vi "Project Program.vi"() -> ()   [LabVIEW 2023]
uses:
  <vilib>/Utility/file.llb/Write Delimited Spreadsheet (string).vi
  <vilib>/Utility/file.llb/Write Delimited Spreadsheet (DBL).vi
  <vilib>/express/express arith-compare/Formula/XNode/ExpressFormulaBlockNode.xnode
panel:
  out "Temp":dbl=4.0
  out "IG Array.":dbl[](array[numeric])=[-6.82e-13, -5e-13, -4.42e-13, -8.34e-13, -4.21e-13, -3.68e-13, -5.57e-13, -6.42e-13, -4.64e-13, -4e-13, -6.61e-13, -7.43e-13, -3.88e-13, -2.58e-13, -5.2e-13, -3.59e-13, -5.4e-13, -3.47e-13, -7.65e-13, -4.69e-13, -3.96e-13, -4.05e-13, -9.33e-13, -5.96e-13, -7.48e-13, -9.11e-13, -8.06e-13, -6.45e-13, -4.48e-13, -5.19e-13, -7.58e-13, -7.76e-13, -5.16e-13, -3.9e-13, -3.24e-13, -6.43e-13, -6.17e-13, -6.27e-13, -4.35e-13, -4.04e-13, -5.04e-13, -8.21e-13, -4.73e-13, -4.57e-13, -2.88e-13, -5.66e-13, -4.46e-13, -7.34e-13, -3.11e-13, -5.05e-13, -6.99e-13, -8.36e-13, -7.42e-13, -5.52e-13, -5.7e-13, -4.36e-13, -4.75e-13, -7.06e-13, -7.55e-13, -6.53e-13, -6.56e-13, -4.28e-13, -7.24e-13, -6.36e-13, -4.42e-13, -5.4e-13, -9.54e-13, -3.54e-13, -3.44e-13, -5.99e-13, -4e-13, -6.34e-13, -4.03e-13, -8.94e-13, -6.36e-13, -7.24e-13, -4.01e-13, -5.45e-13, -8.2e-13, -6.39e-13, -7.02e-13, -7.71e-13, -2.97e-13, -2.58e-13, -2.32e-13, -4.29e-13, -2.53e-13, -6.84e-13, -2.11e-13, -3.25e-13, -7.94e-13, -8.62e-13, -7.69e-13, -3.49e-13, -7.07e-13, -9.35e-13, -7.59e-13, -8.18e-13, -1.75e-13, -5.32e-13, -6.85e-13, -6.03e-13, -5.71e-13, -3.91e-13, -3.83e-13, -5.11e-13, -6.19e-13, -8.05e-13, -5.87e-13, -1.199e-12, -1.69e-13, -6.21e-13, -7.91e-13, -7.88e-13, -8.19e-13, -2.8e-13, -6e-13, -2.05e-13, -7.35e-13, -9.14e-13, -5.56e-13, -6.15e-13, -4.42e-13, -3.57e-13, -6.11e-13, -6.95e-13, -3.19e-13, -3.43e-13, -1.41e-13, -6.66e-13, -8.3e-13, -2.95e-13, -2.83e-13, -3.68e-13, -5.57e-13, -6.58e-13, -9.05e-13, -5.9e-13, -3.75e-13, -5.67e-13, 6.3e-14, -6.42e-13, -5.47e-13, -5.51e-13, -2.83e-13, -2.68e-13, -1.89e-13, -4.14e-13, -1.48e-13, -2.35e-13, -5.91e-13, -4.54e-13, -3.95e-13, -1.6e-13, -3.92e-13, -2.8e-13, -5.4e-13, -5.74e-13, -4.24e-13, -1.97e-13, -3.02e-13, -7.59e-13, -3.84e-13, -3.12e-13, -1.53e-13, -5e-13, -2.01e-13, -1.93e-13, -6.54e-13, -7.73e-13, -4.32e-13, -4.13e-13, -5.04e-13, -7.92e-13, -5.26e-13, -7.05e-13, -1.48e-13, -4.35e-13, -5.34e-13, -6.1e-13, -7.07e-13, -5.12e-13, -2.05e-13, -4.81e-13, -5.25e-13, -5.59e-13, -6.02e-13, -6.46e-13, -2.85e-13, -8.37e-13, -5.61e-13, -7.06e-13, -5.7e-13, -6.64e-13, -4.13e-13, -5.68e-13, -3.11e-13, -1.84e-13, -4.02e-13, -7.21e-13, -5.2e-13, 3.29e-13, 2.34e-13, -2.45e-13, -4.14e-13, -3.81e-13, -4.92e-13, -5.75e-13, -2.57e-13, -5.26e-13, -2.99e-13, 4e-15, -2.53e-13, -1.47e-13, -2.6e-14, -4.26e-13, -3.63e-13, -3.29e-13, -5.5e-14, -4.05e-13, -2.06e-13, -1.03e-13, -2.8e-14, -1.05e-13, -2.6e-13, -5.99e-13, 9.7e-14, -4.2e-14, -2.06e-13, -2e-13, -4.16e-13, -2.51e-13, -4e-15, -1.93e-13, -1.86e-13, -5.89e-13, -1.7e-14, -3.82e-13, -3.01e-13, -2.5e-13, -1.57e-13, -8.7e-14, -1.97e-13, -4.72e-13, -2e-15, -6.68e-13, -2.31e-13, -1.02e-13, -4.17e-13, -5.68e-13, -1.14e-13, -4.6e-13, -4.91e-13, -4.63e-13, -2.12e-13, -1.35e-13, -6.95e-13, -1.07e-13, -6.8e-14, -2.6e-13, -6.72e-13, -3.61e-13, -2.45e-13, -1.11e-13, -3.42e-13, -2.84e-13, -1.79e-13, -6.88e-13, -4.74e-13, -5.54e-13, -1.4e-14, -1.15e-13, 3.8e-14, -1.88e-13, -4.68e-13, -1.75e-13, -4.27e-13, -6.58e-13, -3.4e-13, -4.2e-14, -2.68e-13, -6.2e-14, -5.96e-13, -1.68e-13, -4.1e-14, -9.4e-14, -2.8e-13, -3.81e-13, -2.24e-13, -2.86e-13, -4.53e-13, -5.21e-13, -6e-14, -4.08e-13, -2.43e-13, -4.3e-13, -7.7e-14, -3.7e-14, -5.15e-13, -3.27e-13, -3.92e-13, 4.1e-14, 1e-13, -4.77e-13, 1.23e-13, -1.54e-13, 5e-15, -4.27e-13, -5.34e-13, -6.01e-13, -2.12e-13, 3.66e-13, -9.7e-14, -3.61e-13, -1.82e-13, -1.01e-13, -5e-15, -4.18e-13, -3.18e-13, -3.43e-13, -2.39e-13, -4.5e-14, -2e-14, -3.4e-13, -2.26e-13, -7.2e-14, -1.1e-13, 1.21e-13, -1.32e-13, -2.78e-13, -2.48e-13, -1.78e-13, 4e-14, -2.05e-13, -2.36e-13, -2.02e-13, -9.2e-14, -2.21e-13, -5.1e-14, -4.32e-13, -1.25e-13, -2.8e-13, -2.2e-13, -3.37e-13, -2.31e-13, -7.8e-14, -2.37e-13, -4.72e-13, 4.3e-14, -7.2e-14, 5.4e-14, 6.6e-14, -4.5e-13, -1.78e-13, -2.78e-13, -1.67e-13, -3.97e-13, -9e-14, -7.2e-14, -4.35e-13, -1.42e-13, -2.21e-13, -2.98e-13, -8.3e-14, -1.71e-13, -3.7e-13, -2.32e-13, -3.63e-13, -3.13e-13, -2.81e-13, -5e-15, -1.9e-13, -3.68e-13, -2.52e-13, -6.7e-14, -1.79e-13, -3e-14, 1.81e-13, -1.51e-13, 1.6e-14, -7e-14, -2.77e-13, -2e-13, -2.96e-13, 1.24e-13, 8.3e-14, -1.71e-13, -4.7e-14, -2.69e-13, 4e-14, -1.82e-13, -3.15e-13, -4.22e-13, -1.56e-13, -3.44e-13, -2.46e-13, -3.44e-13, -3.79e-13, -3.57e-13, -1.4e-14, 5.4e-14, -1.02e-13, 5.84e-13, -1.7e-14, 4e-15, -2.38e-13, -1.91e-13, -7.6e-14, 1.88e-13, 5.3e-14, 1.06e-13, -8.1e-14, 3.29e-13, 7.4e-14, 2.3e-14, 8.1e-14, -5.2e-14, 1.75e-13, -1.05e-13, -1.62e-13, -1.52e-13, -1.37e-13, 2.83e-13, -2.01e-13, 1.55e-13, -2.28e-13, -9e-14, -1.08e-13, -2.68e-13, -7.6e-14, 6.4e-14, 4.9e-14, -1.12e-13, -9.3e-14, 2.9e-13, 2e-13, 3.19e-13, 1.24e-13, 1.35e-13, -1.31e-13, -1.18e-13, 0.0, 3.9e-14, 1.96e-13, -2.89e-13, 7.3e-14, 5.7e-14, 1.58e-13, -1.82e-13, -6.4e-14, -2.97e-13, -3.8e-14, 3.21e-13, 1.44e-13, 3.3e-14, -1.25e-13, -1.78e-13, 2.63e-13, 1.3e-13, 1.5e-14, 7.4e-14, 1.04e-13, 7e-14, 6.7e-14, -1.85e-13, 7.4e-14, 2.66e-13, 3.1e-14, 1.27e-13, -2.9e-14, -1.63e-13, 3.25e-13, 2.92e-13, 4.5e-14, -1.53e-13, 2.76e-13, 2.64e-13, -1.45e-13, -1.78e-13, 1.8e-14, 1.59e-13, 2.41e-13, -2.25e-13, 2.67e-13, -1.4e-14, 4.3e-14, 1.49e-13, -1.23e-13, -3.61e-13, -7.8e-14, 4.8e-14, 1.85e-13, -3.45e-13, 1.58e-13, -3.05e-13, 8.2e-14, 1.84e-13, 6.8e-14, -1.82e-13, 1.04e-13, -1.64e-13, 8.5e-14, -1.8e-13, 9.8e-14, -5e-14, 2.3e-14, -2.07e-13, -9.1e-14, -1.71e-13, -1.3e-14, 6.2e-14, 1.04e-13, -1.34e-13, 9.7e-14, 9.8e-14, -4.4e-14, 2.74e-13, -1.38e-13, -1.16e-13, 2.6e-14, -1.46e-13, -1.14e-13, -5.3e-14, 3.2e-14, 1.7e-14, 2.35e-13, 2.64e-13, -1.7e-14, 5.9e-14, -2.23e-13, -2.5e-14, 6e-14, 1.19e-13, 1.61e-13, 6.3e-14, 2.59e-13, 1.94e-13, 2.47e-13, 1.37e-13, -3.06e-13, -2.38e-13, 2.05e-13, -9.9e-14, 1.1e-14, 1.48e-13, 5.8e-14, 4.4e-14, -1.4e-13, 2.7e-14, -3.39e-13, -2.75e-13, -2.58e-13, -3.37e-13, -7.4e-14, 2.24e-13, 1.9e-14, 3e-14, 2.66e-13, 2.16e-13, 1.33e-13, 6.4e-14, -9.8e-14, -2.48e-13, 1.89e-13, 2.8e-13, 1.88e-13, -2.83e-13, -1.29e-13, -6.8e-14, -3.9e-14, -3e-14, 3.4e-14, 2.08e-13, 2.48e-13, -2.29e-13, -3.13e-13, 9.9e-14, 1.1e-14, 1.71e-13, -1.38e-13, -5.1e-14, 1.75e-13, 1.46e-13, 1.97e-13, -1.43e-13, -8.2e-14, -1.7e-13, 4.1e-14, -1.1e-14, 2.3e-14, -5e-14, -1.42e-13, 3e-15, -2.88e-13, 3.02e-13, -2.4e-14, 2.99e-13, 2.82e-13, 4.16e-13, -1e-14, 6.67e-13, 2e-15, -9.7e-14, 5.35e-13, 3.82e-13, 6.95e-13, 2e-14, 9.2e-14, -1.6e-14, 5.21e-13, 4.68e-13, 1.51e-13, 2.8e-14, 2.17e-13, 3.9e-14, 4.61e-13, 5.25e-13, 2.57e-13, 1.68e-13, 3.19e-13, 1.92e-13, -4e-14, 2.56e-13, 4.05e-13, 1.19e-13, 4.26e-13, 4.39e-13, 4.51e-13, 4.5e-14, 3.61e-13, 2.33e-13, 2.6e-14, 2.97e-13, 1.83e-13, 2.1e-14, 3.82e-13, -4.9e-14, 1.53e-13, -7.1e-14, 5.3e-13, 3.78e-13, -5.1e-14, 3.25e-13, 1.52e-13, 1.09e-13, 1.16e-13, 4.7e-13, 2.93e-13, 3.92e-13, -1.33e-13, 3.44e-13, 4.93e-13, 9.6e-14, -1.5e-14, 1.22e-13, 7.8e-14, 3.6e-13, 5.5e-14, 4.16e-13, 3.8e-14, 2.65e-13, 6.14e-13, 3.3e-13, 5.13e-13, 3.59e-13, 6.7e-14, 5.2e-14, 5.62e-13, 5.22e-13, -7.5e-14, -2.4e-14, 2.24e-13, 3.88e-13, 9e-15, 5.14e-13, -2.2e-14, 8e-14, -6e-15, 4.51e-13, 2.81e-13, -1.61e-13, 1.89e-13, -9e-15, 4.4e-13, 1.46e-13, 2.23e-13, 5.7e-14, 6.28e-13, 3.3e-13, 3.9e-14, 1.08e-13, 4.48e-13, -4.6e-14, 3.47e-13, 1.91e-13, 4.28e-13, 8.8e-14, 4.49e-13, 3.93e-13, 3.5e-13, 3.79e-13, -1e-15, 5e-13, 3.85e-13, -1.2e-14, 4.47e-13, 5.7e-14, 4.27e-13, 5.31e-13, 4.09e-13, 4.53e-13, 9.7e-14, 8e-14, -1.24e-13, 3.3e-13, -9e-15, 2.4e-13, 3.95e-13, 2.18e-13, 3.31e-13, 1.09e-13, 4.33e-13, 8.7e-14, 2.95e-13, 3.41e-13, -1.28e-13, -7.1e-14, 1.058e-12, 3.33e-13, 2.88e-13, -3.6e-14, 2.85e-13, 3.72e-13, -2.5e-14, 4.76e-13, 2.36e-13, 4.69e-13, 3.91e-13, 7.7e-14, 2.27e-13, 8.4e-14, 4.01e-13, 3.55e-13, 2.51e-13, -1.57e-13, 4.06e-13, 3.2e-13, 3.88e-13, 1.74e-13, 4.69e-13, -1.39e-13, 1.3e-14, 4.32e-13, 3.7e-14, 4.77e-13, -2.19e-13, 2.78e-13, 9.1e-14, -5.2e-14, -7.8e-14, 4.01e-13, 5.8e-14, 3.88e-13, 3.37e-13, 2.64e-13, 4.82e-13, 1.07e-13, 4.48e-13, -9.7e-14, 1.21e-13, 3.87e-13, 2.38e-13, 2.76e-13, 4.55e-13, 1.38e-13, 3.06e-13, 1.53e-13, 2.4e-14, 2.9e-13, 1.5e-13, 4.51e-13, 2.21e-13, -1e-15, -5e-14, 2.12e-13, 3.6e-13, 6.9e-14, 2.66e-13, 3.83e-13, -5e-15, 1.39e-13, 1.24e-13, 2.55e-13, 3.51e-13, 1.23e-13, 3.45e-13, 1.29e-13, 1.58e-13, 2.38e-13, 1.23e-13, 4.27e-13, 2.43e-13, 9e-15, 8.6e-14, 7.38e-13, 5.06e-13, 4.28e-13, 7.03e-13, 6.12e-13, 1.47e-13, 1.8e-13, 3.82e-13, 2.45e-13, 2.26e-13, -1.47e-13, 6.06e-13, 2.23e-13, 5.36e-13, 3.34e-13, 3.8e-14, 5.08e-13, 2.49e-13, 2.5e-14, 2.81e-13, 3.98e-13, 2.51e-13, 3.48e-13, 5.39e-13, 6e-13, 3.9e-13, 2.45e-13, 4.17e-13, 6.93e-13, 2.32e-13, 2.78e-13, 6.19e-13, 4.87e-13, 3.68e-13, 6.8e-13, 1.81e-13, 1.82e-13, 3.63e-13, 1.46e-13, 4.6e-13, 4.01e-13, 6.71e-13, 5.98e-13, 4.98e-13, 3.95e-13, 2.33e-13, 4.23e-13, 1.76e-13, 1.79e-13, 4.5e-13, 5.38e-13, 1.06e-13, 4.37e-13, 3.52e-13, 2.38e-13, 5.36e-13, 1.69e-13, 2.1e-13, 6.3e-14, 1.06e-13, 3.98e-13, 1.45e-13, 1.69e-13, 3.27e-13, 6.04e-13, 2.29e-13, 6.07e-13, 4.02e-13, 3.86e-13, 2.03e-13, 6.1e-14, 1.34e-13, 5.67e-13, 3.62e-13, 1.01e-13, 4.68e-13, 6.14e-13, 1.67e-13, 2.98e-13, 2.57e-13, 3.43e-13, 5.74e-13, 1.14e-13, 3.19e-13, 2.06e-13, 4.41e-13, 4.75e-13, 5.9e-14, 1.61e-13, 4.51e-13, 4.81e-13, 4.93e-13, 1.25e-13, 5.25e-13, 2.43e-13, 3.1e-14, 5.47e-13, 5.5e-13, 3.22e-13, 2.07e-13, 1.09e-13, 2.1e-13, 5.02e-13, 1.8e-13, 7.39e-13, 7.08e-13, 6.59e-13, 1.48e-13, 6.28e-13, 6.14e-13, 4.39e-13, 4.18e-13, 4.09e-13, 3.93e-13, -4e-14, 5.1e-13, 3.35e-13, 6.31e-13, 3.03e-13, 6.7e-13, 2.6e-13, 2.84e-13, -6.37e-13, 7.55e-13, 4.6e-13, 6.32e-13, 4.21e-13, 4.58e-13, 4.74e-13, 6.53e-13, 2.34e-13, 4.7e-13, 4.8e-14, 3.43e-13, 5.53e-13, 4.41e-13, 3.05e-13, 3.93e-13, 5.99e-13, 5.14e-13, 4.48e-13, 6.15e-13, 5.84e-13, 8.5e-14, 1.12e-13, 8.7e-14, 4.24e-13, 4.25e-13, 1.44e-13, 1.13e-13, 6.66e-13, 3.59e-13, 4.49e-13, 4.12e-13, 4.91e-13, -9.1e-14, -1.03e-13, -1.45e-13, 3.54e-13, 3.62e-13, 2.3e-14, 1.96e-13, 8.67e-13, 1.45e-13, 4.61e-13, 4.26e-13, 3.17e-13, 5.2e-13, 1.48e-13, 2.17e-13, 5.61e-13, 5.29e-13, 7.6e-14, 3.63e-13, 1.38e-13, 8.7e-14, 9.4e-14, 1.53e-13, 2.13e-13, 1.67e-13, 5.7e-14, 4.7e-13, 6.26e-13, 2.01e-13, 4.63e-13, 5.33e-13, 5.61e-13, 2.93e-13, 3.24e-13, 6.8e-14, 3.09e-13, 1.24e-13, 4.98e-13, 3.88e-13, 1.31e-13, 5.47e-13, 6.1e-14, 4.6e-13, 1.77e-13, 4.94e-13, 3.46e-13]
  out "IS Array.":dbl[](array[numeric])=[1.45e-12, 5e-14, -2.1e-13, -2.86e-12, 9.3e-13, 7.8e-13, -9.4e-13, -3e-14, -1.04e-12, 1.2e-13, -6.7e-13, -7.7e-13, 4.2e-13, 5.3e-13, 1.5e-13, -1e-14, 3.9e-13, 5.4e-13, -2e-14, 1.2e-13, -5e-13, 2.4e-13, -3.6e-13, -3e-13, 7.3e-13, -5.6e-13, -9e-14, 3e-13, 3.7e-13, -1.3e-13, 4.6e-13, 4.7e-13, -1.03e-12, 2e-13, 1.4e-13, 5e-14, 4.3e-13, 5e-14, 6e-14, 3.6e-13, 9e-14, -4.6e-13, -7e-14, -5.5e-13, 2.5e-13, 2.3e-13, 3.1e-13, 2.9e-13, 4.1e-13, -9e-14, -5e-14, -1.17e-12, 1.8e-13, 1.5e-13, -5.4e-13, 1.2e-13, 1e-14, -2.7e-13, -5e-13, 1.8e-13, -7.2e-13, -7.6e-13, 3.9e-13, -1.03e-12, -4.8e-13, -5.5e-13, -1.14e-12, -4.4e-13, -7.3e-13, -1.5e-12, -1.03e-12, -1.43e-12, -1.35e-12, -1.04e-12, -1.06e-12, -1.12e-12, -1.2e-12, -4e-13, -3.8e-13, -5.7e-13, 4.8e-13, -3e-14, 3.5e-13, 2e-14, -2.4e-13, 1.3e-13, 4.9e-13, -5.3e-13, 5.2e-13, -1e-13, 3e-13, -8.4e-13, -7.5e-13, -2.4e-13, 3.1e-13, -1.29e-12, -1.37e-12, 4.6e-13, 2.8e-13, 1.9e-13, 2e-13, -6.5e-13, -1.09e-12, -1.12e-12, -1.2e-12, -8.9e-13, -1.76e-12, -1.28e-12, -1.43e-12, -3.13e-12, 3.8e-13, -1.67e-12, -1.88e-12, -1.91e-12, -2.11e-12, -1.44e-12, -2.2e-12, -1.79e-12, -1.62e-12, -1.01e-12, -1.69e-12, -2.03e-12, -8.3e-13, -1.36e-12, -1.41e-12, -1.72e-12, -1.97e-12, -2.05e-12, -1.01e-12, -2.14e-12, -2.65e-12, -1.98e-12, -2.07e-12, -9.2e-13, -1.45e-12, -2.15e-12, -1.33e-12, -1.51e-12, -7.2e-13, -1.03e-12, -5.9e-13, -2.3e-13, -7e-13, -1.83e-12, -1.13e-12, -1.42e-12, -6.9e-13, -1.17e-12, -1.28e-12, -1.22e-12, -9.1e-13, -1.49e-12, -1.2e-12, -1e-12, -1.24e-12, -1.27e-12, -1.77e-12, -1.27e-12, -1.71e-12, -2.68e-12, -2.83e-12, -2.35e-12, -2.67e-12, -1.1e-12, -1.49e-12, -2.12e-12, -2.13e-12, -3.07e-12, -2.63e-12, -3.09e-12, -2.87e-12, -2.45e-12, -1.91e-12, -2.45e-12, -2e-12, -1.09e-12, -1.32e-12, -1.8e-12, -8.9e-13, -2.76e-12, -1.52e-12, -2e-12, -1.19e-12, -2.22e-12, -1.11e-12, -2.47e-12, -1.74e-12, -2.4e-12, -2.69e-12, -2.77e-12, -1.03e-12, -1.99e-12, -1.61e-12, -2.42e-12, -1.35e-12, -2.7e-12, -1.49e-12, -1.34e-12, -1.62e-12, -1.27e-12, -2.73e-12, 2.73e-12, 1.57e-12, 6e-13, -1.7e-13, -1.25e-12, -1.8e-13, -1.53e-12, -1.17e-12, -1.52e-12, -1.32e-12, -3.7e-13, -1.58e-12, -8.7e-13, -2.08e-12, -1.41e-12, -4.6e-13, -9.8e-13, 2e-14, -3.7e-13, -1.21e-12, -2.14e-12, -9.2e-13, -1.96e-12, -6.6e-13, -2.27e-12, -1.8e-12, -5.2e-13, -3.9e-13, -6.2e-13, -5.1e-13, -1.7e-12, -6.1e-13, -1.35e-12, -1.68e-12, -1.87e-12, -1.02e-12, -1.17e-12, -1.43e-12, -1.5e-13, -2.05e-12, -1.61e-12, -8.4e-13, -1.7e-13, -1.1e-12, -2.12e-12, -1.15e-12, -2.03e-12, -1.05e-12, 3.6e-13, -1.4e-12, -5.7e-13, -4.3e-13, -9.1e-13, -1.05e-12, -1.2e-12, -1.54e-12, -1.47e-12, -2.12e-12, -2.02e-12, -1.78e-12, -1.94e-12, -1.49e-12, -6.8e-13, -1.76e-12, -1.68e-12, -1.74e-12, -2.18e-12, -1.77e-12, -1.99e-12, -1.01e-12, -9e-13, -1.56e-12, -1.66e-12, -8.2e-13, -1.85e-12, -1.71e-12, -2.03e-12, -1.81e-12, -1.08e-12, -1.42e-12, -9e-13, -1.94e-12, -1.74e-12, -6.2e-13, -5.2e-13, -1.12e-12, -1.41e-12, -2.36e-12, -8.7e-13, -1.65e-12, -2.5e-13, -1.97e-12, -1.47e-12, -2e-13, -1.95e-12, -1.82e-12, -1.73e-12, -2.13e-12, -1.22e-12, -1.94e-12, -4.5e-13, -4.5e-13, -4.7e-13, -1.05e-12, -3e-13, -6.3e-13, -8.2e-13, -5.8e-13, -1.29e-12, -6e-13, -9.4e-13, -7.8e-13, -9.6e-13, -8.4e-13, -7.2e-13, -5.4e-13, -8.1e-13, -1.47e-12, -1.11e-12, -5.8e-13, -6.9e-13, -8.1e-13, -4.6e-13, -1.08e-12, -6.7e-13, -8.4e-13, -8.1e-13, -1.14e-12, -9.7e-13, -2.17e-12, -8.8e-13, -8.1e-13, -1.09e-12, -1.23e-12, -1.62e-12, -4.9e-13, -1.17e-12, -8.7e-13, -1.3e-12, -9e-13, -7.4e-13, -1.31e-12, -1.59e-12, -5.1e-13, -9.8e-13, -1.48e-12, -1.61e-12, -9.8e-13, -1.25e-12, -8e-13, -1.01e-12, -1.05e-12, -1.75e-12, -1.6e-12, -1.05e-12, -2.05e-12, -2.24e-12, -2.6e-12, -2.1e-12, -1.18e-12, -4.8e-13, -2.52e-12, -2.55e-12, -2.45e-12, -1.33e-12, -2.5e-12, -1.91e-12, -1.81e-12, -2.13e-12, -2.08e-12, -2.67e-12, -2.15e-12, -1.98e-12, -1.59e-12, -1.51e-12, -1.56e-12, -1.55e-12, -1.62e-12, -1.68e-12, -1.81e-12, -1.44e-12, -1.49e-12, -2.74e-12, -1.57e-12, -1.76e-12, -1.65e-12, -2.05e-12, -2.34e-12, -1.89e-12, -1.99e-12, -3.07e-12, -1.87e-12, -1.98e-12, -2.8e-12, -2.47e-12, -2.88e-12, -3.02e-12, -2.54e-12, -2.61e-12, -2.22e-12, -2.11e-12, 1.84e-12, -4.527e-11, -7.62e-11, -9.765e-11, -1.1208e-10, -1.2067e-10, -1.2761e-10, -1.3257e-10, -1.3455e-10, -1.364e-10, -1.3748e-10, -1.3822e-10, -1.3924e-10, -1.3974e-10, -1.399e-10, -1.403e-10, -1.4069e-10, -1.4036e-10, -1.4053e-10, -1.4086e-10, -1.4054e-10, -1.4093e-10, -1.4046e-10, -1.4098e-10, -1.4084e-10, -1.4118e-10, -1.4114e-10, -1.4059e-10, -1.4101e-10, -1.4082e-10, -1.4116e-10, -1.4106e-10, -1.4098e-10, -1.4065e-10, -1.4071e-10, -1.4109e-10, -1.4122e-10, -1.4107e-10, -1.4161e-10, -1.4171e-10, -1.4186e-10, -1.424e-10, -1.4226e-10, -1.4196e-10, -1.4141e-10, -1.4259e-10, -1.4121e-10, -1.4201e-10, -1.4247e-10, -1.4264e-10, -1.4237e-10, -1.4132e-10, -1.4167e-10, -1.4116e-10, -1.4199e-10, -1.4121e-10, -1.416e-10, -1.4155e-10, -1.4222e-10, -1.4124e-10, -1.4118e-10, -1.4173e-10, -1.4239e-10, -1.4143e-10, -1.4161e-10, -1.4134e-10, -1.419e-10, -1.416e-10, -1.4148e-10, -1.4183e-10, -1.4174e-10, -1.4195e-10, -1.4167e-10, -1.4165e-10, -1.4197e-10, -1.4185e-10, -1.4234e-10, -1.4281e-10, -1.4356e-10, -1.4293e-10, -1.4324e-10, -1.4201e-10, -1.421e-10, -1.4332e-10, -1.4357e-10, -1.4387e-10, -1.4283e-10, -1.4343e-10, -1.4313e-10, -1.4341e-10, -1.4369e-10, -1.4388e-10, -1.4359e-10, -1.4282e-10, -1.4388e-10, -1.4289e-10, -1.4361e-10, -1.4297e-10, -1.4366e-10, -1.4404e-10, -1.4348e-10, -1.4383e-10, -1.4245e-10, -1.4235e-10, -1.4395e-10, -1.4377e-10, -1.4375e-10, -1.4322e-10, -1.4311e-10, -1.4396e-10, -1.4379e-10, -1.4377e-10, -1.4429e-10, -1.427e-10, -1.4285e-10, -1.4362e-10, -1.4389e-10, -1.4401e-10, -1.4402e-10, -1.4402e-10, -1.4433e-10, -1.4377e-10, -1.4412e-10, -1.4409e-10, -1.4311e-10, -1.4382e-10, -1.4361e-10, -1.4437e-10, -1.4413e-10, -1.4341e-10, -1.436e-10, -1.4432e-10, -1.444e-10, -1.4404e-10, -1.444e-10, -1.4398e-10, -1.4326e-10, -1.437e-10, -1.4361e-10, -1.4308e-10, -1.4356e-10, -1.4347e-10, -1.4421e-10, -1.4378e-10, -1.4436e-10, -1.4426e-10, -1.4394e-10, -1.4423e-10, -1.4454e-10, -1.4386e-10, -1.4316e-10, -1.4393e-10, -1.4404e-10, -1.4465e-10, -1.4445e-10, -1.4466e-10, -1.4463e-10, -1.4466e-10, -1.4419e-10, -1.4424e-10, -1.4404e-10, -1.4463e-10, -1.4349e-10, -1.4447e-10, -1.4489e-10, -1.4419e-10, -1.4465e-10, -1.4514e-10, -1.4481e-10, -1.4451e-10, -1.4488e-10, -1.448e-10, -1.4505e-10, -1.4492e-10, -1.4527e-10, -1.4411e-10, -1.4463e-10, -1.4465e-10, -1.4487e-10, -1.4545e-10, -1.4418e-10, -1.4441e-10, -1.449e-10, -1.4478e-10, -1.4528e-10, -1.4514e-10, -1.4504e-10, -1.4458e-10, -1.4558e-10, -1.4461e-10, -1.4538e-10, -1.4497e-10, -1.4427e-10, -1.4434e-10, -1.444e-10, -1.4477e-10, -1.4559e-10, -1.448e-10, -1.444e-10, -1.4493e-10, -1.4498e-10, -2.6459e-10, -2.54641e-08, -4.2624e-08, -5.43209e-08, -6.23107e-08, -6.77761e-08, -7.15199e-08, -7.41051e-08, -7.58917e-08, -7.71383e-08, -7.80264e-08, -7.86653e-08, -7.91286e-08, -7.94711e-08, -7.97428e-08, -7.99472e-08, -8.0113e-08, -8.02497e-08, -8.03727e-08, -8.04803e-08, -8.05671e-08, -8.06517e-08, -8.07284e-08, -8.0809e-08, -8.08814e-08, -8.09404e-08, -8.10136e-08, -8.10705e-08, -8.11236e-08, -8.11863e-08, -8.12392e-08, -8.12964e-08, -8.13523e-08, -8.13998e-08, -8.14508e-08, -8.1509e-08, -8.15636e-08, -8.1603e-08, -8.16525e-08, -8.17068e-08, -8.17488e-08, -8.17941e-08, -8.18423e-08, -8.18884e-08, -8.19383e-08, -8.19736e-08, -8.2019e-08, -8.20568e-08, -8.20943e-08, -8.2139e-08, -8.21761e-08, -8.2213e-08, -8.22478e-08, -8.2299e-08, -8.23299e-08, -8.23703e-08, -8.24058e-08, -8.24431e-08, -8.24765e-08, -8.25173e-08, -8.25541e-08, -8.25886e-08, -8.26219e-08, -8.26445e-08, -8.26754e-08, -8.27119e-08, -8.27546e-08, -8.27777e-08, -8.28106e-08, -8.28426e-08, -8.28771e-08, -8.29038e-08, -8.29457e-08, -8.29715e-08, -8.29998e-08, -8.30274e-08, -8.30638e-08, -8.30896e-08, -8.31279e-08, -8.31525e-08, -8.31749e-08, -8.32069e-08, -8.32449e-08, -8.32765e-08, -8.32978e-08, -8.33339e-08, -8.33645e-08, -8.33938e-08, -8.34173e-08, -8.34608e-08, -8.34732e-08, -8.35048e-08, -8.35329e-08, -8.35541e-08, -8.35798e-08, -8.36099e-08, -8.36382e-08, -8.366e-08, -8.36882e-08, -8.37031e-08, -8.37258e-08, -8.37499e-08, -8.37649e-08, -8.38027e-08, -8.38215e-08, -8.3846e-08, -8.3872e-08, -8.38942e-08, -8.39152e-08, -8.39316e-08, -8.39607e-08, -8.39733e-08, -8.40076e-08, -8.40155e-08, -8.40436e-08, -8.40615e-08, -8.40903e-08, -8.4109e-08, -8.4135e-08, -8.41556e-08, -8.41827e-08, -8.4208e-08, -8.42384e-08, -8.42532e-08, -8.42769e-08, -8.43021e-08, -8.43133e-08, -8.43359e-08, -8.43572e-08, -8.43847e-08, -8.44055e-08, -8.44316e-08, -8.44513e-08, -8.44674e-08, -8.44937e-08, -8.4516e-08, -8.45346e-08, -8.45524e-08, -8.45858e-08, -8.46132e-08, -8.46367e-08, -8.46515e-08, -8.46666e-08, -8.46868e-08, -8.47085e-08, -8.47332e-08, -8.47643e-08, -8.47916e-08, -8.48143e-08, -8.48324e-08, -8.48522e-08, -8.48681e-08, -8.48935e-08, -8.49121e-08, -8.49398e-08, -8.49516e-08, -8.4972e-08, -8.49934e-08, -8.50111e-08, -8.50233e-08, -8.50461e-08, -8.5069e-08, -8.50947e-08, -8.51109e-08, -8.51288e-08, -8.51463e-08, -8.51632e-08, -8.51915e-08, -8.52002e-08, -8.52191e-08, -8.52398e-08, -8.52598e-08, -8.52805e-08, -8.52918e-08, -8.53124e-08, -8.53228e-08, -8.53494e-08, -8.53644e-08, -8.53732e-08, -8.5397e-08, -8.5412e-08, -8.54245e-08, -8.54394e-08, -8.5461e-08, -8.54818e-08, -8.54907e-08, -8.55098e-08, -8.55324e-08, -8.55477e-08, -8.55654e-08, -8.5591e-08, -8.56052e-08, -8.56257e-08, -8.56393e-08, -8.56572e-08, -8.56698e-08, -8.56911e-08, -8.57127e-08, -8.57298e-08, -8.57441e-08, -8.57758e-08, -4.97761e-08, -5.88045e-06, -1.147363e-05, -1.68009e-05, -2.18357e-05, -2.65539e-05, -3.09309e-05, -3.49365e-05, -3.85664e-05, -4.17989e-05, -4.46413e-05, -4.71049e-05, -4.92068e-05, -5.0983e-05, -5.24784e-05, -5.37333e-05, -5.47781e-05, -5.56532e-05, -5.63995e-05, -5.70405e-05, -5.75888e-05, -5.80606e-05, -5.8482e-05, -5.88578e-05, -5.91977e-05, -5.9501e-05, -5.97803e-05, -6.00377e-05, -6.02795e-05, -6.04986e-05, -6.06989e-05, -6.08925e-05, -6.10713e-05, -6.12384e-05, -6.14041e-05, -6.15487e-05, -6.16947e-05, -6.18267e-05, -6.19606e-05, -6.20839e-05, -6.21985e-05, -6.23282e-05, -6.2438e-05, -6.25424e-05, -6.26367e-05, -6.27362e-05, -6.28295e-05, -6.29133e-05, -6.30049e-05, -6.30903e-05, -6.31797e-05, -6.32485e-05, -6.33258e-05, -6.33979e-05, -6.34787e-05, -6.35509e-05, -6.36169e-05, -6.36837e-05, -6.37466e-05, -6.38155e-05, -6.38793e-05, -6.39407e-05, -6.40018e-05, -6.40629e-05, -6.41217e-05, -6.41747e-05, -6.42263e-05, -6.42709e-05, -6.4326e-05, -6.43753e-05, -6.44356e-05, -6.44874e-05, -6.45267e-05, -6.458e-05, -6.46331e-05, -6.46783e-05, -6.47156e-05, -6.47671e-05, -6.48122e-05, -6.48529e-05, -6.49047e-05, -6.49457e-05, -6.49889e-05, -6.50317e-05, -6.50682e-05, -6.51131e-05, -6.51648e-05, -6.52036e-05, -6.52453e-05, -6.52791e-05, -6.53291e-05, -6.53676e-05, -6.54007e-05, -6.54392e-05, -6.54791e-05, -6.5516e-05, -6.55542e-05, -6.55872e-05, -6.56284e-05, -6.566e-05, -6.56994e-05, -6.57288e-05, -6.57688e-05, -6.58028e-05, -6.58443e-05, -6.5879e-05, -6.59121e-05, -6.59415e-05, -6.59762e-05, -6.6e-05, -6.60366e-05, -6.60663e-05, -6.61075e-05, -6.61445e-05, -6.6176e-05, -6.62067e-05, -6.62385e-05, -6.62691e-05, -6.62982e-05, -6.63349e-05, -6.63693e-05, -6.63999e-05, -6.64246e-05, -6.64516e-05, -6.64878e-05, -6.65199e-05, -6.65526e-05, -6.65745e-05, -6.66061e-05, -6.664e-05, -6.66603e-05, -6.66943e-05, -6.67256e-05, -6.67537e-05, -6.67805e-05, -6.68215e-05, -6.6844e-05, -6.68755e-05, -6.69059e-05, -6.69304e-05, -6.69563e-05, -6.69813e-05, -6.70104e-05, -6.70309e-05, -6.7059e-05, -6.70859e-05, -6.71203e-05, -6.71418e-05, -6.71594e-05, -6.71947e-05, -6.7212e-05, -6.72355e-05, -6.72665e-05, -6.72848e-05, -6.73151e-05, -6.73465e-05, -6.73694e-05, -6.73947e-05, -6.7425e-05, -6.74492e-05, -6.74753e-05, -6.75045e-05, -6.75358e-05, -6.75609e-05, -6.75801e-05, -6.75993e-05, -6.76316e-05, -6.76481e-05, -6.76748e-05, -6.76966e-05, -6.7725e-05, -6.77455e-05, -6.77755e-05, -6.78057e-05, -6.78222e-05, -6.78487e-05, -6.78797e-05, -6.78995e-05, -6.7927e-05, -6.79571e-05, -6.79734e-05, -6.79928e-05, -6.80149e-05, -6.80402e-05, -6.80675e-05, -6.8096e-05, -6.81133e-05, -6.81446e-05, -6.81735e-05, -6.81888e-05, -6.82085e-05, -6.82342e-05, -6.82538e-05, -6.82817e-05, -6.83089e-05, -6.83291e-05, -6.83409e-05, -6.83623e-05, -6.83832e-05, -6.83993e-05, -6.84278e-05]
  out "Gate current":dbl=3.46e-13 format="%#_13g"
  out "Source current":dbl=-6.84278e-05 format="%#_13g"
  out "d'ID":dbl=7.673582799462006e-08
  out "VG Array":dbl[](array[numeric])=[0.0, 0.01, 0.02, 0.03, 0.04, 0.05, 0.060000000000000005, 0.07, 0.08, 0.09, 0.09999999999999999, 0.10999999999999999, 0.11999999999999998, 0.12999999999999998, 0.13999999999999999, 0.15, 0.16, 0.17, 0.18000000000000002, 0.19000000000000003, 0.20000000000000004, 0.21000000000000005, 0.22000000000000006, 0.23000000000000007, 0.24000000000000007, 0.25000000000000006, 0.26000000000000006, 0.2700000000000001, 0.2800000000000001, 0.2900000000000001, 0.3000000000000001, 0.3100000000000001, 0.3200000000000001, 0.3300000000000001, 0.34000000000000014, 0.35000000000000014, 0.36000000000000015, 0.37000000000000016, 0.38000000000000017, 0.3900000000000002, 0.4000000000000002, 0.4100000000000002, 0.4200000000000002, 0.4300000000000002, 0.4400000000000002, 0.45000000000000023, 0.46000000000000024, 0.47000000000000025, 0.48000000000000026, 0.49000000000000027, 0.5000000000000002, 0.5100000000000002, 0.5200000000000002, 0.5300000000000002, 0.5400000000000003, 0.5500000000000003, 0.5600000000000003, 0.5700000000000003, 0.5800000000000003, 0.5900000000000003, 0.6000000000000003, 0.6100000000000003, 0.6200000000000003, 0.6300000000000003, 0.6400000000000003, 0.6500000000000004, 0.6600000000000004, 0.6700000000000004, 0.6800000000000004, 0.6900000000000004, 0.7000000000000004, 0.7100000000000004, 0.7200000000000004, 0.7300000000000004, 0.7400000000000004, 0.7500000000000004, 0.7600000000000005, 0.7700000000000005, 0.7800000000000005, 0.7900000000000005, 0.8000000000000005, 0.8100000000000005, 0.8200000000000005, 0.8300000000000005, 0.8400000000000005, 0.8500000000000005, 0.8600000000000005, 0.8700000000000006, 0.8800000000000006, 0.8900000000000006, 0.9000000000000006, 0.9100000000000006, 0.9200000000000006, 0.9300000000000006, 0.9400000000000006, 0.9500000000000006, 0.9600000000000006, 0.9700000000000006, 0.9800000000000006, 0.9900000000000007, 1.0000000000000007, 1.0100000000000007, 1.0200000000000007, 1.0300000000000007, 1.0400000000000007, 1.0500000000000007, 1.0600000000000007, 1.0700000000000007, 1.0800000000000007, 1.0900000000000007, 1.1000000000000008, 1.1100000000000008, 1.1200000000000008, 1.1300000000000008, 1.1400000000000008, 1.1500000000000008, 1.1600000000000008, 1.1700000000000008, 1.1800000000000008, 1.1900000000000008, 1.2000000000000008, 1.2100000000000009, 1.2200000000000009, 1.2300000000000009, 1.2400000000000009, 1.2500000000000009, 1.260000000000001, 1.270000000000001, 1.280000000000001, 1.290000000000001, 1.300000000000001, 1.310000000000001, 1.320000000000001, 1.330000000000001, 1.340000000000001, 1.350000000000001, 1.360000000000001, 1.370000000000001, 1.380000000000001, 1.390000000000001, 1.400000000000001, 1.410000000000001, 1.420000000000001, 1.430000000000001, 1.440000000000001, 1.450000000000001, 1.460000000000001, 1.470000000000001, 1.480000000000001, 1.490000000000001, 1.500000000000001, 1.5100000000000011, 1.5200000000000011, 1.5300000000000011, 1.5400000000000011, 1.5500000000000012, 1.5600000000000012, 1.5700000000000012, 1.5800000000000012, 1.5900000000000012, 1.6000000000000012, 1.6100000000000012, 1.6200000000000012, 1.6300000000000012, 1.6400000000000012, 1.6500000000000012, 1.6600000000000013, 1.6700000000000013, 1.6800000000000013, 1.6900000000000013, 1.7000000000000013, 1.7100000000000013, 1.7200000000000013, 1.7300000000000013, 1.7400000000000013, 1.7500000000000013, 1.7600000000000013, 1.7700000000000014, 1.7800000000000014, 1.7900000000000014, 1.8000000000000014, 1.8100000000000014, 1.8200000000000014, 1.8300000000000014, 1.8400000000000014, 1.8500000000000014, 1.8600000000000014, 1.8700000000000014, 1.8800000000000014, 1.8900000000000015, 1.9000000000000015, 1.9100000000000015, 1.9200000000000015, 1.9300000000000015, 1.9400000000000015, 1.9500000000000015, 1.9600000000000015, 1.9700000000000015, 1.9800000000000015, 1.9900000000000015, 2.0000000000000013, 1.9900000000000013, 1.9800000000000013, 1.9700000000000013, 1.9600000000000013, 1.9500000000000013, 1.9400000000000013, 1.9300000000000013, 1.9200000000000013, 1.9100000000000013, 1.9000000000000012, 1.8900000000000012, 1.8800000000000012, 1.8700000000000012, 1.8600000000000012, 1.8500000000000012, 1.8400000000000012, 1.8300000000000012, 1.8200000000000012, 1.8100000000000012, 1.8000000000000012, 1.7900000000000011, 1.7800000000000011, 1.7700000000000011, 1.7600000000000011, 1.750000000000001, 1.740000000000001, 1.730000000000001, 1.720000000000001, 1.710000000000001, 1.700000000000001, 1.690000000000001, 1.680000000000001, 1.670000000000001, 1.660000000000001, 1.650000000000001, 1.640000000000001, 1.630000000000001, 1.620000000000001, 1.610000000000001, 1.600000000000001, 1.590000000000001, 1.580000000000001, 1.570000000000001, 1.560000000000001, 1.550000000000001, 1.540000000000001, 1.530000000000001, 1.520000000000001, 1.510000000000001, 1.5000000000000009, 1.4900000000000009, 1.4800000000000009, 1.4700000000000009, 1.4600000000000009, 1.4500000000000008, 1.4400000000000008, 1.4300000000000008, 1.4200000000000008, 1.4100000000000008, 1.4000000000000008, 1.3900000000000008, 1.3800000000000008, 1.3700000000000008, 1.3600000000000008, 1.3500000000000008, 1.3400000000000007, 1.3300000000000007, 1.3200000000000007, 1.3100000000000007, 1.3000000000000007, 1.2900000000000007, 1.2800000000000007, 1.2700000000000007, 1.2600000000000007, 1.2500000000000007, 1.2400000000000007, 1.2300000000000006, 1.2200000000000006, 1.2100000000000006, 1.2000000000000006, 1.1900000000000006, 1.1800000000000006, 1.1700000000000006, 1.1600000000000006, 1.1500000000000006, 1.1400000000000006, 1.1300000000000006, 1.1200000000000006, 1.1100000000000005, 1.1000000000000005, 1.0900000000000005, 1.0800000000000005, 1.0700000000000005, 1.0600000000000005, 1.0500000000000005, 1.0400000000000005, 1.0300000000000005, 1.0200000000000005, 1.0100000000000005, 1.0000000000000004, 0.9900000000000004, 0.9800000000000004, 0.9700000000000004, 0.9600000000000004, 0.9500000000000004, 0.9400000000000004, 0.9300000000000004, 0.9200000000000004, 0.9100000000000004, 0.9000000000000004, 0.8900000000000003, 0.8800000000000003, 0.8700000000000003, 0.8600000000000003, 0.8500000000000003, 0.8400000000000003, 0.8300000000000003, 0.8200000000000003, 0.8100000000000003, 0.8000000000000003, 0.7900000000000003, 0.7800000000000002, 0.7700000000000002, 0.7600000000000002, 0.7500000000000002, 0.7400000000000002, 0.7300000000000002, 0.7200000000000002, 0.7100000000000002, 0.7000000000000002, 0.6900000000000002, 0.6800000000000002, 0.6700000000000002, 0.6600000000000001, 0.6500000000000001, 0.6400000000000001, 0.6300000000000001, 0.6200000000000001, 0.6100000000000001, 0.6000000000000001, 0.5900000000000001, 0.5800000000000001, 0.5700000000000001, 0.56, 0.55, 0.54, 0.53, 0.52, 0.51, 0.5, 0.49, 0.48, 0.47, 0.45999999999999996, 0.44999999999999996, 0.43999999999999995, 0.42999999999999994, 0.41999999999999993, 0.4099999999999999, 0.3999999999999999, 0.3899999999999999, 0.3799999999999999, 0.3699999999999999, 0.3599999999999999, 0.34999999999999987, 0.33999999999999986, 0.32999999999999985, 0.31999999999999984, 0.30999999999999983, 0.2999999999999998, 0.2899999999999998, 0.2799999999999998, 0.2699999999999998, 0.2599999999999998, 0.24999999999999978, 0.23999999999999977, 0.22999999999999976, 0.21999999999999975, 0.20999999999999974, 0.19999999999999973, 0.18999999999999972, 0.17999999999999972, 0.1699999999999997, 0.1599999999999997, 0.1499999999999997, 0.13999999999999968, 0.12999999999999967, 0.11999999999999968, 0.10999999999999968, 0.09999999999999969, 0.08999999999999969, 0.0799999999999997, 0.0699999999999997, 0.0599999999999997, 0.0499999999999997, 0.039999999999999696, 0.029999999999999694, 0.01999999999999969, 0.009999999999999691, -3.0878077872387166e-16]
  out "IG Array":dbl[](array[numeric])=[-1.003e-12, -2.13e-13, -1.33e-13, 2.2e-14, 5.1e-14, -2.6e-14, -2.1e-14, 1.53e-13, -1.32e-13, 4.4e-14, 7.9e-14, 1.11e-13, 7.4e-14, -5.3e-14, 9.2e-14, 9.4e-14, -1.59e-13, -2.6e-14, 1.19e-13, -2.3e-14, 1.17e-13, 1.18e-13, 2.8e-14, 3.9e-14, 2.41e-13, 1.51e-13, 2.9e-14, 1.13e-13, 5.5e-14, 1.99e-13, 2.15e-13, 3.03e-13, 2.54e-13, 2.03e-13, 5e-14, 2.97e-13, 2.73e-13, -3.1e-14, 3.9e-14, 1.93e-13, 2.2e-13, -3.1e-14, 3.59e-13, 2.25e-13, 6.3e-14, 3.07e-13, 1.6e-13, 7.3e-14, 6.1e-14, 1.57e-13, 3.31e-13, 1.58e-13, -3.8e-14, 3.5e-14, 3.52e-13, 2.74e-13, 3.33e-13, 3.79e-13, 2.79e-13, 3.66e-13, 6.7e-14, 3.68e-13, 3.82e-13, 3.91e-13, 1.3e-14, 1.12e-13, 3.85e-13, 2.35e-13, 4.56e-13, 3.84e-13, 1.48e-13, 1.59e-13, 2.01e-13, 2.43e-13, 3.99e-13, 7e-14, 3.29e-13, 4.59e-13, 5.9e-14, 1.83e-13, 4.74e-13, 2.79e-13, 5.73e-13, 1.82e-13, 3.37e-13, 2.83e-13, 1.1e-13, 3.39e-13, 2.74e-13, 3.37e-13, 2.75e-13, 4.68e-13, 4.51e-13, 4.4e-13, 7.8e-14, 1.47e-13, 2.04e-13, 3.69e-13, 3.09e-13, 4.2e-13, 5.33e-13, 6.23e-13, 4.3e-13, 3.15e-13, 2.73e-13, 5.33e-13, 2.39e-13, 3.46e-13, 5.35e-13, 2.32e-13, 4.06e-13, 2.58e-13, 5.63e-13, 3.09e-13, 1.88e-13, 6.7e-13, 3.05e-13, 4.22e-13, 7.31e-13, 7.03e-13, 2.57e-13, 5.35e-13, 4.49e-13, 5.53e-13, 3.21e-13, 4.52e-13, 6.15e-13, 4.01e-13, 6.17e-13, 2.33e-13, 4.65e-13, 6.87e-13, 4.71e-13, 5.22e-13, 4.07e-13, 3.87e-13, 3.49e-13, 7.48e-13, 4.14e-13, 3.46e-13, 6.7e-13, 6.03e-13, 4.15e-13, 4.67e-13, 3.69e-13, 3.85e-13, 4.52e-13, 6.27e-13, 4.22e-13, 6.13e-13, 7.24e-13, 3.88e-13, 6.58e-13, 7.23e-13, 5.06e-13, 7.49e-13, 4.49e-13, 4.78e-13, 7.43e-13, 5.4e-13, 5.28e-13, 5.07e-13, 4.95e-13, 7.52e-13, 7.77e-13, 8.45e-13, 8.13e-13, 6.7e-13, 5.13e-13, 7.66e-13, 8.62e-13, 8.5e-13, 5.06e-13, 5.44e-13, 6.46e-13, 5.42e-13, 5.27e-13, 7.14e-13, 6.32e-13, 9.52e-13, 7.34e-13, 5.48e-13, 4.25e-13, 9.12e-13, 9.44e-13, 1.004e-12, 8.99e-13, 9.38e-13, 9.08e-13, 7.99e-13, 5.31e-13, 6.37e-13, 6.4e-13, 5.9e-13, 7.94e-13, 7.35e-13, 5.52e-13, 6.1e-13, 6.1e-13, 1e-12, 9.4e-13, 6.8e-13, 7.38e-13, 5.68e-13, 8.9e-13, 8.42e-13, 7.29e-13, 7.45e-13, 5.27e-13, 8.51e-13, 9.42e-13, 6.34e-13, 4.89e-13, 5.8e-13, 5.68e-13, 5.81e-13, 8.1e-13, 8.33e-13, 6.97e-13, 8.57e-13, 4.9e-13, 8.56e-13, 7.5e-13, 8.46e-13, 7.72e-13, 8.1e-13, 7.38e-13, 7.57e-13, 8.31e-13, 8.35e-13, 7.28e-13, 4.82e-13, 5.65e-13, 8.06e-13, 7.22e-13, 3.87e-13, 8.37e-13, 7.17e-13, 5.65e-13, 5.02e-13, 5.8e-13, 5.3e-13, 7.75e-13, 7.8e-13, 8.39e-13, 4.69e-13, 6.08e-13, 7.13e-13, 4.52e-13, 8.2e-13, 3.63e-13, 4.62e-13, 5.92e-13, 7.1e-13, 7.8e-13, 7.95e-13, 7.33e-13, 4.1e-13, 7.09e-13, 5.52e-13, 5.2e-13, 7.38e-13, 6.62e-13, 7.44e-13, 7.71e-13, 7.47e-13, 4.27e-13, 7.31e-13, 8.27e-13, 2.56e-13, 4.66e-13, 5.42e-13, 7.49e-13, 3.64e-13, 3.13e-13, 7.07e-13, 4.71e-13, 4.63e-13, 2.27e-13, 5e-13, 6.43e-13, 7.41e-13, 5.01e-13, 4.57e-13, 4.85e-13, 2.45e-13, 6.44e-13, 2.88e-13, 5.96e-13, 6.84e-13, 3.48e-13, 6.6e-13, 3.79e-13, 4.28e-13, 6.21e-13, 6.57e-13, 4.12e-13, 5.49e-13, 4.46e-13, 4.01e-13, 4.95e-13, 3.51e-13, 5.29e-13, 3.83e-13, 3.35e-13, 2.82e-13, 4.18e-13, 5.29e-13, 4.21e-13, 3.87e-13, 2.88e-13, 2.48e-13, 3.19e-13, 5.85e-13, 5.03e-13, 4.71e-13, 4.72e-13, 2.32e-13, 2.16e-13, 3.68e-13, 2.66e-13, 5.09e-13, 1.49e-13, 5.32e-13, 4.81e-13, 3.75e-13, 2.1e-14, 5.88e-13, 4.34e-13, -3.1e-14, 3e-13, 2.95e-13, 6.65e-13, 2.39e-13, 4.8e-14, 4.27e-13, 3.07e-13, 2.57e-13, 1.2e-13, 3.83e-13, 3.98e-13, -6e-15, 2.57e-13, 2.44e-13, 6.7e-14, 4.9e-14, 3.63e-13, 1.41e-13, 2.04e-13, 1.71e-13, 4.78e-13, 4.3e-13, 2.66e-13, 2.97e-13, 1.85e-13, -3.63e-13, 7.33e-13, 5.2e-13, 1.91e-13, 1.59e-13, 5.9e-14, 1.49e-13, 3.76e-13, 4.62e-13, 1.62e-13, 3.92e-13, -2.4e-14, 4.7e-14, 3.14e-13, 3.33e-13, 3.62e-13, 4.7e-14, 1.9e-13, 1.01e-13, 7.6e-14, 3.99e-13, 5.1e-14, 1.84e-13, 4.84e-13, 2.87e-13, 1.42e-13, 1.78e-13, 2.36e-13, 4.47e-13, 5e-15, 3.9e-13, 2.1e-14, -1.48e-13, -6.2e-14, -4.42e-13, 1.9e-13, 2.42e-13, -5.6e-14, 4.13e-13, 4.5e-14, -8.1e-14, 4.14e-13, 3.05e-13, 1.2e-13, 8.6e-14, 6.9e-14]
  out "IS Array":dbl[](array[numeric])=[-3.05e-12, -2.69e-12, -2.25e-12, -1.73e-12, -2.58e-12, -1.68e-12, -1.91e-12, -2.35e-12, -2.2e-12, -2.17e-12, -1.53e-12, -1.5e-12, -1.53e-12, -1.72e-12, -1.69e-12, -2.18e-12, -1.89e-12, -1.61e-12, -2.24e-12, -2e-12, -1.4e-12, -1.68e-12, -2e-12, -1.61e-12, -1.95e-12, -1.96e-12, -1.66e-12, -2.52e-12, -2.22e-12, -1.94e-12, -1.74e-12, -2.25e-12, -1.6e-12, -2.11e-12, -1.79e-12, -2.35e-12, -1.82e-12, -1.77e-12, -2.19e-12, -2.36e-12, -1.84e-12, -1.95e-12, -2.01e-12, -1.74e-12, -2.14e-12, -2.44e-12, -3.03e-12, -2.12e-12, -2.73e-12, -2.62e-12, -3.06e-12, -3.34e-12, -2.33e-12, -2.63e-12, -2.52e-12, -3.07e-12, -3.73e-12, -2.64e-12, -3.32e-12, -3.52e-12, -3.27e-12, -4.02e-12, -3.8e-12, -3.93e-12, -3.87e-12, -4.79e-12, -5.38e-12, -4.87e-12, -5.83e-12, -6.07e-12, -6.02e-12, -7.32e-12, -8.37e-12, -7.93e-12, -9.57e-12, -9.61e-12, -1.147e-11, -1.222e-11, -1.28e-11, -1.407e-11, -1.637e-11, -1.764e-11, -1.931e-11, -2.236e-11, -2.384e-11, -2.66e-11, -2.96e-11, -3.412e-11, -3.649e-11, -4.202e-11, -4.569e-11, -5.173e-11, -5.862e-11, -6.585e-11, -7.358e-11, -8.163e-11, -9.157e-11, -1.034e-10, -1.1541e-10, -1.2977e-10, -1.46e-10, -1.6488e-10, -1.8527e-10, -2.0938e-10, -2.3533e-10, -2.6612e-10, -3.0017e-10, -3.3845e-10, -3.825e-10, -4.3155e-10, -4.8869e-10, -5.5105e-10, -6.2387e-10, -7.0596e-10, -7.989e-10, -9.0647e-10, -1.02585e-09, -1.16272e-09, -1.31873e-09, -1.49557e-09, -1.69592e-09, -1.9267e-09, -2.18628e-09, -2.48298e-09, -2.82214e-09, -3.20686e-09, -3.64432e-09, -4.14727e-09, -4.71732e-09, -5.36575e-09, -6.1135e-09, -6.95953e-09, -7.92492e-09, -9.03523e-09, -1.03096e-08, -1.17474e-08, -1.34048e-08, -1.52861e-08, -1.74368e-08, -1.99101e-08, -2.27206e-08, -2.59609e-08, -2.96443e-08, -3.38571e-08, -3.87162e-08, -4.42441e-08, -5.05721e-08, -5.78638e-08, -6.61637e-08, -7.56726e-08, -8.66465e-08, -9.91358e-08, -1.13444e-07, -1.29993e-07, -1.48805e-07, -1.70381e-07, -1.95098e-07, -2.23675e-07, -2.56169e-07, -2.93426e-07, -3.3654e-07, -3.85665e-07, -4.4191e-07, -5.06386e-07, -5.80971e-07, -6.65804e-07, -7.63124e-07, -8.747e-07, -1.00532e-06, -1.15197e-06, -1.32009e-06, -1.51401e-06, -1.735e-06, -1.98773e-06, -2.27717e-06, -2.61122e-06, -2.99041e-06, -3.42463e-06, -3.92074e-06, -4.49243e-06, -5.14086e-06, -5.88208e-06, -6.73369e-06, -7.69862e-06, -8.79905e-06, -1.0051e-05, -1.14876e-05, -1.31091e-05, -1.49681e-05, -1.70607e-05, -1.94385e-05, -2.21546e-05, -2.52107e-05, -2.86911e-05, -3.25866e-05, -3.69845e-05, -4.19878e-05, -4.75705e-05, -5.38488e-05, -6.09423e-05, -6.88302e-05, -6.09323e-05, -5.38268e-05, -4.75543e-05, -4.19667e-05, -3.69625e-05, -3.25571e-05, -2.86604e-05, -2.51859e-05, -2.21348e-05, -1.94186e-05, -1.70418e-05, -1.49505e-05, -1.30938e-05, -1.14735e-05, -1.00374e-05, -8.78612e-06, -7.68625e-06, -6.72398e-06, -5.87236e-06, -5.13316e-06, -4.48483e-06, -3.91407e-06, -3.41868e-06, -2.98588e-06, -2.60643e-06, -2.27323e-06, -1.98439e-06, -1.73204e-06, -1.51162e-06, -1.31788e-06, -1.15013e-06, -1.00381e-06, -8.73468e-07, -7.6201e-07, -6.64943e-07, -5.80205e-07, -5.05792e-07, -4.41324e-07, -3.8513e-07, -3.36094e-07, -2.93083e-07, -2.55826e-07, -2.23378e-07, -1.9484e-07, -1.70175e-07, -1.48641e-07, -1.2985e-07, -1.1333e-07, -9.90297e-08, -8.65633e-08, -7.55941e-08, -6.60876e-08, -5.78044e-08, -5.05172e-08, -4.4193e-08, -3.86796e-08, -3.38276e-08, -2.96199e-08, -2.59408e-08, -2.27028e-08, -1.98945e-08, -1.74241e-08, -1.52736e-08, -1.33958e-08, -1.17382e-08, -1.03011e-08, -9.0433e-09, -7.92087e-09, -6.95577e-09, -6.11071e-09, -5.36383e-09, -4.71414e-09, -4.1458e-09, -3.64248e-09, -3.20521e-09, -2.82087e-09, -2.48173e-09, -2.18529e-09, -1.92492e-09, -1.69474e-09, -1.49485e-09, -1.31823e-09, -1.16229e-09, -1.0261e-09, -9.0564e-10, -7.989e-10, -7.0578e-10, -6.2416e-10, -5.5108e-10, -4.882e-10, -4.3183e-10, -3.8248e-10, -3.3916e-10, -3.0015e-10, -2.6635e-10, -2.3535e-10, -2.0866e-10, -1.8566e-10, -1.6493e-10, -1.4709e-10, -1.3039e-10, -1.1584e-10, -1.0278e-10, -9.164e-11, -8.247e-11, -7.264e-11, -6.498e-11, -5.755e-11, -5.252e-11, -4.626e-11, -4.133e-11, -3.78e-11, -3.39e-11, -2.932e-11, -2.639e-11, -2.496e-11, -2.148e-11, -2.056e-11, -1.75e-11, -1.555e-11, -1.498e-11, -1.305e-11, -1.174e-11, -1.062e-11, -1.072e-11, -9.56e-12, -8.42e-12, -8.87e-12, -7.37e-12, -6.85e-12, -5.64e-12, -5.96e-12, -5.13e-12, -4.33e-12, -4.63e-12, -3.92e-12, -4.57e-12, -4.82e-12, -4.28e-12, -4.09e-12, -3.05e-12, -3.73e-12, -3.92e-12, -3.21e-12, -2.46e-12, -2.44e-12, -3.14e-12, -2.15e-12, -3.47e-12, -2.7e-12, -1.83e-12, -2.03e-12, -2.13e-12, -3.45e-12, -1.16e-12, -2.17e-12, -1.44e-12, -2.82e-12, -2.16e-12, -1.78e-12, -1.75e-12, -2.46e-12, -2.25e-12, -1.84e-12, -2.14e-12, -2.82e-12, -1.58e-12, -2.4e-12, -1.69e-12, -2.05e-12, -2.14e-12, -2.04e-12, -2.28e-12, -1.69e-12, -2.33e-12, -1.56e-12, -1.56e-12, -2.37e-12, -2.27e-12, -2.23e-12, -2.36e-12, -1.47e-12, -2.54e-12, -1.5e-12, -1.78e-12, -2.07e-12, -1.99e-12, -1.77e-12, -9.8e-13, -2.23e-12, -1.61e-12, -1.82e-12, -2.31e-12, -2.17e-12, -1.85e-12, -1.8e-12, -1.92e-12, -2.37e-12, -1.86e-12, -1.4e-12]
  out "ID Array":dbl[](array[numeric])=[3.88e-12, 3.64e-12, 3.18e-12, 2.52e-12, 2.8e-12, 2.68e-12, 2.32e-12, 2.81e-12, 2.16e-12, 2.73e-12, 2.29e-12, 2.34e-12, 2.71e-12, 2.42e-12, 1.98e-12, 1.93e-12, 2.38e-12, 2.17e-12, 1.64e-12, 2.53e-12, 2.2e-12, 2.11e-12, 2.09e-12, 2.42e-12, 2.52e-12, 1.71e-12, 1.77e-12, 2.56e-12, 1.96e-12, 2.56e-12, 2.61e-12, 1.84e-12, 2.01e-12, 1.71e-12, 1.99e-12, 2.59e-12, 1.89e-12, 2.69e-12, 1.66e-12, 2.58e-12, 2.74e-12, 2.52e-12, 2.58e-12, 1.92e-12, 2.63e-12, 2.35e-12, 2.9e-12, 2.07e-12, 3.12e-12, 2.87e-12, 3.01e-12, 2.03e-12, 2.79e-12, 2.4e-12, 3.2e-12, 3.59e-12, 3.05e-12, 3.44e-12, 3.97e-12, 3.12e-12, 3.46e-12, 4.18e-12, 3.64e-12, 4.11e-12, 5.15e-12, 5.3e-12, 5.58e-12, 5.32e-12, 5.57e-12, 6.51e-12, 6.47e-12, 7.66e-12, 8.34e-12, 8.17e-12, 9.3e-12, 1.037e-11, 1.112e-11, 1.146e-11, 1.351e-11, 1.526e-11, 1.586e-11, 1.775e-11, 1.936e-11, 2.186e-11, 2.399e-11, 2.741e-11, 2.955e-11, 3.33e-11, 3.806e-11, 4.096e-11, 4.604e-11, 5.158e-11, 5.795e-11, 6.554e-11, 7.281e-11, 8.134e-11, 9.13e-11, 1.0272e-10, 1.1597e-10, 1.2958e-10, 1.4645e-10, 1.6448e-10, 1.8519e-10, 2.0891e-10, 2.3592e-10, 2.656e-10, 2.9961e-10, 3.3805e-10, 3.8277e-10, 4.3198e-10, 4.8743e-10, 5.5194e-10, 6.24e-10, 7.0694e-10, 7.9931e-10, 9.0539e-10, 1.02644e-09, 1.1625e-09, 1.31809e-09, 1.49425e-09, 1.69599e-09, 1.92587e-09, 2.18703e-09, 2.48255e-09, 2.82254e-09, 3.20734e-09, 3.64559e-09, 4.14722e-09, 4.71621e-09, 5.36629e-09, 6.11357e-09, 6.95969e-09, 7.9255e-09, 9.03598e-09, 1.03146e-08, 1.17517e-08, 1.34102e-08, 1.52907e-08, 1.74415e-08, 1.99148e-08, 2.27251e-08, 2.59674e-08, 2.96495e-08, 3.38627e-08, 3.87214e-08, 4.42515e-08, 5.05772e-08, 5.78698e-08, 6.61666e-08, 7.5681e-08, 8.66554e-08, 9.91418e-08, 1.13458e-07, 1.3e-07, 1.48829e-07, 1.70413e-07, 1.95114e-07, 2.23706e-07, 2.56203e-07, 2.935e-07, 3.36628e-07, 3.8569e-07, 4.42033e-07, 5.065e-07, 5.81044e-07, 6.6598e-07, 7.63283e-07, 8.74861e-07, 1.00629e-06, 1.15287e-06, 1.32094e-06, 1.51491e-06, 1.73584e-06, 1.98839e-06, 2.27792e-06, 2.61187e-06, 2.99133e-06, 3.42515e-06, 3.92114e-06, 4.49253e-06, 5.14099e-06, 5.88197e-06, 6.73388e-06, 7.69827e-06, 8.79826e-06, 1.00505e-05, 1.14867e-05, 1.31084e-05, 1.49676e-05, 1.70609e-05, 1.94389e-05, 2.21526e-05, 2.52108e-05, 2.86887e-05, 3.2585e-05, 3.69848e-05, 4.19856e-05, 4.75668e-05, 5.38457e-05, 6.09384e-05, 6.8832e-05, 6.0933e-05, 5.38293e-05, 4.7549e-05, 4.1964e-05, 3.69624e-05, 3.25575e-05, 2.86601e-05, 2.51835e-05, 2.21335e-05, 1.94169e-05, 1.70425e-05, 1.49505e-05, 1.30926e-05, 1.14729e-05, 1.00378e-05, 8.7856e-06, 7.68648e-06, 6.72357e-06, 5.87283e-06, 5.13321e-06, 4.48541e-06, 3.91479e-06, 3.41982e-06, 2.98613e-06, 2.60712e-06, 2.27402e-06, 1.9852e-06, 1.73291e-06, 1.51243e-06, 1.31878e-06, 1.15105e-06, 1.00473e-06, 8.73592e-07, 7.62236e-07, 6.65138e-07, 5.8028e-07, 5.05874e-07, 4.41403e-07, 3.85205e-07, 3.36194e-07, 2.93149e-07, 2.55868e-07, 2.23409e-07, 1.94879e-07, 1.70201e-07, 1.48666e-07, 1.2986e-07, 1.13347e-07, 9.9043e-08, 8.6567e-08, 7.55938e-08, 6.61033e-08, 5.78057e-08, 5.05225e-08, 4.42007e-08, 3.86861e-08, 3.3832e-08, 2.96229e-08, 2.5945e-08, 2.27092e-08, 1.99003e-08, 1.74304e-08, 1.52806e-08, 1.3401e-08, 1.17444e-08, 1.03069e-08, 9.0485e-09, 7.92018e-09, 6.95589e-09, 6.10949e-09, 5.36312e-09, 4.71469e-09, 4.14605e-09, 3.64381e-09, 3.20526e-09, 2.82135e-09, 2.48098e-09, 2.186e-09, 1.92607e-09, 1.69538e-09, 1.49458e-09, 1.31815e-09, 1.16253e-09, 1.02611e-09, 9.0638e-10, 7.99e-10, 7.0633e-10, 6.25e-10, 5.5101e-10, 4.8828e-10, 4.3127e-10, 3.817e-10, 3.3822e-10, 2.9963e-10, 2.6593e-10, 2.3635e-10, 2.0867e-10, 1.8538e-10, 1.6495e-10, 1.4706e-10, 1.3073e-10, 1.1573e-10, 1.0283e-10, 9.131e-11, 8.23e-11, 7.352e-11, 6.578e-11, 5.766e-11, 5.245e-11, 4.67e-11, 4.123e-11, 3.769e-11, 3.405e-11, 3.024e-11, 2.761e-11, 2.476e-11, 2.251e-11, 2.021e-11, 1.835e-11, 1.6e-11, 1.415e-11, 1.333e-11, 1.195e-11, 1.067e-11, 1.02e-11, 9.57e-12, 7.9e-12, 6.37e-12, 7.99e-12, 8.38e-12, 7.38e-12, 6.33e-12, 4.47e-12, 5.06e-12, 5.48e-12, 4.42e-12, 4.27e-12, 4.14e-12, 4.92e-12, 4.23e-12, 2.87e-12, 2.61e-12, 3.66e-12, 3.21e-12, 2.64e-12, 3.39e-12, 3.2e-12, 3.2e-12, 3.26e-12, 3.26e-12, 2.64e-12, 3.3e-12, 2.16e-12, 1.49e-12, 3.84e-12, 2.79e-12, 2.15e-12, 2.47e-12, 1.46e-12, 2.97e-12, 1.69e-12, 2.26e-12, 2.26e-12, 2.25e-12, 2e-12, 2.54e-12, 1.63e-12, 1.93e-12, 1.97e-12, 1.42e-12, 1.89e-12, 2.56e-12, 2.44e-12, 1.6e-12, 2.77e-12, 2.78e-12, 1.63e-12, 2.64e-12, 2.14e-12, 1.54e-12, 2.24e-12, 2.9e-12, 2.34e-12, 1.15e-12, 1.68e-12, 2.21e-12, 2.34e-12, 1.79e-12, 2.14e-12, 2.33e-12, 1.42e-12, 2.44e-12, 2.04e-12, 1.82e-12, 1.97e-12, 2.05e-12, 1.92e-12, 1.28e-12, 2.53e-12, 2.78e-12]
  out "Mobility Array":dbl[](array[numeric])=[8.42730795294608e-06, 8.320365737465945e-09, 3.3732863829196545e-08, 8.327280629134259e-08, 1.6015210242052114e-08, 2.8540471832412786e-09, 2.8185522052649134e-08, 5.094433604468362e-08, 9.271854477881737e-08, 7.240203740261918e-08, 4.1962881256868745e-08, 5.864065643898759e-10, 2.9479711160547515e-08, 1.7817762067473134e-08, 4.790376520580053e-08, 6.943975022621023e-10, 5.116386456405085e-08, 1.0531392570460425e-08, 8.045820122542513e-08, 2.0869091325435605e-07, 2.5033601292793174e-08, 2.041184408876643e-09, 1.0342851899045321e-10, 2.6257958034195705e-08, 2.198592245133383e-09, 1.7001760594627694e-07, 1.1235248398923812e-09, 1.5785324623372606e-07, 8.687946343243364e-08, 8.687946343243364e-08, 5.251541043512147e-10, 1.4579293092230858e-07, 8.155979047718917e-09, 2.6316889986077026e-08, 2.30443573648374e-08, 8.573134353027616e-08, 1.1951448237617445e-07, 1.5293004946210197e-07, 2.686777445366687e-07, 2.1940239327524883e-07, 5.2270146351242295e-09, 9.99716401547038e-09, 7.666100280908951e-10, 1.0569564855967363e-07, 1.2105999535150441e-07, 1.7110295018527324e-08, 6.274653593628904e-08, 1.515958076686327e-07, 2.3310528858888429e-07, 1.1336254503503093e-08, 3.6204908238680447e-09, 2.089359801682833e-07, 1.3095803447007887e-07, 3.187156460470306e-08, 1.2475329659691555e-07, 2.4346986627610335e-08, 4.77712335287488e-08, 2.547441753530095e-08, 4.122087307592357e-08, 1.1106769509739866e-07, 1.9091904895063394e-08, 7.38526840391342e-08, 4.054399707933924e-08, 3.098282572804771e-08, 1.2725031932750444e-07, 2.3383835267445738e-09, 7.826836058282384e-09, 6.736109371184987e-09, 6.233565281982932e-09, 7.955634798399255e-08, 1.3386697950609897e-10, 1.0903126149142136e-07, 3.139939136102598e-08, 1.9010319869418078e-09, 7.945954792639952e-08, 6.325749286977644e-08, 2.8434497531269273e-08, 5.560139125349351e-09, 1.830838277809465e-07, 1.1570860415085654e-07, 1.2564072124276245e-08, 1.1551170016992992e-07, 7.589137900301959e-08, 1.648159002133359e-07, 1.0751808420261549e-07, 2.4739886893549546e-07, 8.734499903042151e-08, 2.4320440534274585e-07, 3.451994584602821e-07, 1.1561985508860334e-07, 3.224081187134985e-07, 3.4171022044630924e-07, 4.026619716548835e-07, 5.07095361462797e-07, 4.151613489651695e-07, 5.129966341047824e-07, 6.245485740838395e-07, 7.306165276651357e-07, 8.72627889236453e-07, 8.198556420487414e-07, 1.120745850851423e-06, 1.1363745870226574e-06, 1.33324612899069e-06, 1.5518292311848778e-06, 1.782719835754913e-06, 1.9091824584092643e-06, 2.2244580407193426e-06, 2.518835611154334e-06, 3.015938011524284e-06, 3.230770631489752e-06, 3.6351009875254764e-06, 4.352411077990929e-06, 4.799972755411896e-06, 5.618481778716771e-06, 6.157449509666162e-06, 7.175749138465034e-06, 8.245457439551473e-06, 9.193360997204728e-06, 1.0608727521155464e-05, 1.1995008066787043e-05, 1.3868281370371408e-05, 1.586119511866289e-05, 1.802730229238458e-05, 2.033099280125842e-05, 2.368717654391795e-05, 2.669509279203709e-05, 3.0467681907784598e-05, 3.510351826344096e-05, 3.970843029601592e-05, 4.556638611899417e-05, 5.288324128596223e-05, 5.95336736038005e-05, 6.812616883243518e-05, 7.904074446143319e-05, 9.18524967182239e-05, 0.00010174963217932319, 0.00011884670236009769, 0.00013395075201746659, 0.0001536461027060132, 0.00017803016963781505, 0.00020136719848476043, 0.00023472192900570338, 0.00026502582305168817, 0.0003038594271480162, 0.00035360071433007353, 0.00040071901289674103, 0.00045876308529529253, 0.0005331705960261241, 0.0006033729528168363, 0.0006938366951674269, 0.0008066216098344451, 0.0009123335876666689, 0.0010481247397799362, 0.0012220282440107194, 0.0013824189327382433, 0.0015866025286875066, 0.0018148193979770958, 0.002122245869277246, 0.002392508510431417, 0.0027513606691444534, 0.0032094196625004176, 0.0036231889120812506, 0.004169903530580357, 0.004763783517486614, 0.005555417396266736, 0.006289853099142316, 0.00720230557572137, 0.008262981824864813, 0.009984282139798408, 0.010819146551059615, 0.012414900039183477, 0.014425200879304873, 0.016325080172627158, 0.01862025138652243, 0.021363026668915475, 0.02479745632184384, 0.027939705885863097, 0.03188941830681632, 0.036408323603393584, 0.04218990576958308, 0.047457112613011006, 0.05415434807074493, 0.06254520081323862, 0.07006274123717789, 0.07974355017007634, 0.09044811428962575, 0.10412412461757205, 0.11624984531241726, 0.13385081633572296, 0.1487366573565437, 0.16843097089799935, 0.19249044562895987, 0.2146690368042931, 0.2439660236994877, 0.2693379174888114, 0.30248731754837327, 0.3442530679887496, 0.3781180601444472, 0.4225903665387146, 0.4764131529384825, 0.5219200831027319, 0.5226568695385339, 0.4779844020928654, 0.4229219169134312, 0.37880061097716183, 0.3445556936341736, 0.30340774332411147, 0.2697376351777784, 0.24403710705547074, 0.21372800997994965, 0.1930937367755599, 0.16810731413041072, 0.14871696657926328, 0.13382065075893965, 0.11610300783617634, 0.10409287307975537, 0.09056444925745384, 0.07973576084145285, 0.06995498461511336, 0.06246985611407664, 0.05403865128073277, 0.047433980822846604, 0.04214376837014715, 0.03631643206218252, 0.031922795334756365, 0.02792310096692429, 0.02471505933793257, 0.02129372843366805, 0.01861254428204949, 0.01628573377752066, 0.014401207194844907, 0.012384634186724142, 0.010797696886667384, 0.009955072009652826, 0.008241774961594945, 0.007181467960869791, 0.006286407434466546, 0.005541943162782115, 0.004770707164815995, 0.004154052421705281, 0.003620268202148007, 0.003201061177163448, 0.002752440676613388, 0.0023900648031046348, 0.002115734967734768, 0.0018136604057863847, 0.0015812603636286805, 0.0013805434842799286, 0.0012190020186425854, 0.0010473730166916584, 0.0009117334219653627, 0.0008073203015531439, 0.0006910862422827401, 0.0006041113340968446, 0.0005323799621125911, 0.0004587084109102524, 0.00039888821015329274, 0.0003532526639565676, 0.0003035421289911224, 0.00026465457946033385, 0.000233965151027023, 0.00020131023709618604, 0.00017766251806380698, 0.0001536028087818201, 0.00013391267193582748, 0.00011865223352127056, 0.00010187574149860591, 8.89451111543847e-05, 8.156888218640452e-05, 6.795339897222064e-05, 5.9609128981064305e-05, 5.278779449906904e-05, 4.535627329001201e-05, 3.967160857679204e-05, 3.52023871976737e-05, 3.052668164817643e-05, 2.6586071530393583e-05, 2.3752593113789052e-05, 2.0267992981369687e-05, 1.7861335806624855e-05, 1.5975094342277424e-05, 1.3740425258169918e-05, 1.2030170425180587e-05, 1.061243718792287e-05, 9.24339136802347e-06, 8.06367885830808e-06, 7.349941361833767e-06, 6.201343801549878e-06, 5.400683458515212e-06, 5.06049039048221e-06, 4.115636982616189e-06, 3.842127789253647e-06, 3.2854486421136443e-06, 2.854424459210979e-06, 2.5377924152906168e-06, 2.1827011406310393e-06, 1.8934534949351788e-06, 1.8715457266486708e-06, 1.4962169373845941e-06, 1.2949597117073942e-06, 1.114902019331266e-06, 1.0434186439149646e-06, 9.92352460353553e-07, 8.275888146928984e-07, 7.430189278963063e-07, 5.081532592202902e-07, 5.376976103624228e-07, 4.674051967953546e-07, 5.807027265453609e-07, 2.678669357862148e-07, 3.6243967143911393e-07, 3.699009983227492e-07, 1.725302326209487e-07, 2.007004391438298e-07, 2.454231296386084e-07, 1.2991516645477408e-07, 1.6856064993576732e-07, 1.1637314641768617e-07, 1.345756941960057e-07, 9.749197127899203e-08, 1.748015130791986e-07, 1.2339360287735078e-07, 2.6578766861590543e-08, 8.187138714133922e-08, 7.872316812152192e-08, 1.1496231093909046e-08, 2.1807800627779738e-08, 1.7376517179518776e-07, 1.7866503758140373e-07, 1.9910913007479866e-07, 1.0091815816672788e-08, 6.897770215116935e-08, 8.745940699232878e-08, 3.504984034675883e-07, 3.970589667064548e-08, 1.8182668356870404e-08, 1.2361004574739552e-07, 2.812044815950763e-09, 2.182447458913078e-09, 7.306260281334305e-08, 5.658782095495005e-08, 2.8555269110542864e-07, 1.3404107184976785e-08, 1.923160780634276e-07, 3.204512897611636e-08, 6.045823282840954e-08, 1.0170020088139937e-07, 5.950304780871371e-09, 0.0, 6.052105531792235e-10, 0.0, 7.095164406602565e-08, 7.988683819689323e-08, 2.6137054371584065e-07, 1.3470675345725374e-07, 1.1859627893686965e-06, 1.817361675878547e-07, 9.04261549482238e-08, 2.4099439775469745e-08, 2.867033730799208e-07, 5.762087683559222e-07, 3.893093423666347e-07, 8.979631462321217e-08, 0.0, 2.407970349672259e-11, 1.5984328857697692e-08, 7.000080833986825e-08, 2.1829272444116325e-07, 2.750380232637843e-08, 4.455474274416696e-10, 9.755271829837574e-08, 7.284515917566323e-08, 1.1017908646764082e-07, 3.128111196463091e-09, 1.917679725958063e-07, 3.465118820241058e-07, 1.9567462600420016e-11, 3.3140810471412017e-07, 2.631770935766423e-07, 5.6955036926844145e-08, 1.0695405657246102e-07, 1.4200499296700347e-07, 9.241728409654668e-08, 6.518044199453874e-08, 4.5426328934737066e-07, 1.0875558934021854e-07, 7.878779203869647e-08, 4.034512911734045e-09, 7.989892400972736e-08, 3.391832498992551e-08, 8.774514936492631e-09, 2.4345474285231136e-07, 2.980081814717877e-07, 3.886308325878563e-08, 1.3628194464371222e-08, 6.449716440694948e-09, 1.7291157582145603e-09, 4.624234062140053e-09, 1.4042572943461444e-07, 4.5804807617452834e-07, 1.2789498223358228e-08]
  in  "Ids array 2":dbl[](array[numeric])
  out "Vgs index":dbl
  out "Vd array":dbl[](array[numeric])
  in  "Ids Linear":dbl[](array[numeric])=[0.0, 0.000245, 0.0014449999999999999, 0.0036450000000000002, 0.006845, 0.011045000000000001, 0.0, 0.000245, 0.0014449999999999999, 0.0036450000000000002, 0.006845, 0.011045000000000001]
  in  "Vds linear":dbl[](array[numeric])=[0.0, 0.7, 1.7, 2.7, 3.7, 4.7, 0.0, 0.7, 1.7, 2.7, 3.7, 4.7]
  out "Vg array":dbl[](array[numeric])=[1.0, 2.0, 3.0, 4.0, 5.0]
  out "Vds index":dbl=80.0
  in  "Vds array":dbl[](array[numeric])=[0.0, 0.1, 0.2, 0.30000000000000004, 0.4, 0.5, 0.6000000000000001, 0.7000000000000001, 0.8, 0.9, 1.0, 1.1, 1.2000000000000002, 1.3, 1.4000000000000001, 1.5, 1.6, 1.7000000000000002, 1.8, 1.9000000000000001, 2.0, 2.1, 2.2, 2.3000000000000003, 2.4000000000000004, 2.5, 2.6, 2.7, 2.8000000000000003, 2.9000000000000004, 3.0, 3.1, 3.2, 3.3000000000000003, 3.4000000000000004, 3.5, 3.6, 3.7, 3.8000000000000003, 3.9000000000000004, 4.0, 4.1000000000000005, 4.2, 4.3, 4.4, 4.5, 4.6000000000000005, 4.7, 4.800000000000001, 4.9, 5.0, 5.1000000000000005, 5.2, 5.300000000000001, 5.4, 5.5, 5.6000000000000005, 5.7, 5.800000000000001, 5.9, 6.0, 6.1000000000000005, 6.2, 6.300000000000001, 6.4, 6.5, 6.6000000000000005, 6.7, 6.800000000000001, 6.9, 7.0, 7.1000000000000005, 7.2, 7.300000000000001, 7.4, 7.5, 7.6000000000000005, 7.7, 7.800000000000001, 7.9, 0.0, 0.1, 0.2, 0.30000000000000004, 0.4, 0.5, 0.6000000000000001, 0.7000000000000001, 0.8, 0.9, 1.0, 1.1, 1.2000000000000002, 1.3, 1.4000000000000001, 1.5, 1.6, 1.7000000000000002, 1.8, 1.9000000000000001, 2.0, 2.1, 2.2, 2.3000000000000003, 2.4000000000000004, 2.5, 2.6, 2.7, 2.8000000000000003, 2.9000000000000004, 3.0, 3.1, 3.2, 3.3000000000000003, 3.4000000000000004, 3.5, 3.6, 3.7, 3.8000000000000003, 3.9000000000000004, 4.0, 4.1000000000000005, 4.2, 4.3, 4.4, 4.5, 4.6000000000000005, 4.7, 4.800000000000001, 4.9, 5.0, 5.1000000000000005, 5.2, 5.300000000000001, 5.4, 5.5, 5.6000000000000005, 5.7, 5.800000000000001, 5.9, 6.0, 6.1000000000000005, 6.2, 6.300000000000001, 6.4, 6.5, 6.6000000000000005, 6.7, 6.800000000000001, 6.9, 7.0, 7.1000000000000005, 7.2, 7.300000000000001, 7.4, 7.5, 7.6000000000000005, 7.7, 7.800000000000001, 7.9]
  in  "Ids array":dbl[](array[numeric])=[0.0, 6.5e-05, 0.00011999999999999999, 0.000165, 0.00019999999999999996, 0.000225, 0.00024, 0.000245, 0.000245, 0.000245, 0.000245, 0.000245, 0.000245, 0.000245, 0.000245, 0.000245, 0.000245, 0.000245, 0.000245, 0.000245, 0.000245, 0.000245, 0.000245, 0.000245, 0.000245, 0.000245, 0.000245, 0.000245, 0.000245, 0.000245, 0.000245, 0.000245, 0.000245, 0.000245, 0.000245, 0.000245, 0.000245, 0.000245, 0.000245, 0.000245, 0.000245, 0.000245, 0.000245, 0.000245, 0.000245, 0.000245, 0.000245, 0.000245, 0.000245, 0.000245, 0.000245, 0.000245, 0.000245, 0.000245, 0.000245, 0.000245, 0.000245, 0.000245, 0.000245, 0.000245, 0.000245, 0.000245, 0.000245, 0.000245, 0.000245, 0.000245, 0.000245, 0.000245, 0.000245, 0.000245, 0.000245, 0.000245, 0.000245, 0.000245, 0.000245, 0.000245, 0.000245, 0.000245, 0.000245, 0.000245, 0.0, 6.5e-05, 0.00011999999999999999, 0.000165, 0.00019999999999999996, 0.000225, 0.00024, 0.000245, 0.000245, 0.000245, 0.000245, 0.000245, 0.000245, 0.000245, 0.000245, 0.000245, 0.000245, 0.000245, 0.000245, 0.000245, 0.000245, 0.000245, 0.000245, 0.000245, 0.000245, 0.000245, 0.000245, 0.000245, 0.000245, 0.000245, 0.000245, 0.000245, 0.000245, 0.000245, 0.000245, 0.000245, 0.000245, 0.000245, 0.000245, 0.000245, 0.000245, 0.000245, 0.000245, 0.000245, 0.000245, 0.000245, 0.000245, 0.000245, 0.000245, 0.000245, 0.000245, 0.000245, 0.000245, 0.000245, 0.000245, 0.000245, 0.000245, 0.000245, 0.000245, 0.000245, 0.000245, 0.000245, 0.000245, 0.000245, 0.000245, 0.000245, 0.000245, 0.000245, 0.000245, 0.000245, 0.000245, 0.000245, 0.000245, 0.000245, 0.000245, 0.000245, 0.000245, 0.000245, 0.000245, 0.000245]
  out "Index":i32=47
  in  "Tab Control":enum32{"Simulation", "Transfer", "Output"}(tab)=enum."Output"
  in  "Transfer Save Button":bool
  in  "Output Save Button":bool
  out "Output Graph":cluster{"Value":dbl[], "Value":dbl[]}[](graph)
  out "Temp Vg":dbl=5.0
  out "Index 2":i32=4
  out "Ids 2":dbl[](array[numeric])=[0.0, 0.000165, 0.00032, 0.00046499999999999997, 0.0006000000000000001, 0.000725, 0.00084, 0.0009450000000000001, 0.0010400000000000001, 0.0011250000000000001, 0.0012, 0.001265, 0.0013199999999999998, 0.001365, 0.0014000000000000002, 0.0014249999999999998, 0.0014399999999999999, 0.0014449999999999999, 0.0014449999999999999, 0.0014449999999999999, 0.0014449999999999999, 0.0014449999999999999, 0.0014449999999999999, 0.0014449999999999999, 0.0014449999999999999, 0.0014449999999999999, 0.0014449999999999999, 0.0014449999999999999, 0.0014449999999999999, 0.0014449999999999999, 0.0014449999999999999, 0.0014449999999999999, 0.0014449999999999999, 0.0014449999999999999, 0.0014449999999999999, 0.0014449999999999999, 0.0014449999999999999, 0.0014449999999999999, 0.0014449999999999999, 0.0014449999999999999, 0.0014449999999999999, 0.0014449999999999999, 0.0014449999999999999, 0.0014449999999999999, 0.0014449999999999999, 0.0014449999999999999, 0.0014449999999999999, 0.0014449999999999999, 0.0014449999999999999, 0.0014449999999999999, 0.0014449999999999999, 0.0014449999999999999, 0.0014449999999999999, 0.0014449999999999999, 0.0014449999999999999, 0.0014449999999999999, 0.0014449999999999999, 0.0014449999999999999, 0.0014449999999999999, 0.0014449999999999999, 0.0014449999999999999, 0.0014449999999999999, 0.0014449999999999999, 0.0014449999999999999, 0.0014449999999999999, 0.0014449999999999999, 0.0014449999999999999, 0.0014449999999999999, 0.0014449999999999999, 0.0014449999999999999, 0.0014449999999999999, 0.0014449999999999999, 0.0014449999999999999, 0.0014449999999999999, 0.0014449999999999999, 0.0014449999999999999, 0.0014449999999999999, 0.0014449999999999999, 0.0014449999999999999, 0.0014449999999999999, 0.0, 0.000165, 0.00032, 0.00046499999999999997, 0.0006000000000000001, 0.000725, 0.00084, 0.0009450000000000001, 0.0010400000000000001, 0.0011250000000000001, 0.0012, 0.001265, 0.0013199999999999998, 0.001365, 0.0014000000000000002, 0.0014249999999999998, 0.0014399999999999999, 0.0014449999999999999, 0.0014449999999999999, 0.0014449999999999999, 0.0014449999999999999, 0.0014449999999999999, 0.0014449999999999999, 0.0014449999999999999, 0.0014449999999999999, 0.0014449999999999999, 0.0014449999999999999, 0.0014449999999999999, 0.0014449999999999999, 0.0014449999999999999, 0.0014449999999999999, 0.0014449999999999999, 0.0014449999999999999, 0.0014449999999999999, 0.0014449999999999999, 0.0014449999999999999, 0.0014449999999999999, 0.0014449999999999999, 0.0014449999999999999, 0.0014449999999999999, 0.0014449999999999999, 0.0014449999999999999, 0.0014449999999999999, 0.0014449999999999999, 0.0014449999999999999, 0.0014449999999999999, 0.0014449999999999999, 0.0014449999999999999, 0.0014449999999999999, 0.0014449999999999999, 0.0014449999999999999, 0.0014449999999999999, 0.0014449999999999999, 0.0014449999999999999, 0.0014449999999999999, 0.0014449999999999999, 0.0014449999999999999, 0.0014449999999999999, 0.0014449999999999999, 0.0014449999999999999, 0.0014449999999999999, 0.0014449999999999999, 0.0014449999999999999, 0.0014449999999999999, 0.0014449999999999999, 0.0014449999999999999, 0.0014449999999999999, 0.0014449999999999999, 0.0014449999999999999, 0.0014449999999999999, 0.0014449999999999999, 0.0014449999999999999, 0.0014449999999999999, 0.0014449999999999999, 0.0014449999999999999, 0.0014449999999999999, 0.0014449999999999999, 0.0014449999999999999, 0.0014449999999999999, 0.0014449999999999999]
  out "Ids 3":dbl[](array[numeric])=[0.0, 0.00026500000000000004, 0.0005200000000000001, 0.0007650000000000002, 0.001, 0.0012250000000000002, 0.0014400000000000005, 0.0016450000000000002, 0.00184, 0.0020250000000000003, 0.0022, 0.0023650000000000008, 0.0025200000000000005, 0.0026650000000000003, 0.002800000000000001, 0.002925000000000001, 0.00304, 0.0031450000000000007, 0.0032400000000000003, 0.0033250000000000007, 0.0034000000000000002, 0.0034650000000000006, 0.003520000000000001, 0.0035650000000000005, 0.0036000000000000008, 0.003625, 0.00364, 0.0036450000000000007, 0.0036450000000000002, 0.0036450000000000002, 0.0036450000000000002, 0.0036450000000000002, 0.0036450000000000002, 0.0036450000000000002, 0.0036450000000000002, 0.0036450000000000002, 0.0036450000000000002, 0.0036450000000000002, 0.0036450000000000002, 0.0036450000000000002, 0.0036450000000000002, 0.0036450000000000002, 0.0036450000000000002, 0.0036450000000000002, 0.0036450000000000002, 0.0036450000000000002, 0.0036450000000000002, 0.0036450000000000002, 0.0036450000000000002, 0.0036450000000000002, 0.0036450000000000002, 0.0036450000000000002, 0.0036450000000000002, 0.0036450000000000002, 0.0036450000000000002, 0.0036450000000000002, 0.0036450000000000002, 0.0036450000000000002, 0.0036450000000000002, 0.0036450000000000002, 0.0036450000000000002, 0.0036450000000000002, 0.0036450000000000002, 0.0036450000000000002, 0.0036450000000000002, 0.0036450000000000002, 0.0036450000000000002, 0.0036450000000000002, 0.0036450000000000002, 0.0036450000000000002, 0.0036450000000000002, 0.0036450000000000002, 0.0036450000000000002, 0.0036450000000000002, 0.0036450000000000002, 0.0036450000000000002, 0.0036450000000000002, 0.0036450000000000002, 0.0036450000000000002, 0.0036450000000000002, 0.0, 0.00026500000000000004, 0.0005200000000000001, 0.0007650000000000002, 0.001, 0.0012250000000000002, 0.0014400000000000005, 0.0016450000000000002, 0.00184, 0.0020250000000000003, 0.0022, 0.0023650000000000008, 0.0025200000000000005, 0.0026650000000000003, 0.002800000000000001, 0.002925000000000001, 0.00304, 0.0031450000000000007, 0.0032400000000000003, 0.0033250000000000007, 0.0034000000000000002, 0.0034650000000000006, 0.003520000000000001, 0.0035650000000000005, 0.0036000000000000008, 0.003625, 0.00364, 0.0036450000000000007, 0.0036450000000000002, 0.0036450000000000002, 0.0036450000000000002, 0.0036450000000000002, 0.0036450000000000002, 0.0036450000000000002, 0.0036450000000000002, 0.0036450000000000002, 0.0036450000000000002, 0.0036450000000000002, 0.0036450000000000002, 0.0036450000000000002, 0.0036450000000000002, 0.0036450000000000002, 0.0036450000000000002, 0.0036450000000000002, 0.0036450000000000002, 0.0036450000000000002, 0.0036450000000000002, 0.0036450000000000002, 0.0036450000000000002, 0.0036450000000000002, 0.0036450000000000002, 0.0036450000000000002, 0.0036450000000000002, 0.0036450000000000002, 0.0036450000000000002, 0.0036450000000000002, 0.0036450000000000002, 0.0036450000000000002, 0.0036450000000000002, 0.0036450000000000002, 0.0036450000000000002, 0.0036450000000000002, 0.0036450000000000002, 0.0036450000000000002, 0.0036450000000000002, 0.0036450000000000002, 0.0036450000000000002, 0.0036450000000000002, 0.0036450000000000002, 0.0036450000000000002, 0.0036450000000000002, 0.0036450000000000002, 0.0036450000000000002, 0.0036450000000000002, 0.0036450000000000002, 0.0036450000000000002, 0.0036450000000000002, 0.0036450000000000002, 0.0036450000000000002, 0.0036450000000000002]
  out "Ids 4":dbl[](array[numeric])=[0.0, 0.00036500000000000004, 0.00072, 0.0010650000000000004, 0.0014000000000000002, 0.0017250000000000002, 0.0020400000000000006, 0.0023450000000000003, 0.0026400000000000004, 0.002925, 0.0032, 0.003465, 0.003720000000000001, 0.003965000000000001, 0.004200000000000001, 0.004425000000000001, 0.004640000000000001, 0.004845, 0.00504, 0.005225000000000001, 0.0054, 0.0055650000000000005, 0.005720000000000001, 0.005865000000000001, 0.006000000000000002, 0.006125, 0.006240000000000001, 0.006345000000000002, 0.00644, 0.006525000000000001, 0.006600000000000002, 0.006665, 0.006720000000000001, 0.006765, 0.0068000000000000005, 0.006825000000000001, 0.00684, 0.006845, 0.006845, 0.006845, 0.006845, 0.006845, 0.006845, 0.006845, 0.006845, 0.006845, 0.006845, 0.006845, 0.006845, 0.006845, 0.006845, 0.006845, 0.006845, 0.006845, 0.006845, 0.006845, 0.006845, 0.006845, 0.006845, 0.006845, 0.006845, 0.006845, 0.006845, 0.006845, 0.006845, 0.006845, 0.006845, 0.006845, 0.006845, 0.006845, 0.006845, 0.006845, 0.006845, 0.006845, 0.006845, 0.006845, 0.006845, 0.006845, 0.006845, 0.006845, 0.0, 0.00036500000000000004, 0.00072, 0.0010650000000000004, 0.0014000000000000002, 0.0017250000000000002, 0.0020400000000000006, 0.0023450000000000003, 0.0026400000000000004, 0.002925, 0.0032, 0.003465, 0.003720000000000001, 0.003965000000000001, 0.004200000000000001, 0.004425000000000001, 0.004640000000000001, 0.004845, 0.00504, 0.005225000000000001, 0.0054, 0.0055650000000000005, 0.005720000000000001, 0.005865000000000001, 0.006000000000000002, 0.006125, 0.006240000000000001, 0.006345000000000002, 0.00644, 0.006525000000000001, 0.006600000000000002, 0.006665, 0.006720000000000001, 0.006765, 0.0068000000000000005, 0.006825000000000001, 0.00684, 0.006845, 0.006845, 0.006845, 0.006845, 0.006845, 0.006845, 0.006845, 0.006845, 0.006845, 0.006845, 0.006845, 0.006845, 0.006845, 0.006845, 0.006845, 0.006845, 0.006845, 0.006845, 0.006845, 0.006845, 0.006845, 0.006845, 0.006845, 0.006845, 0.006845, 0.006845, 0.006845, 0.006845, 0.006845, 0.006845, 0.006845, 0.006845, 0.006845, 0.006845, 0.006845, 0.006845, 0.006845, 0.006845, 0.006845, 0.006845, 0.006845, 0.006845, 0.006845]
  out "Ids 5":dbl[](array[numeric])=[0.0, 0.000465, 0.00092, 0.0013650000000000005, 0.0018000000000000002, 0.002225, 0.0026400000000000004, 0.0030450000000000004, 0.0034400000000000003, 0.0038250000000000003, 0.004200000000000001, 0.0045650000000000005, 0.004920000000000002, 0.005265000000000001, 0.005600000000000001, 0.005925000000000001, 0.006240000000000001, 0.006545000000000001, 0.006840000000000001, 0.007125000000000002, 0.0074, 0.007665000000000001, 0.007920000000000002, 0.008165000000000002, 0.008400000000000003, 0.008625, 0.00884, 0.009045000000000003, 0.009240000000000002, 0.009425000000000001, 0.009600000000000001, 0.009765000000000001, 0.00992, 0.010065000000000001, 0.0102, 0.010324999999999999, 0.010440000000000001, 0.010545, 0.010640000000000002, 0.010725000000000002, 0.0108, 0.010865, 0.010920000000000003, 0.010965000000000003, 0.011000000000000003, 0.011025000000000002, 0.011040000000000003, 0.011045000000000003, 0.011045000000000001, 0.011045000000000001, 0.011045000000000001, 0.011045000000000001, 0.011045000000000001, 0.011045000000000001, 0.011045000000000001, 0.011045000000000001, 0.011045000000000001, 0.011045000000000001, 0.011045000000000001, 0.011045000000000001, 0.011045000000000001, 0.011045000000000001, 0.011045000000000001, 0.011045000000000001, 0.011045000000000001, 0.011045000000000001, 0.011045000000000001, 0.011045000000000001, 0.011045000000000001, 0.011045000000000001, 0.011045000000000001, 0.011045000000000001, 0.011045000000000001, 0.011045000000000001, 0.011045000000000001, 0.011045000000000001, 0.011045000000000001, 0.011045000000000001, 0.011045000000000001, 0.011045000000000001, 0.0, 0.000465, 0.00092, 0.0013650000000000005, 0.0018000000000000002, 0.002225, 0.0026400000000000004, 0.0030450000000000004, 0.0034400000000000003, 0.0038250000000000003, 0.004200000000000001, 0.0045650000000000005, 0.004920000000000002, 0.005265000000000001, 0.005600000000000001, 0.005925000000000001, 0.006240000000000001, 0.006545000000000001, 0.006840000000000001, 0.007125000000000002, 0.0074, 0.007665000000000001, 0.007920000000000002, 0.008165000000000002, 0.008400000000000003, 0.008625, 0.00884, 0.009045000000000003, 0.009240000000000002, 0.009425000000000001, 0.009600000000000001, 0.009765000000000001, 0.00992, 0.010065000000000001, 0.0102, 0.010324999999999999, 0.010440000000000001, 0.010545, 0.010640000000000002, 0.010725000000000002, 0.0108, 0.010865, 0.010920000000000003, 0.010965000000000003, 0.011000000000000003, 0.011025000000000002, 0.011040000000000003, 0.011045000000000003, 0.011045000000000001, 0.011045000000000001, 0.011045000000000001, 0.011045000000000001, 0.011045000000000001, 0.011045000000000001, 0.011045000000000001, 0.011045000000000001, 0.011045000000000001, 0.011045000000000001, 0.011045000000000001, 0.011045000000000001, 0.011045000000000001, 0.011045000000000001, 0.011045000000000001, 0.011045000000000001, 0.011045000000000001, 0.011045000000000001, 0.011045000000000001, 0.011045000000000001, 0.011045000000000001, 0.011045000000000001, 0.011045000000000001, 0.011045000000000001, 0.011045000000000001, 0.011045000000000001, 0.011045000000000001, 0.011045000000000001, 0.011045000000000001, 0.011045000000000001, 0.011045000000000001, 0.011045000000000001]
  out "Temp Vd":dbl
  out "Index 3":i32
  out "Ids 6":dbl[](array[numeric])
  out "Ids 7":dbl[](array[numeric])
  out "Ids 8":dbl[](array[numeric])
  out "Ids 9":dbl[](array[numeric])
  out "Transfer Graph":cluster{"Y":dbl[], "Y":dbl[]}[](graph)
  in  "Width [um]":dbl=0.001
  in  "Length [um]":dbl=0.001
  in  "Capactiance [nf]":dbl=0.001
  in  "Vt [V]":dbl=0.3
  in  "STEP":dbl=0.1
  in  "u [cm^2/Vs]":dbl=1.0
  in  "Transfer Start":bool
  in  "Vgs [V]":dbl=6.0
  in  "Vd 1 [V]":dbl=1.0
  in  "Vd 2 [V]":dbl=2.0
  in  "Vd 3 [V]":dbl=3.0
  in  "Vd 4 [V]":dbl=4.0
  in  "Vd 5 [V]":dbl=5.0
  in  "Stop Program":bool
  in  "Graph Clear.":bool
  in  "Vg 5 [A]":dbl=5.0
  in  "Vg 4 [A]":dbl=4.0
  in  "Vg 3 [A]":dbl=3.0
  in  "Vg 2 [A]":dbl=2.0
  in  "Vds [A]":dbl=8.0
  in  "Simulation Start":bool
  in  "Vg 1 [V]":dbl=1.0
  in  "Clear Graph":bool
  in  "Vgs array":dbl[](array[numeric])
  out "ID-VG 2":cluster{"Y":dbl[], "Y":dbl[]}[](graph)
  in  "Hysteresis":bool
  in  "Transfer Save":bool
  in  "Cancel Button":bool
  in  "Stop Button":bool
  in  "Run Button":bool
  out "Hysteresis LED":bool=TRUE
  in  "Length [um]":dbl=25.0 min=0.0
  in  "Thickness [nm]":dbl=3e-07 min=0.0 format="%#_6e"
  in  "Width [um]":dbl=2000.0 min=0.0
  in  "Int time":dbl=5.0 min=1.0 max=100.0
  in  "VISA resource name":refnum<visa-resource-name>="GPIB0::16::INSTR"
  in  "VD Comp [V].":dbl=0.001 format="%#_6e"
  in  "VS Comp [V].":dbl=0.001 format="%#_6e"
  in  "VD [V]":dbl=2.0
  in  "VS [V]":dbl
  in  "VD SMU No":dbl=2.0 min=1.0 max=4.0
  in  "VS SMU No":dbl=3.0 min=1.0 max=4.0
  in  "VG Comp [V].":dbl=0.001 format="%#_6e"
  in  "VG SMU No":dbl=1.0 min=1.0 max=4.0
  out "IG [V]":dbl=6.9e-14 format="%#_3e"
  out "IS [V]":dbl=-1.4e-12 format="%#_3e"
  out "ID [V]":dbl=2.78e-12 format="%#_3e"
  in  "Regime":bool=TRUE
  out "Mobility-VG":cluster{"Y":dbl[], "Y":dbl[]}[](graph)
  out "ID-VG":cluster{"Y":dbl[], "Y":dbl[]}[](graph)
  out "IS-VG":cluster{"Y":dbl[], "Y":dbl[]}[](graph)
  out "VG [V]":dbl=-3.0878077872387166e-16
  in  "VG stop [V]":dbl=2.0
  in  "VG start [V]":dbl
  out "Mobility [cm^2/Vs]":dbl=1.2789498223358228e-08 format="%#_2e"
  in  "VG step [V]":dbl=0.01
  in  "Repeat Times":i32
  in  "Repeat Times.":i32
  out "Processing Detector":bool
  out "Hysteresis LED.":bool=TRUE
  out "VD vs. IG":cluster{"Y":dbl[], "Y":dbl[]}[](graph)
  out "VD vs. IS":cluster{"Y":dbl[], "Y":dbl[]}[](graph)
  in  "Output Save":bool
  in  "Cancel Running":bool
  in  "Output Stop":bool
  in  "Start Button":bool
  in  "Int Time [Second]":dbl=2.0
  in  "Source comp [V].":dbl=0.001 format="%#_6e"
  in  "VS [V].":dbl
  in  "Source SMU no.":dbl=3.0
  in  "VISA resource name.":refnum<visa-resource-name>="GPIB0::16::INSTR"
  in  "VG Step. [V]":dbl=0.5
  in  "VG Stop. [V]":dbl=2.0
  in  "VG Start. [V]":dbl
  out "ID Array.":dbl[](array[numeric])=[-5.26e-12, -1.35e-12, -1.36e-12, -1.37e-12, -5.2e-13, -1.19e-12, -2.1e-13, -1e-13, -9.3e-13, -1.48e-12, -1.7e-13, -3.3e-13, 3.2e-13, -4.5e-13, -1.17e-12, -4.4e-13, 2e-14, -7.6e-13, -1.1e-12, 4.7e-13, 2e-14, 8.2e-13, 1e-12, 6.3e-13, 1e-13, 5.7e-13, 8.6e-13, 6.7e-13, 9.2e-13, 1.06e-12, -7.8e-13, 3.2e-13, 8.4e-13, 8.6e-13, -3.6e-13, -1.2e-13, 7.3e-13, 1.7e-12, -5.4e-13, -4e-14, -3.2e-13, 4.5e-13, 9.6e-13, 7.3e-13, 1.12e-12, 9.9e-13, 3.06e-12, -4e-13, 5.9e-13, -1.3e-13, 1.07e-12, 1.3e-12, 8.2e-13, 1.34e-12, 1.16e-12, 1.43e-12, 5e-13, 3.1e-13, 1.57e-12, 1.36e-12, 8.4e-13, 1.07e-12, 1.17e-12, 1.41e-12, 1.8e-13, 1.68e-12, 6.3e-13, 2e-13, -5e-14, 9.3e-13, -5.6e-13, 9e-13, 6e-13, 2.03e-12, 2.1e-12, 1.86e-12, 1.16e-12, 2.3e-13, -8e-14, 4e-13, 5.2e-13, 8.9e-13, 5.6e-13, 2.1e-13, 1.67e-12, 1.01e-12, 6.8e-13, 2.6e-13, 1.92e-12, 1.4e-13, 6.9e-13, 1.4e-12, 1.13e-12, 3.2e-13, 1.74e-12, 1.43e-12, 1.2e-12, 2e-14, 2.08e-12, 1.2e-13, -3e-13, 1.77e-12, 1.49e-12, 2.8e-13, 8.5e-13, 0.0, 1.97e-12, 2.11e-12, 1.08e-12, 1.09e-12, 1.11e-12, 6.9e-13, 1.35e-12, 1.91e-12, 1.96e-12, 2.18e-12, 2.34e-12, 1.66e-12, 1.77e-12, 2.04e-12, 2.65e-12, 6.3e-13, 1.1e-12, 1.28e-12, 7.7e-13, 1.91e-12, 1.92e-12, 2.07e-12, 1.49e-12, 8.2e-13, 2.16e-12, 2.29e-12, 1.84e-12, 1.48e-12, 1.77e-12, 1.94e-12, 4e-14, 2.59e-12, 2.96e-12, 1.06e-12, 2.03e-12, 2.5e-12, 3.48e-12, 3.09e-12, 2.78e-12, 1.25e-12, 1.5e-12, 2.92e-12, 1.51e-12, 3.15e-12, 2.4e-12, 2.28e-12, 1.92e-12, 8e-13, 1.26e-12, 2.97e-12, 1.85e-12, 3.32e-12, 3.14e-12, 2.26e-12, 1.93e-12, 1.73e-12, 1.54e-12, 1.19e-12, 2.08e-12, 1.31e-12, 1.94e-12, 2.44e-12, 2.39e-12, 2.22e-12, 2.65e-12, 2.29e-12, 2.22e-12, 3.13e-12, 2.82e-12, 1.55e-12, 9.5e-13, 1.68e-12, 1.15e-12, 2.92e-12, 2.58e-12, 2.15e-12, 1.42e-12, 1.86e-12, 6.3e-13, 2.32e-12, 2.67e-12, 3.14e-12, 3.59e-12, 2.48e-12, 2.95e-12, 2.79e-12, 1.87e-12, 3.49e-12, 1.7e-12, 2.25e-12, 1.68e-12, 2.62e-12, 1.74e-12, 2.09e-12, 3.02e-12, -8.63e-12, -1.13e-12, -1.3e-12, 6e-14, 7.1e-13, 1.16e-12, 1.26e-12, 1.68e-12, -3.7e-13, 1.87e-12, -6e-13, 7.2e-13, 1.41e-12, 1.63e-12, 1.26e-12, -7.9e-13, 8.6e-13, 1.41e-12, 7.9e-13, 3.8e-13, -1.5e-13, 8e-13, 2.5e-13, 4.2e-13, 7e-14, 9.7e-13, 8.7e-13, 1.77e-12, 2.53e-12, 3.4e-13, 7.1e-13, 2.18e-12, 1.3e-12, 1.6e-13, 1.98e-12, 3.9e-13, 8.9e-13, 9.9e-13, 6.4e-13, 1.08e-12, 2.4e-12, 2.5e-13, 1.3e-12, 1.52e-12, 1.17e-12, 4.9e-13, 2.68e-12, 1.07e-12, 8.8e-13, 1.21e-12, 7e-13, 1.1e-12, 1.05e-12, 1.09e-12, 1.5e-13, 1e-13, 2.37e-12, 1.42e-12, 6.5e-13, 1.92e-12, 1.05e-12, 1.57e-12, 5.3e-13, 2.37e-12, 1.65e-12, 1.49e-12, 2.15e-12, 1.2e-13, 3.49e-12, 4.1e-13, 3.8e-13, -2.7e-13, 6.6e-13, 9.4e-13, 2.4e-12, 1.21e-12, 8.6e-13, 1.76e-12, 1.97e-12, 8.9e-13, 1.32e-12, 1.82e-12, 8e-14, 4.9e-13, 1.99e-12, 8.9e-13, 2.31e-12, 1.36e-12, 1.71e-12, 1.69e-12, 2.57e-12, 1.78e-12, 1.43e-12, 2.28e-12, 1.69e-12, 2.05e-12, 5e-13, 2.13e-12, 2.03e-12, 2.23e-12, 2.2e-13, 1.7e-12, 2.14e-12, 2e-12, 2.17e-12, 8.2e-13, 7.9e-13, 1.76e-12, 1.35e-12, 2.39e-12, 5.6e-13, 8e-13, 5.9e-13, 2.06e-12, 9.8e-13, 2.54e-12, 1.05e-12, 1.18e-12, 2.08e-12, 2.07e-12, 1.49e-12, 8.1e-13, 4.6e-13, 1.47e-12, 2.83e-12, 1.04e-12, 1.59e-12, 1e-12, 1.4e-13, 2.24e-12, 7.7e-13, 1.24e-12, 2.04e-12, 1.56e-12, 1.41e-12, 1.64e-12, 1.79e-12, 3.6e-13, 1.09e-12, 2.12e-12, 2.54e-12, 1.95e-12, 2.57e-12, 7.4e-13, 1.64e-12, 5e-13, 1.42e-12, 2.61e-12, 1.17e-12, 1.32e-12, 1.24e-12, 1.31e-12, 2.84e-12, 3.15e-12, 2.04e-12, 2.47e-12, 9.6e-13, 2.44e-12, 1.37e-12, 2.45e-12, 2.1e-12, 2.64e-12, 2.42e-12, 2.94e-12, 2.68e-12, 2.81e-12, 2.48e-12, 3e-12, 3.33e-12, 2.7e-12, 5.08e-12, 3.06e-12, 3.18e-12, 3.2e-12, 1.3e-12, 1.23e-12, 1.32e-12, 1.94e-12, 2.06e-12, 3.5e-12, 1.53e-12, 1.33e-12, 3.29e-12, 3.38e-12, 2.47e-12, 2.22e-12, 1.74e-12, 3.06e-12, 3.56e-12, 1.83e-12, 2.21e-12, 1.66e-12, 3.21e-12, 3.45e-12, 3.73e-12, 3.59e-12, 3.25e-12, 3.23e-12, 2.52e-12, 2.13e-12, 2.49e-12, -1.051e-11, 4.385e-11, 7.625e-11, 9.738e-11, 1.1111e-10, 1.2094e-10, 1.2752e-10, 1.3105e-10, 1.3353e-10, 1.36e-10, 1.4058e-10, 1.384e-10, 1.3919e-10, 1.4028e-10, 1.3997e-10, 1.3994e-10, 1.4036e-10, 1.413e-10, 1.4188e-10, 1.406e-10, 1.4104e-10, 1.4043e-10, 1.4077e-10, 1.4167e-10, 1.4168e-10, 1.406e-10, 1.4193e-10, 1.4216e-10, 1.4045e-10, 1.4047e-10, 1.4096e-10, 1.4047e-10, 1.4157e-10, 1.4159e-10, 1.4066e-10, 1.4145e-10, 1.422e-10, 1.4054e-10, 1.4157e-10, 1.4254e-10, 1.4277e-10, 1.4145e-10, 1.4077e-10, 1.4266e-10, 1.4081e-10, 1.4165e-10, 1.4159e-10, 1.418e-10, 1.4236e-10, 1.4364e-10, 1.4258e-10, 1.419e-10, 1.4172e-10, 1.4213e-10, 1.4249e-10, 1.4202e-10, 1.4202e-10, 1.4096e-10, 1.4139e-10, 1.4206e-10, 1.416e-10, 1.4302e-10, 1.4327e-10, 1.4223e-10, 1.4126e-10, 1.4143e-10, 1.4233e-10, 1.4144e-10, 1.414e-10, 1.4352e-10, 1.4225e-10, 1.425e-10, 1.4213e-10, 1.4329e-10, 1.421e-10, 1.4243e-10, 1.4295e-10, 1.4365e-10, 1.4222e-10, 1.4148e-10, 1.418e-10, 1.4316e-10, 1.4267e-10, 1.4276e-10, 1.4303e-10, 1.4188e-10, 1.4223e-10, 1.4403e-10, 1.4365e-10, 1.4215e-10, 1.4319e-10, 1.4306e-10, 1.4285e-10, 1.4321e-10, 1.4322e-10, 1.4208e-10, 1.4482e-10, 1.4309e-10, 1.4256e-10, 1.4364e-10, 1.43e-10, 1.432e-10, 1.417e-10, 1.4258e-10, 1.4256e-10, 1.4313e-10, 1.4312e-10, 1.4348e-10, 1.4375e-10, 1.4335e-10, 1.4437e-10, 1.4393e-10, 1.4505e-10, 1.4268e-10, 1.4357e-10, 1.4257e-10, 1.4435e-10, 1.4372e-10, 1.4327e-10, 1.4441e-10, 1.4424e-10, 1.4407e-10, 1.45e-10, 1.4288e-10, 1.4285e-10, 1.4324e-10, 1.4264e-10, 1.4393e-10, 1.435e-10, 1.4383e-10, 1.4257e-10, 1.4367e-10, 1.4422e-10, 1.439e-10, 1.4459e-10, 1.4362e-10, 1.4309e-10, 1.4325e-10, 1.4331e-10, 1.445e-10, 1.4378e-10, 1.4379e-10, 1.4485e-10, 1.444e-10, 1.4337e-10, 1.435e-10, 1.4473e-10, 1.4349e-10, 1.4378e-10, 1.448e-10, 1.4522e-10, 1.4503e-10, 1.4488e-10, 1.4342e-10, 1.432e-10, 1.439e-10, 1.4511e-10, 1.4482e-10, 1.4401e-10, 1.4359e-10, 1.4487e-10, 1.4518e-10, 1.4383e-10, 1.4408e-10, 1.4377e-10, 1.4508e-10, 1.4503e-10, 1.4487e-10, 1.4561e-10, 1.4396e-10, 1.4533e-10, 1.4368e-10, 1.4335e-10, 1.4524e-10, 1.4523e-10, 1.4424e-10, 1.4411e-10, 1.4382e-10, 1.4586e-10, 1.4481e-10, 1.441e-10, 1.4415e-10, 1.451e-10, 1.4449e-10, 1.4513e-10, 1.4524e-10, 1.4532e-10, 1.4532e-10, 1.4558e-10, 1.4328e-10, 1.4517e-10, 1.4549e-10, 1.4407e-10, 1.441e-10, 1.4499e-10, 1.4506e-10, 1.4476e-10, 1.4469e-10, 1.4516e-10, 1.4512e-10, 1.4493e-10, 2.4224e-10, 2.54604e-08, 4.26347e-08, 5.43301e-08, 6.23163e-08, 6.77817e-08, 7.15229e-08, 7.41156e-08, 7.58981e-08, 7.71542e-08, 7.80353e-08, 7.86733e-08, 7.91409e-08, 7.94757e-08, 7.9749e-08, 7.99542e-08, 8.01258e-08, 8.02581e-08, 8.03812e-08, 8.04917e-08, 8.0582e-08, 8.06637e-08, 8.07449e-08, 8.08173e-08, 8.08874e-08, 8.09494e-08, 8.10232e-08, 8.10875e-08, 8.11356e-08, 8.11943e-08, 8.12416e-08, 8.13071e-08, 8.13576e-08, 8.14105e-08, 8.14626e-08, 8.15109e-08, 8.15714e-08, 8.16114e-08, 8.16568e-08, 8.17141e-08, 8.17592e-08, 8.17998e-08, 8.18503e-08, 8.18994e-08, 8.1941e-08, 8.19852e-08, 8.20254e-08, 8.20727e-08, 8.21096e-08, 8.21496e-08, 8.21838e-08, 8.22264e-08, 8.22557e-08, 8.23025e-08, 8.23403e-08, 8.23739e-08, 8.24128e-08, 8.24505e-08, 8.24906e-08, 8.25302e-08, 8.25597e-08, 8.2591e-08, 8.26305e-08, 8.26559e-08, 8.26908e-08, 8.27231e-08, 8.27592e-08, 8.27943e-08, 8.28233e-08, 8.28544e-08, 8.28913e-08, 8.29163e-08, 8.29522e-08, 8.29802e-08, 8.30151e-08, 8.30373e-08, 8.30702e-08, 8.31083e-08, 8.31362e-08, 8.31583e-08, 8.31884e-08, 8.32176e-08, 8.32521e-08, 8.32861e-08, 8.33174e-08, 8.33403e-08, 8.33762e-08, 8.3411e-08, 8.34217e-08, 8.34587e-08, 8.34883e-08, 8.35099e-08, 8.35395e-08, 8.35608e-08, 8.3592e-08, 8.36161e-08, 8.36507e-08, 8.36694e-08, 8.37031e-08, 8.37153e-08, 8.37406e-08, 8.37612e-08, 8.37783e-08, 8.38078e-08, 8.38345e-08, 8.38616e-08, 8.38829e-08, 8.39066e-08, 8.3925e-08, 8.39486e-08, 8.3971e-08, 8.39908e-08, 8.40109e-08, 8.40374e-08, 8.40549e-08, 8.40755e-08, 8.41007e-08, 8.41194e-08, 8.41478e-08, 8.4171e-08, 8.41943e-08, 8.42202e-08, 8.42427e-08, 8.42701e-08, 8.42881e-08, 8.43135e-08, 8.4333e-08, 8.43505e-08, 8.43643e-08, 8.43932e-08, 8.44129e-08, 8.44429e-08, 8.44608e-08, 8.44777e-08, 8.45063e-08, 8.45201e-08, 8.4543e-08, 8.45655e-08, 8.45988e-08, 8.46187e-08, 8.46399e-08, 8.46644e-08, 8.46814e-08, 8.47018e-08, 8.47215e-08, 8.47495e-08, 8.47801e-08, 8.47971e-08, 8.48271e-08, 8.4849e-08, 8.48625e-08, 8.48826e-08, 8.49056e-08, 8.49235e-08, 8.49486e-08, 8.49624e-08, 8.49781e-08, 8.50073e-08, 8.50249e-08, 8.50392e-08, 8.50597e-08, 8.50849e-08, 8.51037e-08, 8.51241e-08, 8.51435e-08, 8.51639e-08, 8.51765e-08, 8.52071e-08, 8.52136e-08, 8.52272e-08, 8.52481e-08, 8.52675e-08, 8.5292e-08, 8.53082e-08, 8.53282e-08, 8.53392e-08, 8.53576e-08, 8.53773e-08, 8.53892e-08, 8.53981e-08, 8.54214e-08, 8.54364e-08, 8.54529e-08, 8.54705e-08, 8.549e-08, 8.55064e-08, 8.55203e-08, 8.55449e-08, 8.556e-08, 8.55768e-08, 8.56038e-08, 8.56116e-08, 8.56375e-08, 8.56543e-08, 8.56655e-08, 8.56864e-08, 8.56996e-08, 8.5724e-08, 8.57489e-08, 8.57642e-08, 8.57805e-08, 5.80611e-08, 5.88439e-06, 1.14739e-05, 1.68037e-05, 2.18373e-05, 2.65517e-05, 3.09319e-05, 3.49405e-05, 3.8569e-05, 4.1797e-05, 4.46411e-05, 4.71025e-05, 4.92052e-05, 5.09863e-05, 5.24794e-05, 5.3732e-05, 5.47774e-05, 5.56582e-05, 5.64019e-05, 5.70377e-05, 5.75874e-05, 5.80618e-05, 5.84806e-05, 5.88594e-05, 5.91947e-05, 5.94959e-05, 5.97847e-05, 6.00376e-05, 6.02726e-05, 6.04963e-05, 6.07013e-05, 6.08858e-05, 6.10685e-05, 6.12398e-05, 6.14064e-05, 6.15521e-05, 6.1699e-05, 6.18313e-05, 6.19681e-05, 6.20864e-05, 6.22007e-05, 6.23234e-05, 6.24371e-05, 6.25348e-05, 6.26348e-05, 6.27363e-05, 6.28273e-05, 6.29151e-05, 6.30097e-05, 6.30904e-05, 6.31776e-05, 6.32499e-05, 6.33252e-05, 6.33897e-05, 6.34825e-05, 6.3551e-05, 6.3617e-05, 6.369e-05, 6.37444e-05, 6.38095e-05, 6.38784e-05, 6.39427e-05, 6.39972e-05, 6.40688e-05, 6.41211e-05, 6.41791e-05, 6.42275e-05, 6.42726e-05, 6.43288e-05, 6.43804e-05, 6.44342e-05, 6.4483e-05, 6.45222e-05, 6.45785e-05, 6.46253e-05, 6.46769e-05, 6.47199e-05, 6.47628e-05, 6.4815e-05, 6.48532e-05, 6.4902e-05, 6.49498e-05, 6.499e-05, 6.50361e-05, 6.50731e-05, 6.51101e-05, 6.51598e-05, 6.52074e-05, 6.52407e-05, 6.52839e-05, 6.53239e-05, 6.53584e-05, 6.54017e-05, 6.54404e-05, 6.54804e-05, 6.55152e-05, 6.55558e-05, 6.55893e-05, 6.56254e-05, 6.56596e-05, 6.56946e-05, 6.57309e-05, 6.57716e-05, 6.58076e-05, 6.58379e-05, 6.58787e-05, 6.59124e-05, 6.59461e-05, 6.59773e-05, 6.59986e-05, 6.60355e-05, 6.60661e-05, 6.61005e-05, 6.61398e-05, 6.61734e-05, 6.62066e-05, 6.62397e-05, 6.62728e-05, 6.62953e-05, 6.63323e-05, 6.63739e-05, 6.63982e-05, 6.64207e-05, 6.64501e-05, 6.64861e-05, 6.65204e-05, 6.65435e-05, 6.65791e-05, 6.66053e-05, 6.66395e-05, 6.66631e-05, 6.66977e-05, 6.6725e-05, 6.6754e-05, 6.67812e-05, 6.68205e-05, 6.68498e-05, 6.68758e-05, 6.69066e-05, 6.69283e-05, 6.69588e-05, 6.6977e-05, 6.70125e-05, 6.70315e-05, 6.70621e-05, 6.70786e-05, 6.71142e-05, 6.71459e-05, 6.71679e-05, 6.71907e-05, 6.72193e-05, 6.72406e-05, 6.72611e-05, 6.72912e-05, 6.73133e-05, 6.73462e-05, 6.73678e-05, 6.73942e-05, 6.74228e-05, 6.74498e-05, 6.74745e-05, 6.75057e-05, 6.75224e-05, 6.75598e-05, 6.75799e-05, 6.76058e-05, 6.7626e-05, 6.76504e-05, 6.76706e-05, 6.7698e-05, 6.77274e-05, 6.77491e-05, 6.77722e-05, 6.7789e-05, 6.78309e-05, 6.7848e-05, 6.78757e-05, 6.78952e-05, 6.79262e-05, 6.79451e-05, 6.79681e-05, 6.79904e-05, 6.80134e-05, 6.80354e-05, 6.80772e-05, 6.8093e-05, 6.81142e-05, 6.81423e-05, 6.81666e-05, 6.81914e-05, 6.82122e-05, 6.82264e-05, 6.82485e-05, 6.82835e-05, 6.83046e-05, 6.83208e-05, 6.83457e-05, 6.83655e-05, 6.83779e-05, 6.84009e-05, 6.84344e-05]
  out "VD Array.":dbl[](array[numeric])=[0.0, 0.01, 0.02, 0.03, 0.04, 0.05, 0.060000000000000005, 0.07, 0.08, 0.09, 0.09999999999999999, 0.10999999999999999, 0.11999999999999998, 0.12999999999999998, 0.13999999999999999, 0.15, 0.16, 0.17, 0.18000000000000002, 0.19000000000000003, 0.20000000000000004, 0.21000000000000005, 0.22000000000000006, 0.23000000000000007, 0.24000000000000007, 0.25000000000000006, 0.26000000000000006, 0.2700000000000001, 0.2800000000000001, 0.2900000000000001, 0.3000000000000001, 0.3100000000000001, 0.3200000000000001, 0.3300000000000001, 0.34000000000000014, 0.35000000000000014, 0.36000000000000015, 0.37000000000000016, 0.38000000000000017, 0.3900000000000002, 0.4000000000000002, 0.4100000000000002, 0.4200000000000002, 0.4300000000000002, 0.4400000000000002, 0.45000000000000023, 0.46000000000000024, 0.47000000000000025, 0.48000000000000026, 0.49000000000000027, 0.5000000000000002, 0.5100000000000002, 0.5200000000000002, 0.5300000000000002, 0.5400000000000003, 0.5500000000000003, 0.5600000000000003, 0.5700000000000003, 0.5800000000000003, 0.5900000000000003, 0.6000000000000003, 0.6100000000000003, 0.6200000000000003, 0.6300000000000003, 0.6400000000000003, 0.6500000000000004, 0.6600000000000004, 0.6700000000000004, 0.6800000000000004, 0.6900000000000004, 0.7000000000000004, 0.7100000000000004, 0.7200000000000004, 0.7300000000000004, 0.7400000000000004, 0.7500000000000004, 0.7600000000000005, 0.7700000000000005, 0.7800000000000005, 0.7900000000000005, 0.8000000000000005, 0.8100000000000005, 0.8200000000000005, 0.8300000000000005, 0.8400000000000005, 0.8500000000000005, 0.8600000000000005, 0.8700000000000006, 0.8800000000000006, 0.8900000000000006, 0.9000000000000006, 0.9100000000000006, 0.9200000000000006, 0.9300000000000006, 0.9400000000000006, 0.9500000000000006, 0.9600000000000006, 0.9700000000000006, 0.9800000000000006, 0.9900000000000007, 1.0000000000000007, 1.0100000000000007, 1.0200000000000007, 1.0300000000000007, 1.0400000000000007, 1.0500000000000007, 1.0600000000000007, 1.0700000000000007, 1.0800000000000007, 1.0900000000000007, 1.1000000000000008, 1.1100000000000008, 1.1200000000000008, 1.1300000000000008, 1.1400000000000008, 1.1500000000000008, 1.1600000000000008, 1.1700000000000008, 1.1800000000000008, 1.1900000000000008, 1.2000000000000008, 1.2100000000000009, 1.2200000000000009, 1.2300000000000009, 1.2400000000000009, 1.2500000000000009, 1.260000000000001, 1.270000000000001, 1.280000000000001, 1.290000000000001, 1.300000000000001, 1.310000000000001, 1.320000000000001, 1.330000000000001, 1.340000000000001, 1.350000000000001, 1.360000000000001, 1.370000000000001, 1.380000000000001, 1.390000000000001, 1.400000000000001, 1.410000000000001, 1.420000000000001, 1.430000000000001, 1.440000000000001, 1.450000000000001, 1.460000000000001, 1.470000000000001, 1.480000000000001, 1.490000000000001, 1.500000000000001, 1.5100000000000011, 1.5200000000000011, 1.5300000000000011, 1.5400000000000011, 1.5500000000000012, 1.5600000000000012, 1.5700000000000012, 1.5800000000000012, 1.5900000000000012, 1.6000000000000012, 1.6100000000000012, 1.6200000000000012, 1.6300000000000012, 1.6400000000000012, 1.6500000000000012, 1.6600000000000013, 1.6700000000000013, 1.6800000000000013, 1.6900000000000013, 1.7000000000000013, 1.7100000000000013, 1.7200000000000013, 1.7300000000000013, 1.7400000000000013, 1.7500000000000013, 1.7600000000000013, 1.7700000000000014, 1.7800000000000014, 1.7900000000000014, 1.8000000000000014, 1.8100000000000014, 1.8200000000000014, 1.8300000000000014, 1.8400000000000014, 1.8500000000000014, 1.8600000000000014, 1.8700000000000014, 1.8800000000000014, 1.8900000000000015, 1.9000000000000015, 1.9100000000000015, 1.9200000000000015, 1.9300000000000015, 1.9400000000000015, 1.9500000000000015, 1.9600000000000015, 1.9700000000000015, 1.9800000000000015, 1.9900000000000015, 2.0000000000000013, 0.0, 0.01, 0.02, 0.03, 0.04, 0.05, 0.060000000000000005, 0.07, 0.08, 0.09, 0.09999999999999999, 0.10999999999999999, 0.11999999999999998, 0.12999999999999998, 0.13999999999999999, 0.15, 0.16, 0.17, 0.18000000000000002, 0.19000000000000003, 0.20000000000000004, 0.21000000000000005, 0.22000000000000006, 0.23000000000000007, 0.24000000000000007, 0.25000000000000006, 0.26000000000000006, 0.2700000000000001, 0.2800000000000001, 0.2900000000000001, 0.3000000000000001, 0.3100000000000001, 0.3200000000000001, 0.3300000000000001, 0.34000000000000014, 0.35000000000000014, 0.36000000000000015, 0.37000000000000016, 0.38000000000000017, 0.3900000000000002, 0.4000000000000002, 0.4100000000000002, 0.4200000000000002, 0.4300000000000002, 0.4400000000000002, 0.45000000000000023, 0.46000000000000024, 0.47000000000000025, 0.48000000000000026, 0.49000000000000027, 0.5000000000000002, 0.5100000000000002, 0.5200000000000002, 0.5300000000000002, 0.5400000000000003, 0.5500000000000003, 0.5600000000000003, 0.5700000000000003, 0.5800000000000003, 0.5900000000000003, 0.6000000000000003, 0.6100000000000003, 0.6200000000000003, 0.6300000000000003, 0.6400000000000003, 0.6500000000000004, 0.6600000000000004, 0.6700000000000004, 0.6800000000000004, 0.6900000000000004, 0.7000000000000004, 0.7100000000000004, 0.7200000000000004, 0.7300000000000004, 0.7400000000000004, 0.7500000000000004, 0.7600000000000005, 0.7700000000000005, 0.7800000000000005, 0.7900000000000005, 0.8000000000000005, 0.8100000000000005, 0.8200000000000005, 0.8300000000000005, 0.8400000000000005, 0.8500000000000005, 0.8600000000000005, 0.8700000000000006, 0.8800000000000006, 0.8900000000000006, 0.9000000000000006, 0.9100000000000006, 0.9200000000000006, 0.9300000000000006, 0.9400000000000006, 0.9500000000000006, 0.9600000000000006, 0.9700000000000006, 0.9800000000000006, 0.9900000000000007, 1.0000000000000007, 1.0100000000000007, 1.0200000000000007, 1.0300000000000007, 1.0400000000000007, 1.0500000000000007, 1.0600000000000007, 1.0700000000000007, 1.0800000000000007, 1.0900000000000007, 1.1000000000000008, 1.1100000000000008, 1.1200000000000008, 1.1300000000000008, 1.1400000000000008, 1.1500000000000008, 1.1600000000000008, 1.1700000000000008, 1.1800000000000008, 1.1900000000000008, 1.2000000000000008, 1.2100000000000009, 1.2200000000000009, 1.2300000000000009, 1.2400000000000009, 1.2500000000000009, 1.260000000000001, 1.270000000000001, 1.280000000000001, 1.290000000000001, 1.300000000000001, 1.310000000000001, 1.320000000000001, 1.330000000000001, 1.340000000000001, 1.350000000000001, 1.360000000000001, 1.370000000000001, 1.380000000000001, 1.390000000000001, 1.400000000000001, 1.410000000000001, 1.420000000000001, 1.430000000000001, 1.440000000000001, 1.450000000000001, 1.460000000000001, 1.470000000000001, 1.480000000000001, 1.490000000000001, 1.500000000000001, 1.5100000000000011, 1.5200000000000011, 1.5300000000000011, 1.5400000000000011, 1.5500000000000012, 1.5600000000000012, 1.5700000000000012, 1.5800000000000012, 1.5900000000000012, 1.6000000000000012, 1.6100000000000012, 1.6200000000000012, 1.6300000000000012, 1.6400000000000012, 1.6500000000000012, 1.6600000000000013, 1.6700000000000013, 1.6800000000000013, 1.6900000000000013, 1.7000000000000013, 1.7100000000000013, 1.7200000000000013, 1.7300000000000013, 1.7400000000000013, 1.7500000000000013, 1.7600000000000013, 1.7700000000000014, 1.7800000000000014, 1.7900000000000014, 1.8000000000000014, 1.8100000000000014, 1.8200000000000014, 1.8300000000000014, 1.8400000000000014, 1.8500000000000014, 1.8600000000000014, 1.8700000000000014, 1.8800000000000014, 1.8900000000000015, 1.9000000000000015, 1.9100000000000015, 1.9200000000000015, 1.9300000000000015, 1.9400000000000015, 1.9500000000000015, 1.9600000000000015, 1.9700000000000015, 1.9800000000000015, 1.9900000000000015, 2.0000000000000013, 0.0, 0.01, 0.02, 0.03, 0.04, 0.05, 0.060000000000000005, 0.07, 0.08, 0.09, 0.09999999999999999, 0.10999999999999999, 0.11999999999999998, 0.12999999999999998, 0.13999999999999999, 0.15, 0.16, 0.17, 0.18000000000000002, 0.19000000000000003, 0.20000000000000004, 0.21000000000000005, 0.22000000000000006, 0.23000000000000007, 0.24000000000000007, 0.25000000000000006, 0.26000000000000006, 0.2700000000000001, 0.2800000000000001, 0.2900000000000001, 0.3000000000000001, 0.3100000000000001, 0.3200000000000001, 0.3300000000000001, 0.34000000000000014, 0.35000000000000014, 0.36000000000000015, 0.37000000000000016, 0.38000000000000017, 0.3900000000000002, 0.4000000000000002, 0.4100000000000002, 0.4200000000000002, 0.4300000000000002, 0.4400000000000002, 0.45000000000000023, 0.46000000000000024, 0.47000000000000025, 0.48000000000000026, 0.49000000000000027, 0.5000000000000002, 0.5100000000000002, 0.5200000000000002, 0.5300000000000002, 0.5400000000000003, 0.5500000000000003, 0.5600000000000003, 0.5700000000000003, 0.5800000000000003, 0.5900000000000003, 0.6000000000000003, 0.6100000000000003, 0.6200000000000003, 0.6300000000000003, 0.6400000000000003, 0.6500000000000004, 0.6600000000000004, 0.6700000000000004, 0.6800000000000004, 0.6900000000000004, 0.7000000000000004, 0.7100000000000004, 0.7200000000000004, 0.7300000000000004, 0.7400000000000004, 0.7500000000000004, 0.7600000000000005, 0.7700000000000005, 0.7800000000000005, 0.7900000000000005, 0.8000000000000005, 0.8100000000000005, 0.8200000000000005, 0.8300000000000005, 0.8400000000000005, 0.8500000000000005, 0.8600000000000005, 0.8700000000000006, 0.8800000000000006, 0.8900000000000006, 0.9000000000000006, 0.9100000000000006, 0.9200000000000006, 0.9300000000000006, 0.9400000000000006, 0.9500000000000006, 0.9600000000000006, 0.9700000000000006, 0.9800000000000006, 0.9900000000000007, 1.0000000000000007, 1.0100000000000007, 1.0200000000000007, 1.0300000000000007, 1.0400000000000007, 1.0500000000000007, 1.0600000000000007, 1.0700000000000007, 1.0800000000000007, 1.0900000000000007, 1.1000000000000008, 1.1100000000000008, 1.1200000000000008, 1.1300000000000008, 1.1400000000000008, 1.1500000000000008, 1.1600000000000008, 1.1700000000000008, 1.1800000000000008, 1.1900000000000008, 1.2000000000000008, 1.2100000000000009, 1.2200000000000009, 1.2300000000000009, 1.2400000000000009, 1.2500000000000009, 1.260000000000001, 1.270000000000001, 1.280000000000001, 1.290000000000001, 1.300000000000001, 1.310000000000001, 1.320000000000001, 1.330000000000001, 1.340000000000001, 1.350000000000001, 1.360000000000001, 1.370000000000001, 1.380000000000001, 1.390000000000001, 1.400000000000001, 1.410000000000001, 1.420000000000001, 1.430000000000001, 1.440000000000001, 1.450000000000001, 1.460000000000001, 1.470000000000001, 1.480000000000001, 1.490000000000001, 1.500000000000001, 1.5100000000000011, 1.5200000000000011, 1.5300000000000011, 1.5400000000000011, 1.5500000000000012, 1.5600000000000012, 1.5700000000000012, 1.5800000000000012, 1.5900000000000012, 1.6000000000000012, 1.6100000000000012, 1.6200000000000012, 1.6300000000000012, 1.6400000000000012, 1.6500000000000012, 1.6600000000000013, 1.6700000000000013, 1.6800000000000013, 1.6900000000000013, 1.7000000000000013, 1.7100000000000013, 1.7200000000000013, 1.7300000000000013, 1.7400000000000013, 1.7500000000000013, 1.7600000000000013, 1.7700000000000014, 1.7800000000000014, 1.7900000000000014, 1.8000000000000014, 1.8100000000000014, 1.8200000000000014, 1.8300000000000014, 1.8400000000000014, 1.8500000000000014, 1.8600000000000014, 1.8700000000000014, 1.8800000000000014, 1.8900000000000015, 1.9000000000000015, 1.9100000000000015, 1.9200000000000015, 1.9300000000000015, 1.9400000000000015, 1.9500000000000015, 1.9600000000000015, 1.9700000000000015, 1.9800000000000015, 1.9900000000000015, 2.0000000000000013, 0.0, 0.01, 0.02, 0.03, 0.04, 0.05, 0.060000000000000005, 0.07, 0.08, 0.09, 0.09999999999999999, 0.10999999999999999, 0.11999999999999998, 0.12999999999999998, 0.13999999999999999, 0.15, 0.16, 0.17, 0.18000000000000002, 0.19000000000000003, 0.20000000000000004, 0.21000000000000005, 0.22000000000000006, 0.23000000000000007, 0.24000000000000007, 0.25000000000000006, 0.26000000000000006, 0.2700000000000001, 0.2800000000000001, 0.2900000000000001, 0.3000000000000001, 0.3100000000000001, 0.3200000000000001, 0.3300000000000001, 0.34000000000000014, 0.35000000000000014, 0.36000000000000015, 0.37000000000000016, 0.38000000000000017, 0.3900000000000002, 0.4000000000000002, 0.4100000000000002, 0.4200000000000002, 0.4300000000000002, 0.4400000000000002, 0.45000000000000023, 0.46000000000000024, 0.47000000000000025, 0.48000000000000026, 0.49000000000000027, 0.5000000000000002, 0.5100000000000002, 0.5200000000000002, 0.5300000000000002, 0.5400000000000003, 0.5500000000000003, 0.5600000000000003, 0.5700000000000003, 0.5800000000000003, 0.5900000000000003, 0.6000000000000003, 0.6100000000000003, 0.6200000000000003, 0.6300000000000003, 0.6400000000000003, 0.6500000000000004, 0.6600000000000004, 0.6700000000000004, 0.6800000000000004, 0.6900000000000004, 0.7000000000000004, 0.7100000000000004, 0.7200000000000004, 0.7300000000000004, 0.7400000000000004, 0.7500000000000004, 0.7600000000000005, 0.7700000000000005, 0.7800000000000005, 0.7900000000000005, 0.8000000000000005, 0.8100000000000005, 0.8200000000000005, 0.8300000000000005, 0.8400000000000005, 0.8500000000000005, 0.8600000000000005, 0.8700000000000006, 0.8800000000000006, 0.8900000000000006, 0.9000000000000006, 0.9100000000000006, 0.9200000000000006, 0.9300000000000006, 0.9400000000000006, 0.9500000000000006, 0.9600000000000006, 0.9700000000000006, 0.9800000000000006, 0.9900000000000007, 1.0000000000000007, 1.0100000000000007, 1.0200000000000007, 1.0300000000000007, 1.0400000000000007, 1.0500000000000007, 1.0600000000000007, 1.0700000000000007, 1.0800000000000007, 1.0900000000000007, 1.1000000000000008, 1.1100000000000008, 1.1200000000000008, 1.1300000000000008, 1.1400000000000008, 1.1500000000000008, 1.1600000000000008, 1.1700000000000008, 1.1800000000000008, 1.1900000000000008, 1.2000000000000008, 1.2100000000000009, 1.2200000000000009, 1.2300000000000009, 1.2400000000000009, 1.2500000000000009, 1.260000000000001, 1.270000000000001, 1.280000000000001, 1.290000000000001, 1.300000000000001, 1.310000000000001, 1.320000000000001, 1.330000000000001, 1.340000000000001, 1.350000000000001, 1.360000000000001, 1.370000000000001, 1.380000000000001, 1.390000000000001, 1.400000000000001, 1.410000000000001, 1.420000000000001, 1.430000000000001, 1.440000000000001, 1.450000000000001, 1.460000000000001, 1.470000000000001, 1.480000000000001, 1.490000000000001, 1.500000000000001, 1.5100000000000011, 1.5200000000000011, 1.5300000000000011, 1.5400000000000011, 1.5500000000000012, 1.5600000000000012, 1.5700000000000012, 1.5800000000000012, 1.5900000000000012, 1.6000000000000012, 1.6100000000000012, 1.6200000000000012, 1.6300000000000012, 1.6400000000000012, 1.6500000000000012, 1.6600000000000013, 1.6700000000000013, 1.6800000000000013, 1.6900000000000013, 1.7000000000000013, 1.7100000000000013, 1.7200000000000013, 1.7300000000000013, 1.7400000000000013, 1.7500000000000013, 1.7600000000000013, 1.7700000000000014, 1.7800000000000014, 1.7900000000000014, 1.8000000000000014, 1.8100000000000014, 1.8200000000000014, 1.8300000000000014, 1.8400000000000014, 1.8500000000000014, 1.8600000000000014, 1.8700000000000014, 1.8800000000000014, 1.8900000000000015, 1.9000000000000015, 1.9100000000000015, 1.9200000000000015, 1.9300000000000015, 1.9400000000000015, 1.9500000000000015, 1.9600000000000015, 1.9700000000000015, 1.9800000000000015, 1.9900000000000015, 2.0000000000000013, 0.0, 0.01, 0.02, 0.03, 0.04, 0.05, 0.060000000000000005, 0.07, 0.08, 0.09, 0.09999999999999999, 0.10999999999999999, 0.11999999999999998, 0.12999999999999998, 0.13999999999999999, 0.15, 0.16, 0.17, 0.18000000000000002, 0.19000000000000003, 0.20000000000000004, 0.21000000000000005, 0.22000000000000006, 0.23000000000000007, 0.24000000000000007, 0.25000000000000006, 0.26000000000000006, 0.2700000000000001, 0.2800000000000001, 0.2900000000000001, 0.3000000000000001, 0.3100000000000001, 0.3200000000000001, 0.3300000000000001, 0.34000000000000014, 0.35000000000000014, 0.36000000000000015, 0.37000000000000016, 0.38000000000000017, 0.3900000000000002, 0.4000000000000002, 0.4100000000000002, 0.4200000000000002, 0.4300000000000002, 0.4400000000000002, 0.45000000000000023, 0.46000000000000024, 0.47000000000000025, 0.48000000000000026, 0.49000000000000027, 0.5000000000000002, 0.5100000000000002, 0.5200000000000002, 0.5300000000000002, 0.5400000000000003, 0.5500000000000003, 0.5600000000000003, 0.5700000000000003, 0.5800000000000003, 0.5900000000000003, 0.6000000000000003, 0.6100000000000003, 0.6200000000000003, 0.6300000000000003, 0.6400000000000003, 0.6500000000000004, 0.6600000000000004, 0.6700000000000004, 0.6800000000000004, 0.6900000000000004, 0.7000000000000004, 0.7100000000000004, 0.7200000000000004, 0.7300000000000004, 0.7400000000000004, 0.7500000000000004, 0.7600000000000005, 0.7700000000000005, 0.7800000000000005, 0.7900000000000005, 0.8000000000000005, 0.8100000000000005, 0.8200000000000005, 0.8300000000000005, 0.8400000000000005, 0.8500000000000005, 0.8600000000000005, 0.8700000000000006, 0.8800000000000006, 0.8900000000000006, 0.9000000000000006, 0.9100000000000006, 0.9200000000000006, 0.9300000000000006, 0.9400000000000006, 0.9500000000000006, 0.9600000000000006, 0.9700000000000006, 0.9800000000000006, 0.9900000000000007, 1.0000000000000007, 1.0100000000000007, 1.0200000000000007, 1.0300000000000007, 1.0400000000000007, 1.0500000000000007, 1.0600000000000007, 1.0700000000000007, 1.0800000000000007, 1.0900000000000007, 1.1000000000000008, 1.1100000000000008, 1.1200000000000008, 1.1300000000000008, 1.1400000000000008, 1.1500000000000008, 1.1600000000000008, 1.1700000000000008, 1.1800000000000008, 1.1900000000000008, 1.2000000000000008, 1.2100000000000009, 1.2200000000000009, 1.2300000000000009, 1.2400000000000009, 1.2500000000000009, 1.260000000000001, 1.270000000000001, 1.280000000000001, 1.290000000000001, 1.300000000000001, 1.310000000000001, 1.320000000000001, 1.330000000000001, 1.340000000000001, 1.350000000000001, 1.360000000000001, 1.370000000000001, 1.380000000000001, 1.390000000000001, 1.400000000000001, 1.410000000000001, 1.420000000000001, 1.430000000000001, 1.440000000000001, 1.450000000000001, 1.460000000000001, 1.470000000000001, 1.480000000000001, 1.490000000000001, 1.500000000000001, 1.5100000000000011, 1.5200000000000011, 1.5300000000000011, 1.5400000000000011, 1.5500000000000012, 1.5600000000000012, 1.5700000000000012, 1.5800000000000012, 1.5900000000000012, 1.6000000000000012, 1.6100000000000012, 1.6200000000000012, 1.6300000000000012, 1.6400000000000012, 1.6500000000000012, 1.6600000000000013, 1.6700000000000013, 1.6800000000000013, 1.6900000000000013, 1.7000000000000013, 1.7100000000000013, 1.7200000000000013, 1.7300000000000013, 1.7400000000000013, 1.7500000000000013, 1.7600000000000013, 1.7700000000000014, 1.7800000000000014, 1.7900000000000014, 1.8000000000000014, 1.8100000000000014, 1.8200000000000014, 1.8300000000000014, 1.8400000000000014, 1.8500000000000014, 1.8600000000000014, 1.8700000000000014, 1.8800000000000014, 1.8900000000000015, 1.9000000000000015, 1.9100000000000015, 1.9200000000000015, 1.9300000000000015, 1.9400000000000015, 1.9500000000000015, 1.9600000000000015, 1.9700000000000015, 1.9800000000000015, 1.9900000000000015, 2.0000000000000013]
  in  "Gate comp [V].":dbl=0.001 format="%#_6e"
  in  "Gate SMU no.":dbl=1.0
  out "VD vs. ID":cluster{"Y":dbl[], "Y":dbl[]}[](graph)
  in  "Drain comp [V].":dbl=0.001 format="%#_6e"
  in  "Drain SMU no.":dbl=2.0
  out "Drain current":dbl=6.84344e-05 format="%#_6e"
  out "VD.":dbl=2.0000000000000013
  in  "Hysteresis.":bool
  in  "VD step [V]":dbl=0.01
  in  "VD stop [V]":dbl=2.0
  in  "VD start [V]":dbl
  # "Gate Voltage Set"
  # "Parameter indicator"
  # "MOSFET Parameter"
  # "Resource Control"
  # "Drain&Source"
  # "Compliance"
  # "Switch Controllor"
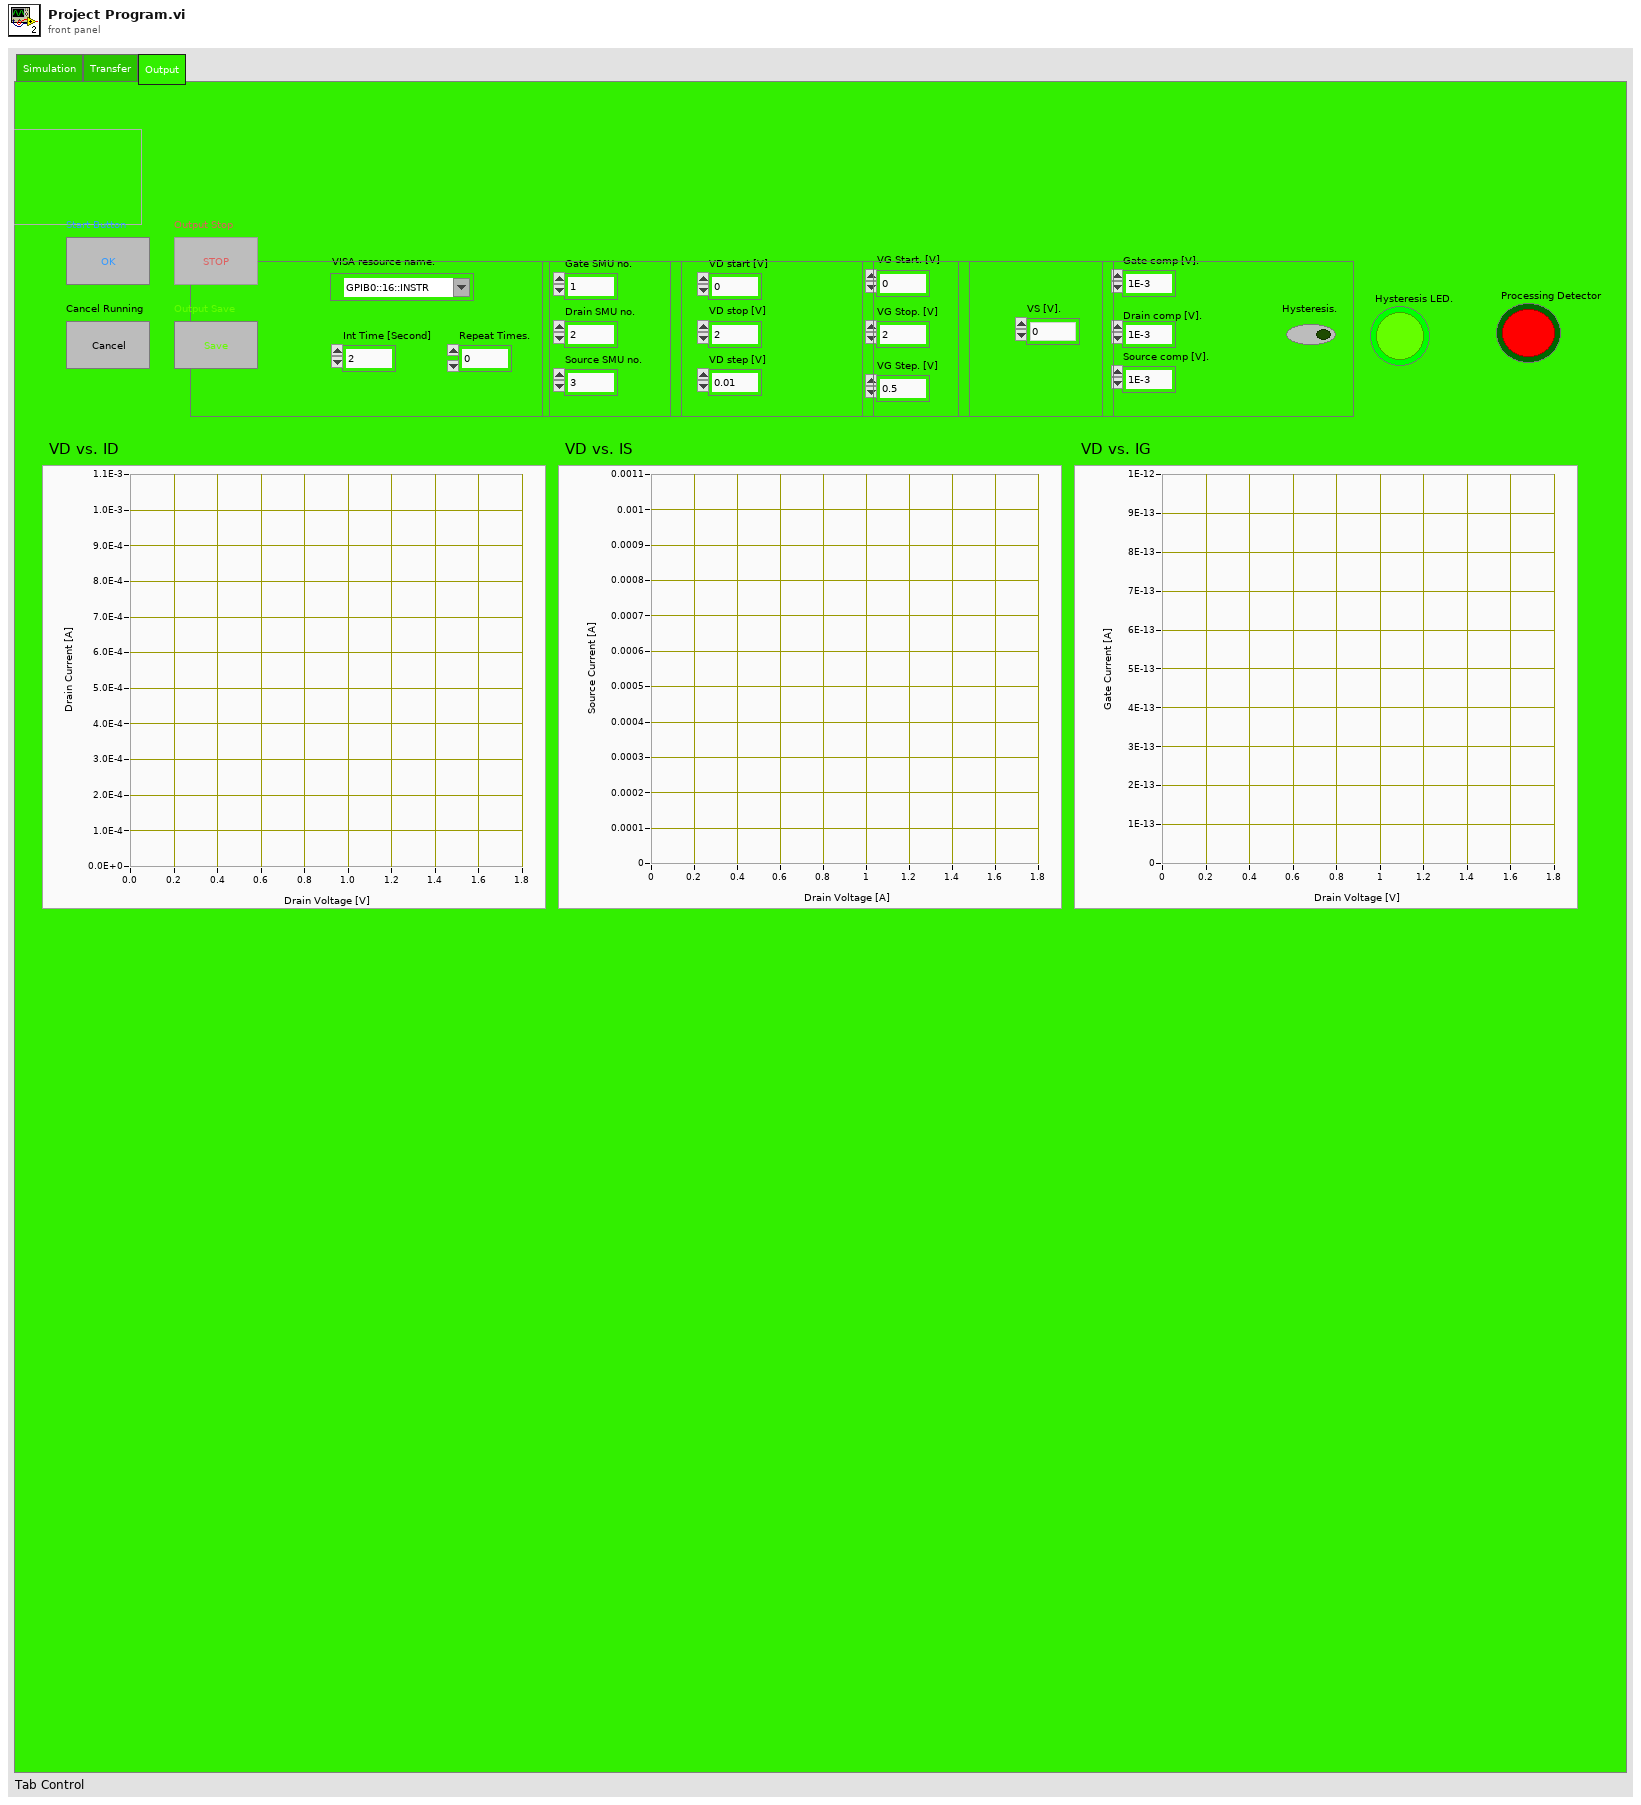
[diagram p1: front panel]
types:
  T1 = enum16{"_Quit_", "Init", "Waiting", "Measuring", "Stop", "Save", "Exit"}
  T2 = enum16{"_Quit_", "Init", "Waiting", "Measuring", "Saving", "Stopping", "Exit"}
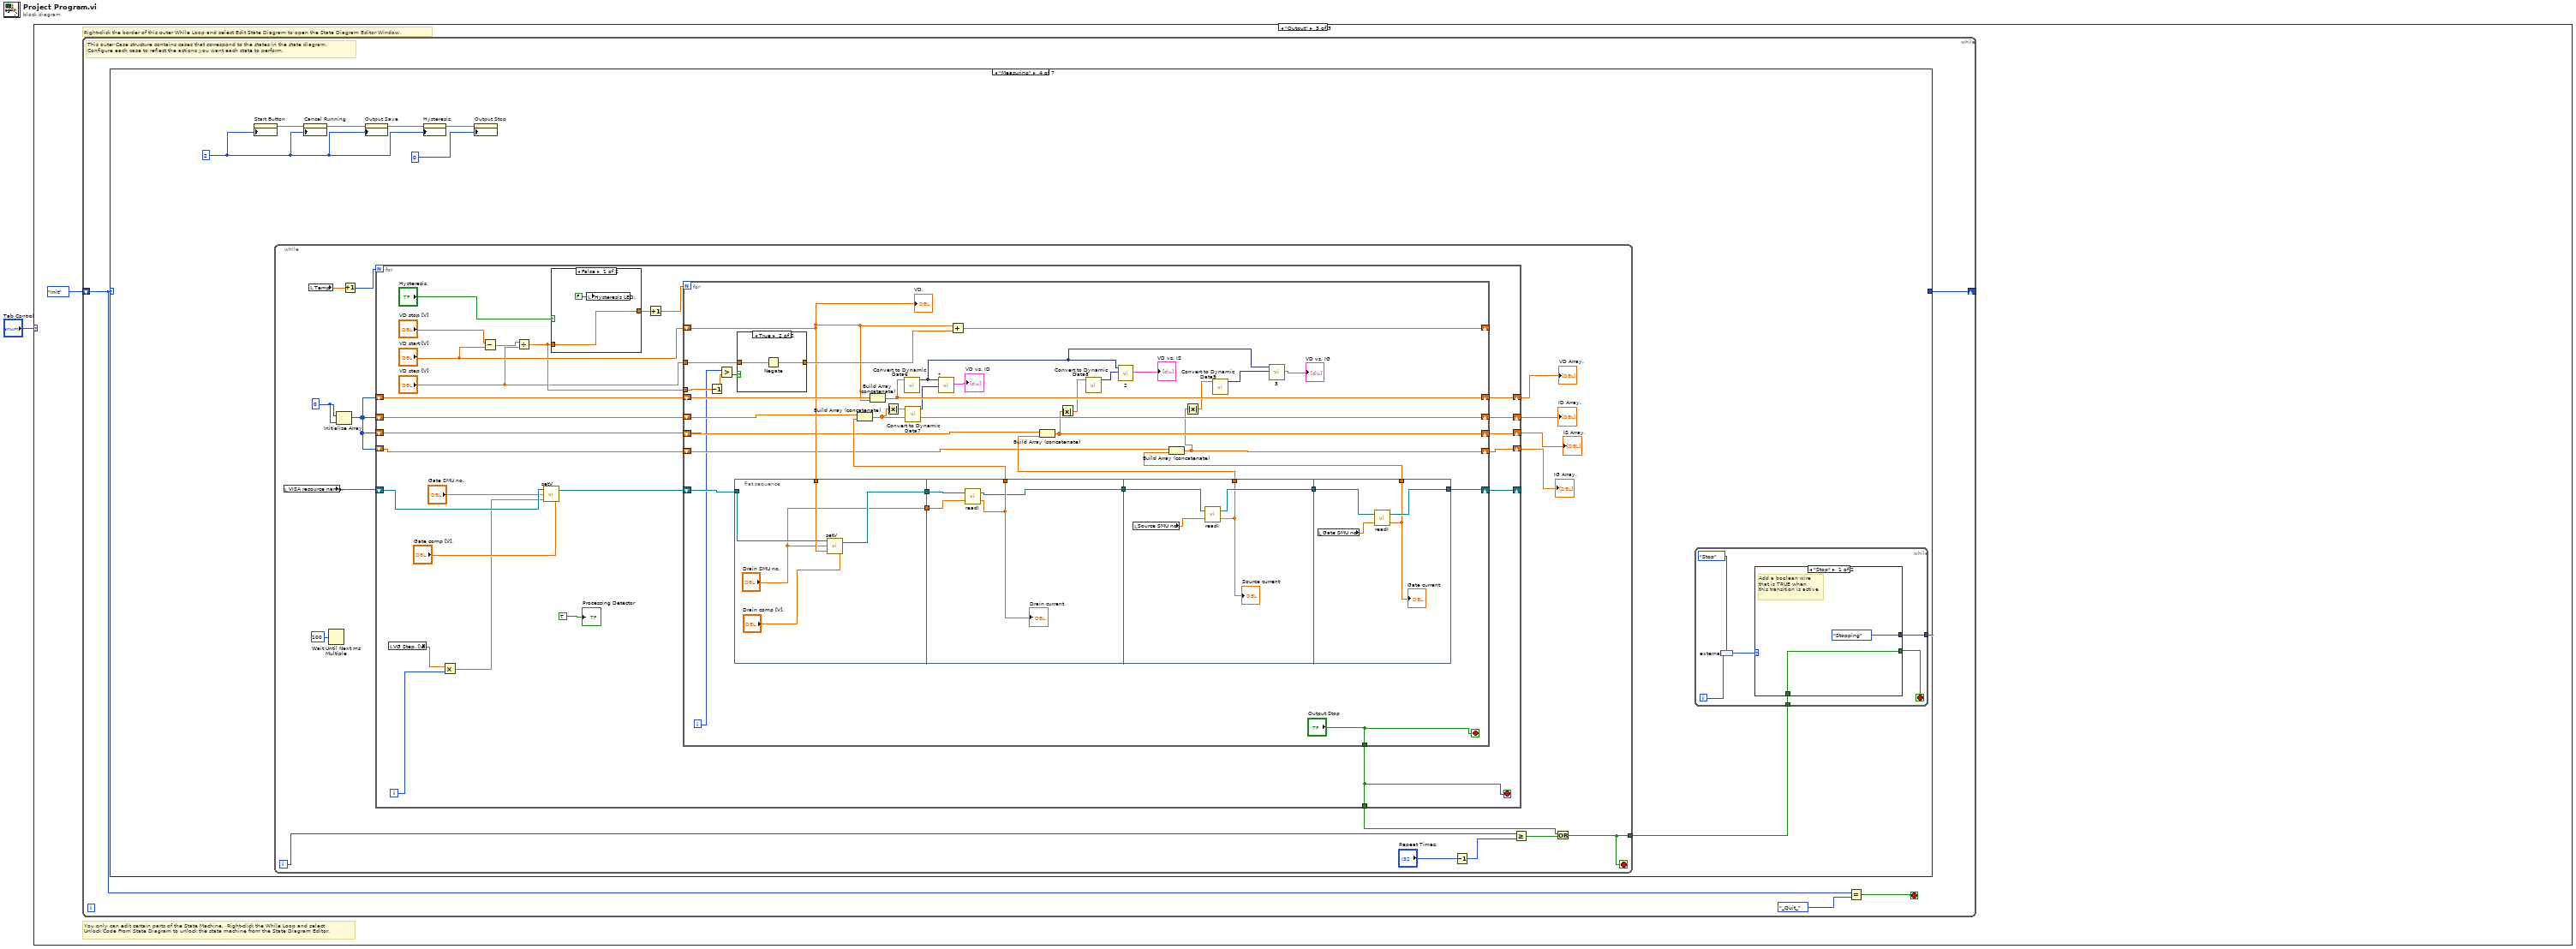
[diagram p0: block diagram]
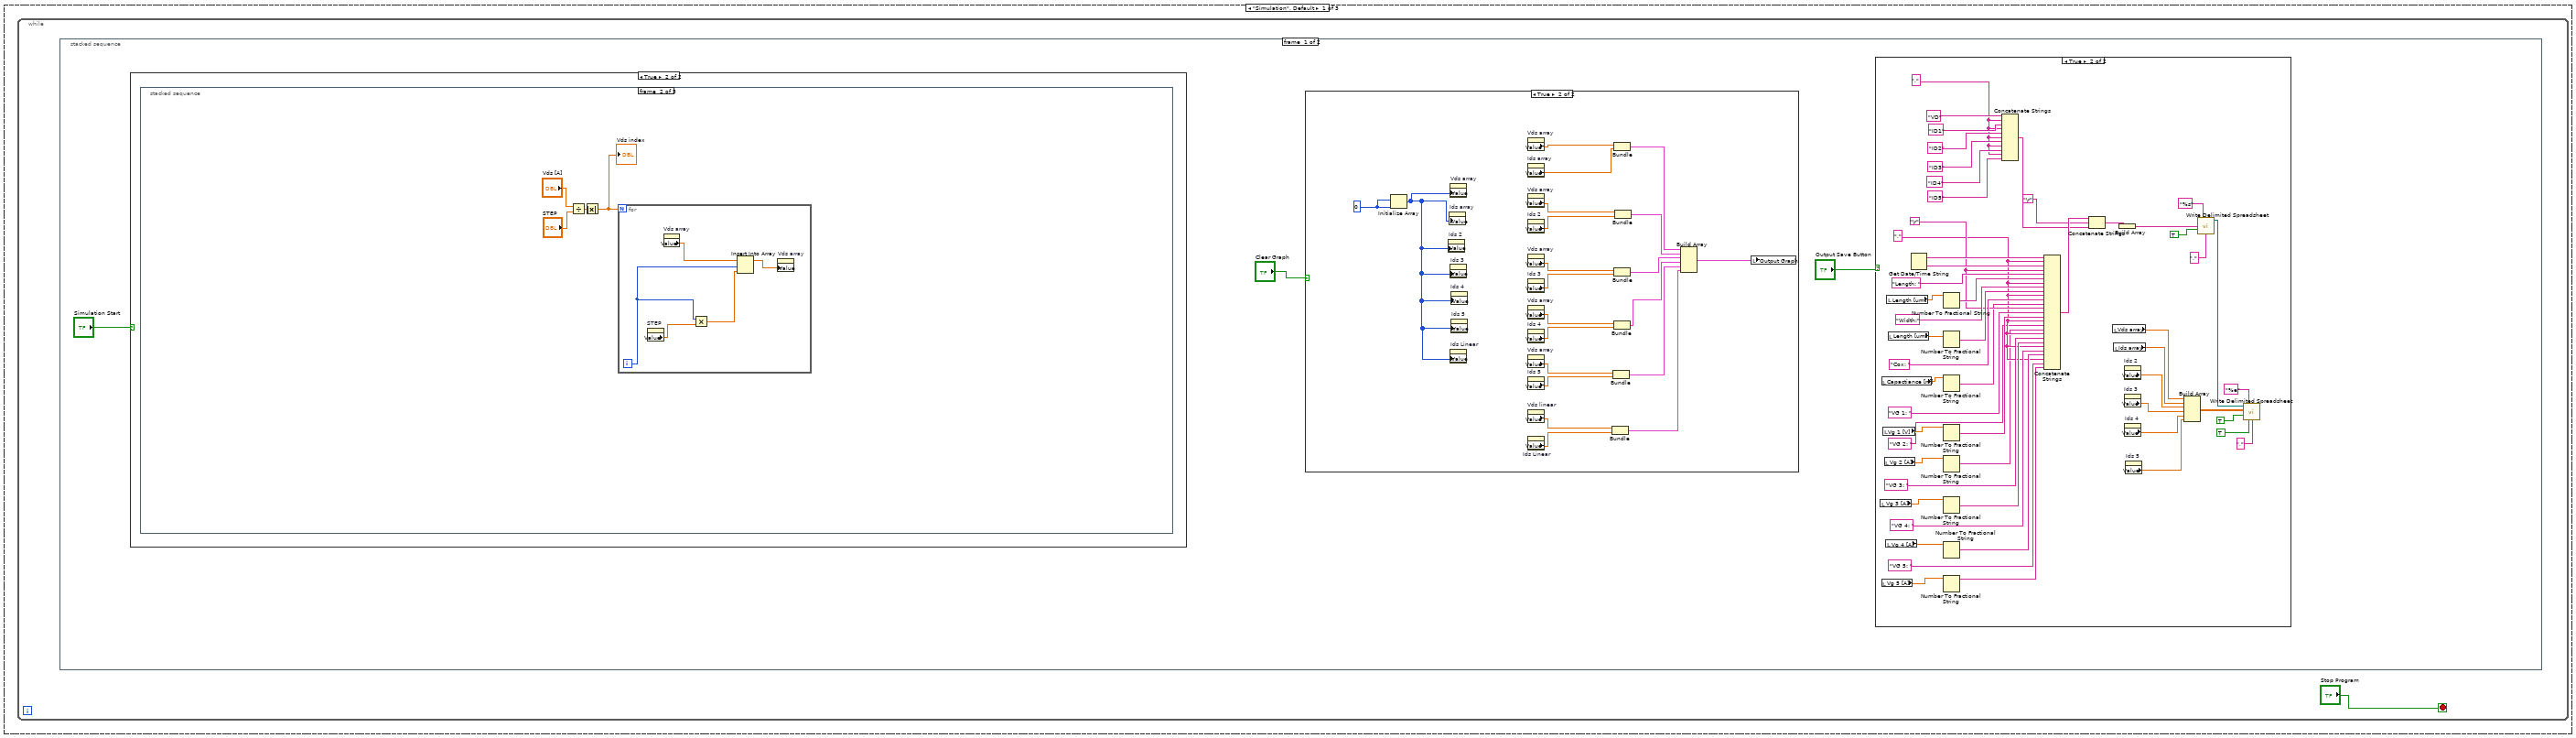
[diagram p2: hidden frame]
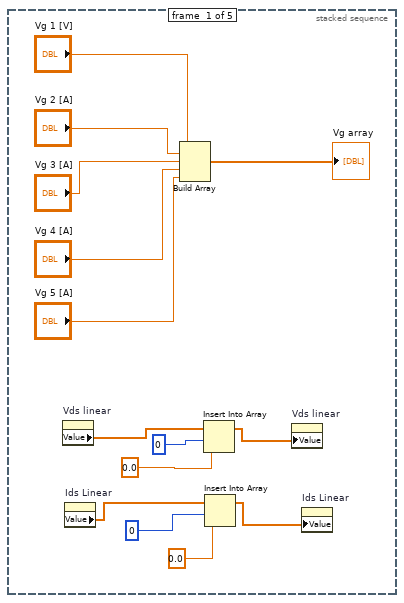
[diagram p6: hidden frame]
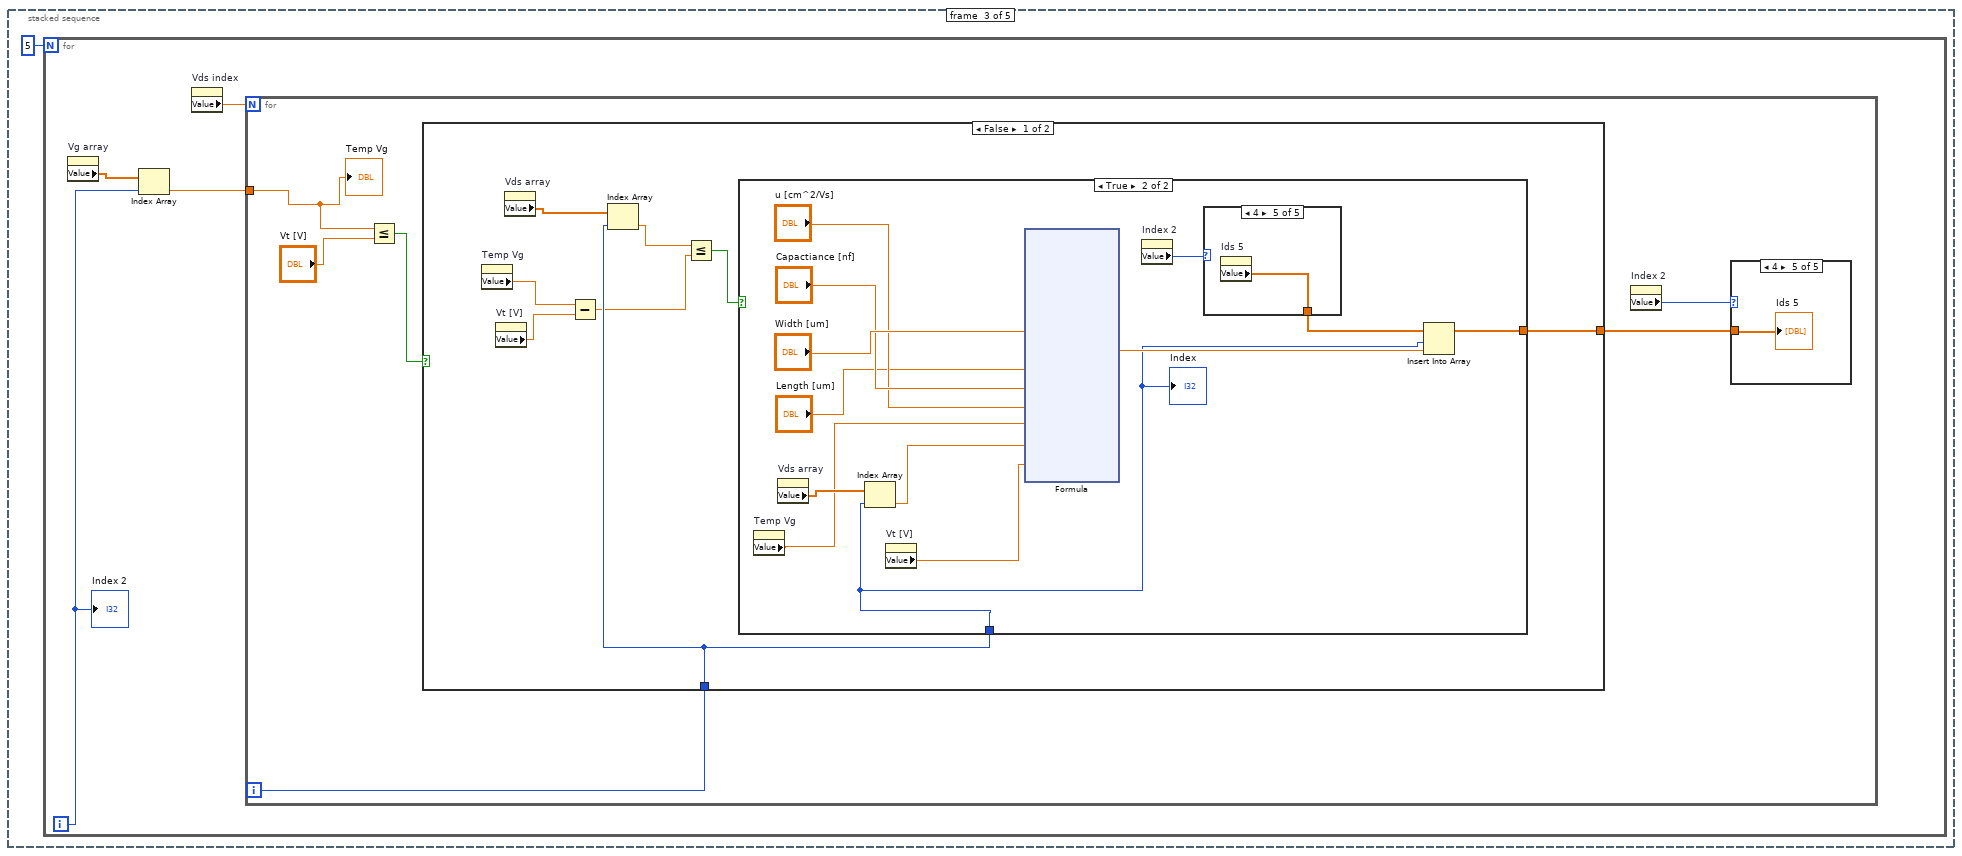
[diagram p7: hidden frame]
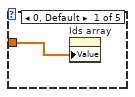
[diagram p8: hidden frame]
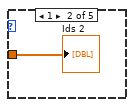
[diagram p9: hidden frame]
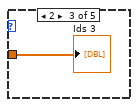
[diagram p10: hidden frame]
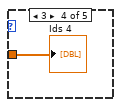
[diagram p11: hidden frame]
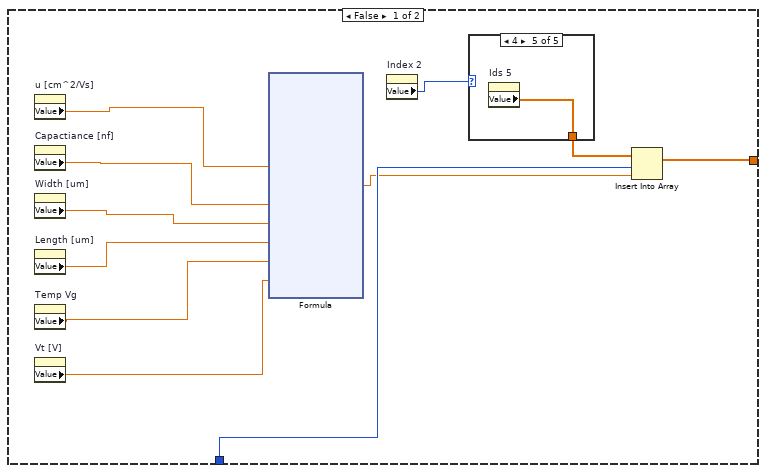
[diagram p12: hidden frame]
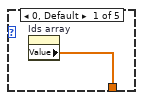
[diagram p13: hidden frame]
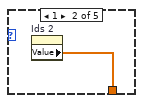
[diagram p14: hidden frame]
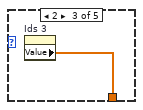
[diagram p15: hidden frame]
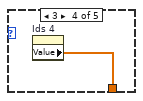
[diagram p16: hidden frame]
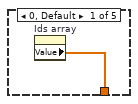
[diagram p17: hidden frame]
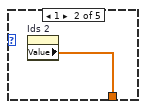
[diagram p18: hidden frame]
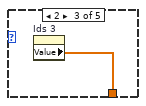
[diagram p19: hidden frame]
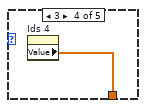
[diagram p20: hidden frame]
diagram:
  n1 = case shown="\"Output\"" "Tab Control" {
    frame "Simulation", Default {
      n2 = while {
        stop <- "Stop Program" stop-if-true
        n3 = stacked-sequence {
          frame #0 {
            n4 = case shown="True" "Simulation Start" {
              frame False {
              }
              frame True {
                n5 = stacked-sequence {
                  frame #0 {
                    n6 = property on="Vds linear" class="Arr (strict)"() -> ("Value"=w90:dbl[])  [unwired: 2 in, 2 out]
                    n7 = property on="Ids Linear" class="Arr (strict)"() -> ("Value"=w86:dbl[])  [unwired: 2 in, 2 out]
                    n8 = Build Array("Vg 1 [V]", "Vg 2 [A]", "Vg 3 [A]", "Vg 4 [A]", "Vg 5 [A]") -> (→"Vg array":dbl[])
                    n9 = Insert Into Array(array=w90, index=0, new element=0.0 ("new element/subarray")) -> (w87:dbl[])
                    n10 = Insert Into Array(array=w86, index=0, new element=0.0 ("new element/subarray")) -> (w83:dbl[])
                    n11 = property on="Vds linear" class="Arr (strict)"("Value"=w87) -> ()  [unwired: 2 in, 2 out]
                    n12 = property on="Ids Linear" class="Arr (strict)"("Value"=w83) -> ()  [unwired: 2 in, 2 out]
                  }
                  frame #1 {
                    n13 = Divide(x="Vds [A]", y="STEP") -> (x/y=w97:dbl)
                    n14 = Absolute Value(x=w97) -> (abs(x)=w96:dbl)
                    "Vds index" <- w96
                    n15 = for {
                      N: w96 -> [_]
                      i -> [w102]
                      n16 = property on="STEP" class="DigNum (strict)"() -> ("Value"=w103:dbl)  [unwired: 2 in, 2 out]
                      n17 = property on="Vds array" class="Arr (strict)"() -> ("Value"=w104:dbl[])  [unwired: 2 in, 2 out]
                      n18 = Multiply(x=w102, y=w103) -> (x*y=w101:dbl)
                      n19 = Insert Into Array(array=w104, index=w102, new element=w101) -> (w100:dbl[])
                      n20 = property on="Vds array" class="Arr (strict)"("Value"=w100) -> ()  [unwired: 2 in, 2 out]
                    }
                  }
                  frame #2 {
                    n21 = for {
                      N: 5 -> [_]
                      i -> [w107]
                      n22 = property on="Vg array" class="Arr (strict)"() -> ("Value"=w108:dbl[])  [unwired: 2 in, 2 out]
                      n23 = Index Array(array=w108, index=w107) -> (element=w106:dbl)
                      n24 = property on="Vds index" class="DigNum (strict)"() -> ("Value"=w109:dbl)  [unwired: 2 in, 2 out]
                      n25 = for {
                        N: w109 -> [_]
                        tunnel: w106 -> [w111]
                        i -> [w115]
                        n26 = Less Or Equal?(x=w111, y="Vt [V]") -> (x <= y?=w113:bool)
                        n27 = case shown="False" w113 {
                          tunnel: w115 -> [w125 w203]
                          tunnel: [w121 w201] -> w110
                          frame False {
                            n28 = property on="Temp Vg" class="DigNum (strict)"() -> ("Value"=w124:dbl)  [unwired: 2 in, 2 out]
                            n29 = property on="Vt [V]" class="DigNum (strict)"() -> ("Value"=w127:dbl)  [unwired: 2 in, 2 out]
                            n30 = property on="Vds array" class="Arr (strict)"() -> ("Value"=w126:dbl[])  [unwired: 2 in, 2 out]
                            n31 = Subtract(x=w124, y=w127) -> (x-y=w122:dbl)
                            n32 = Index Array(array=w126, index=w125) -> (element=w123:dbl)
                            n33 = Less Or Equal?(x=w123, y=w122) -> (x <= y?=w128:bool)
                            n34 = case shown="True" w128 {
                              tunnel: w125 -> [w133 w166]
                              tunnel: [w134 w167] -> w121
                              frame False {
                                n35 = property on="u [cm^2/Vs]" class="DigNum (strict)"() -> ("Value"=w139:dbl)  [unwired: 2 in, 2 out]
                                n36 = property on="Capactiance [nf]" class="DigNum (strict)"() -> ("Value"=w138:dbl)  [unwired: 2 in, 2 out]
                                n37 = property on="Width [um]" class="DigNum (strict)"() -> ("Value"=w137:dbl)  [unwired: 2 in, 2 out]
                                n38 = property on="Length [um]" class="DigNum (strict)"() -> ("Value"=w136:dbl)  [unwired: 2 in, 2 out]
                                n39 = property on="Temp Vg" class="DigNum (strict)"() -> ("Value"=w132:dbl)  [unwired: 2 in, 2 out]
                                n40 = property on="Vt [V]" class="DigNum (strict)"() -> ("Value"=w135:dbl)  [unwired: 2 in, 2 out]
                                n41 = xnode "Formula"("u"=w139, "Cox"=w138, "W"=w137, "L"=w136, "Vg"=w132, "Vt"=w135) -> ("Result"=w129:dbl)  [unwired: 1 in, 1 out]
                                n42 = property on="Index 2" class="DigNum (strict)"() -> ("Value"=w131:i32)  [unwired: 2 in, 2 out]
                                n43 = case shown="4" w131 {
                                tunnel: [w140 w141 w142 w143 w144] -> w130
                                frame 0, Default {
                                n44 = property on="Ids array" class="Arr (strict)"() -> ("Value"=w140:dbl[])  [unwired: 2 in, 2 out]
                                }
                                frame 1 {
                                n45 = property on="Ids 2" class="Arr (strict)"() -> ("Value"=w141:dbl[])  [unwired: 2 in, 2 out]
                                }
                                frame 2 {
                                n46 = property on="Ids 3" class="Arr (strict)"() -> ("Value"=w142:dbl[])  [unwired: 2 in, 2 out]
                                }
                                frame 3 {
                                n47 = property on="Ids 4" class="Arr (strict)"() -> ("Value"=w143:dbl[])  [unwired: 2 in, 2 out]
                                }
                                frame 4 {
                                n48 = property on="Ids 5" class="Arr (strict)"() -> ("Value"=w144:dbl[])  [unwired: 2 in, 2 out]
                                }
                                }
                                n49 = Insert Into Array(array=w130, index=w133, new element=w129) -> (w134:dbl[])
                              }
                              frame True {
                                n50 = property on="Temp Vg" class="DigNum (strict)"() -> ("Value"=w165:dbl)  [unwired: 2 in, 2 out]
                                n51 = property on="Vds array" class="Arr (strict)"() -> ("Value"=w175:dbl[])  [unwired: 2 in, 2 out]
                                n52 = Index Array(array=w175, index=w166) -> (element=w170:dbl)
                                n53 = property on="Vt [V]" class="DigNum (strict)"() -> ("Value"=w169:dbl)  [unwired: 2 in, 2 out]
                                n54 = xnode "Formula"("W"="Width [um]", "L"="Length [um]", "Cox"="Capactiance [nf]", "u"="u [cm^2/Vs]", "Vg"=w165, "Vd"=w170, "Vt"=w169) -> ("Result"=w168:dbl)  [unwired: 1 in, 1 out]
                                n55 = property on="Index 2" class="DigNum (strict)"() -> ("Value"=w164:i32)  [unwired: 2 in, 2 out]
                                n56 = case shown="4" w164 {
                                tunnel: [w176 w177 w178 w179 w180] -> w163
                                frame 0, Default {
                                n57 = property on="Ids array" class="Arr (strict)"() -> ("Value"=w176:dbl[])  [unwired: 2 in, 2 out]
                                }
                                frame 1 {
                                n58 = property on="Ids 2" class="Arr (strict)"() -> ("Value"=w177:dbl[])  [unwired: 2 in, 2 out]
                                }
                                frame 2 {
                                n59 = property on="Ids 3" class="Arr (strict)"() -> ("Value"=w178:dbl[])  [unwired: 2 in, 2 out]
                                }
                                frame 3 {
                                n60 = property on="Ids 4" class="Arr (strict)"() -> ("Value"=w179:dbl[])  [unwired: 2 in, 2 out]
                                }
                                frame 4 {
                                n61 = property on="Ids 5" class="Arr (strict)"() -> ("Value"=w180:dbl[])  [unwired: 2 in, 2 out]
                                }
                                }
                                n62 = Insert Into Array(array=w163, index=w166, new element=w168) -> (w167:dbl[])
                                "Index" <- w166
                              }
                            }
                          }
                          frame True {
                            n63 = property on="Ids array" class="Arr (strict)"() -> ("Value"=w204:dbl[])  [unwired: 2 in, 2 out]
                            n64 = Insert Into Array(array=w204, index=w203, new element=0.0 ("new element/subarray")) -> (w201:dbl[])
                          }
                        }
                        n65 = property on="Index 2" class="DigNum (strict)"() -> ("Value"=w112:i32)  [unwired: 2 in, 2 out]
                        n66 = case shown="4" w112 {
                          tunnel: w110 -> [w116 w117 w118 w119 w120]
                          frame 0, Default {
                            n67 = property on="Ids array" class="Arr (strict)"("Value"=w116) -> ()  [unwired: 2 in, 2 out]
                          }
                          frame 1 {
                            "Ids 2" <- w117
                          }
                          frame 2 {
                            "Ids 3" <- w118
                          }
                          frame 3 {
                            "Ids 4" <- w119
                          }
                          frame 4 {
                            "Ids 5" <- w120
                          }
                        }
                        "Temp Vg" <- w111
                      }
                      "Index 2" <- w107
                    }
                  }
                  frame #3 {
                    n68 = for {
                      N: 5 -> [_]
                      i -> [w221]
                      n69 = property on="Vg array" class="Arr (strict)"() -> ("Value"=w207:dbl[])  [unwired: 2 in, 2 out]
                      n70 = property on="Vt [V]" class="DigNum (strict)"() -> ("Value"=w222:dbl)  [unwired: 2 in, 2 out]
                      n71 = Sort 1D Array(array=w207) -> (sorted array=w206:dbl[])
                      n72 = Increment(x=w221) -> (x+1=w211:i32)
                      n73 = Index Array(array=w206, index=w221) -> (element=w208:dbl)
                      n74 = Subtract(x=w208, y=w222) -> (x-y=w213:dbl)
                      n75 = Insert Into Array(array="Vds linear", index=w211, new element=w213) -> (w219:dbl[])
                      n76 = property on="u [cm^2/Vs]" class="DigNum (strict)"() -> ("Value"=w218:dbl)  [unwired: 2 in, 2 out]
                      n77 = property on="Capactiance [nf]" class="DigNum (strict)"() -> ("Value"=w217:dbl)  [unwired: 2 in, 2 out]
                      n78 = property on="Width [um]" class="DigNum (strict)"() -> ("Value"=w216:dbl)  [unwired: 2 in, 2 out]
                      n79 = property on="Length [um]" class="DigNum (strict)"() -> ("Value"=w215:dbl)  [unwired: 2 in, 2 out]
                      n80 = property on="Vt [V]" class="DigNum (strict)"() -> ("Value"=w214:dbl)  [unwired: 2 in, 2 out]
                      n81 = property on="Vds linear" class="Arr (strict)"("Value"=w219) -> ()  [unwired: 2 in, 2 out]
                      n82 = xnode "Formula"("u"=w218, "Cox"=w217, "W"=w216, "L"=w215, "Vg"=w208, "Vt"=w214) -> ("Result"=w212:dbl)  [unwired: 1 in, 1 out]
                      n83 = Insert Into Array(array="Ids Linear", index=w211, new element=w212) -> (w209:dbl[])
                      n84 = property on="Ids Linear" class="Arr (strict)"("Value"=w209) -> ()  [unwired: 2 in, 2 out]
                    }
                  }
                  frame #4 {
                    n85 = property on="Vds array" class="Arr (strict)"() -> ("Value"=w252:dbl[])  [unwired: 2 in, 2 out]
                    n86 = property on="Ids 2" class="Arr (strict)"() -> ("Value"=w251:dbl[])  [unwired: 2 in, 2 out]
                    n87 = property on="Vds array" class="Arr (strict)"() -> ("Value"=w250:dbl[])  [unwired: 2 in, 2 out]
                    n88 = property on="Ids 3" class="Arr (strict)"() -> ("Value"=w249:dbl[])  [unwired: 2 in, 2 out]
                    n89 = property on="Vds array" class="Arr (strict)"() -> ("Value"=w248:dbl[])  [unwired: 2 in, 2 out]
                    n90 = property on="Ids 4" class="Arr (strict)"() -> ("Value"=w247:dbl[])  [unwired: 2 in, 2 out]
                    n91 = property on="Vds array" class="Arr (strict)"() -> ("Value"=w246:dbl[])  [unwired: 2 in, 2 out]
                    n92 = property on="Ids 5" class="Arr (strict)"() -> ("Value"=w245:dbl[])  [unwired: 2 in, 2 out]
                    n93 = property on="Vds linear" class="Arr (strict)"() -> ("Value"=w244:dbl[])  [unwired: 2 in, 2 out]
                    n94 = property on="Ids Linear" class="Arr (strict)"() -> ("Value"=w243:dbl[])  [unwired: 2 in, 2 out]
                    n95 = Bundle("Value"=w244, "Value"=w243) -> (w242:cluster{"Value":dbl[], "Value":dbl[]})  [unwired: 1 in]
                    n96 = Bundle("Value"=w246, "Value"=w245) -> (w253:cluster{"Value":dbl[], "Value":dbl[]})  [unwired: 1 in]
                    n97 = Bundle("Value"=w248, "Value"=w247) -> (w254:cluster{"Value":dbl[], "Value":dbl[]})  [unwired: 1 in]
                    n98 = Bundle("Vds array"="Vds array", "Ids array"="Ids array") -> (w257:cluster{"Vds array":dbl[], "Ids array":dbl[]})  [unwired: 1 in]
                    n99 = Bundle("Value"=w250, "Value"=w249) -> (w255:cluster{"Value":dbl[], "Value":dbl[]})  [unwired: 1 in]
                    n100 = Bundle("Value"=w252, "Value"=w251) -> (w256:cluster{"Value":dbl[], "Value":dbl[]})  [unwired: 1 in]
                    n101 = Build Array(w257, w256, w255, w254, w253, w242) -> (→"Output Graph":cluster{"Value":dbl[], "Value":dbl[]}[])
                  }
                }
              }
            }
            n102 = case shown="True" "Clear Graph" {
              frame False {
              }
              frame True {
                w62 = 0 ("dimension size")
                n103 = Initialize Array(w62, w62) -> (w61:i32[])
                n104 = property on="Ids 2" class="Arr (strict)"("Value"=w61) -> ()  [unwired: 2 in, 2 out]
                n105 = property on="Ids array" class="Arr (strict)"("Value"=w61) -> ()  [unwired: 2 in, 2 out]
                n106 = property on="Vds array" class="Arr (strict)"("Value"=w61) -> ()  [unwired: 2 in, 2 out]
                n107 = property on="Ids 3" class="Arr (strict)"("Value"=w61) -> ()  [unwired: 2 in, 2 out]
                n108 = property on="Ids Linear" class="Arr (strict)"("Value"=w61) -> ()  [unwired: 2 in, 2 out]
                n109 = property on="Ids 4" class="Arr (strict)"("Value"=w61) -> ()  [unwired: 2 in, 2 out]
                n110 = property on="Ids 5" class="Arr (strict)"("Value"=w61) -> ()  [unwired: 2 in, 2 out]
                n111 = property on="Vds array" class="Arr (strict)"() -> ("Value"=w75:dbl[])  [unwired: 2 in, 2 out]
                n112 = property on="Ids array" class="Arr (strict)"() -> ("Value"=w74:dbl[])  [unwired: 2 in, 2 out]
                n113 = property on="Vds array" class="Arr (strict)"() -> ("Value"=w73:dbl[])  [unwired: 2 in, 2 out]
                n114 = property on="Ids 2" class="Arr (strict)"() -> ("Value"=w72:dbl[])  [unwired: 2 in, 2 out]
                n115 = property on="Vds array" class="Arr (strict)"() -> ("Value"=w71:dbl[])  [unwired: 2 in, 2 out]
                n116 = property on="Ids 3" class="Arr (strict)"() -> ("Value"=w70:dbl[])  [unwired: 2 in, 2 out]
                n117 = property on="Vds array" class="Arr (strict)"() -> ("Value"=w69:dbl[])  [unwired: 2 in, 2 out]
                n118 = property on="Ids 4" class="Arr (strict)"() -> ("Value"=w68:dbl[])  [unwired: 2 in, 2 out]
                n119 = property on="Vds array" class="Arr (strict)"() -> ("Value"=w67:dbl[])  [unwired: 2 in, 2 out]
                n120 = property on="Ids 5" class="Arr (strict)"() -> ("Value"=w66:dbl[])  [unwired: 2 in, 2 out]
                n121 = property on="Vds linear" class="Arr (strict)"() -> ("Value"=w65:dbl[])  [unwired: 2 in, 2 out]
                n122 = property on="Ids Linear" class="Arr (strict)"() -> ("Value"=w64:dbl[])  [unwired: 2 in, 2 out]
                n123 = Bundle("Value"=w65, "Value"=w64) -> (w76:cluster{"Value":dbl[], "Value":dbl[]})  [unwired: 1 in]
                n124 = Bundle("Value"=w67, "Value"=w66) -> (w77:cluster{"Value":dbl[], "Value":dbl[]})  [unwired: 1 in]
                n125 = Bundle("Value"=w69, "Value"=w68) -> (w78:cluster{"Value":dbl[], "Value":dbl[]})  [unwired: 1 in]
                n126 = Bundle("Value"=w75, "Value"=w74) -> (w81:cluster{"Value":dbl[], "Value":dbl[]})  [unwired: 1 in]
                n127 = Bundle("Value"=w71, "Value"=w70) -> (w79:cluster{"Value":dbl[], "Value":dbl[]})  [unwired: 1 in]
                n128 = Bundle("Value"=w73, "Value"=w72) -> (w80:cluster{"Value":dbl[], "Value":dbl[]})  [unwired: 1 in]
                n129 = Build Array(w81, w80, w79, w78, w77, w76) -> (w63:cluster{"Value":dbl[], "Value":dbl[]}[])
                n130 = local write "Output Graph"(w63) -> ()
              }
            }
            n131 = case shown="True" "Output Save Button" {
              frame False {
              }
              frame True {
                w10 = ","
                w31 = ","
                w47 = "\r"
                n132 = local read "Vg 3 [A]"() -> (w17:dbl)
                n133 = local read "Capactiance [nf]"() -> (w25:dbl)
                n134 = local read "Vg 5 [A]"() -> (w15:dbl)
                n135 = local read "Vg 1 [V]"() -> (w20:dbl)
                n136 = local read "Vg 2 [A]"() -> (w18:dbl)
                n137 = local read "Vg 4 [A]"() -> (w16:dbl)
                n138 = local read "Length [um]"() -> (w53:dbl)
                n139 = local read "Length [um]"() -> (w51:dbl)
                n140 = Get Date/Time String() -> (date string=w56:string, time string=w55:string)  [unwired: 3 in]
                n141 = Number To Fractional String(number=w53) -> (F-format string=w52:string)  [unwired: 3 in]
                n142 = Number To Fractional String(number=w51) -> (F-format string=w49:string)  [unwired: 3 in]
                n143 = Number To Fractional String(number=w25) -> (F-format string=w24:string)  [unwired: 3 in]
                n144 = Number To Fractional String(number=w20) -> (F-format string=w19:string)  [unwired: 3 in]
                n145 = Number To Fractional String(number=w18) -> (F-format string=w7:string)  [unwired: 3 in]
                n146 = Number To Fractional String(number=w17) -> (F-format string=w13:string)  [unwired: 3 in]
                n147 = Number To Fractional String(number=w16) -> (F-format string=w11:string)  [unwired: 3 in]
                n148 = Number To Fractional String(number=w15) -> (F-format string=w8:string)  [unwired: 3 in]
                n149 = Concatenate Strings("VD" ("string"), w31, "ID1" ("string"), w31, "ID2" ("string"), w31, "ID3" ("string"), w31, "ID4" ("string"), w31, "ID5" ("string")) -> (w45:string)
                n150 = Concatenate Strings(w56, w10, w55, w47, "Length: " ("string"), w52, w10, "Width:" ("string"), w49, w10, "Cox: " ("string"), w24, w47, "VG 1: " ("string"), w19, w10, "VG 2: " ("string"), w7, w10, "VG 3: " ("string"), w13, w10, "VG 4: " ("string"), w11, w10, "VG 5: " ("string"), w8) -> (w46:string)
                n151 = Concatenate Strings(w46, "\r", w45) -> (w35:string)
                n152 = local read "Vds array"() -> (w41:dbl[])
                n153 = local read "Ids array"() -> (w40:dbl[])
                n154 = Build Array(w35) -> (w34:string[])
                n155 = property on="Ids 2" class="Arr (strict)"() -> ("Value"=w39:dbl[])  [unwired: 2 in, 2 out]
                n156 = property on="Ids 3" class="Arr (strict)"() -> ("Value"=w38:dbl[])  [unwired: 2 in, 2 out]
                n157 = property on="Ids 4" class="Arr (strict)"() -> ("Value"=w37:dbl[])  [unwired: 2 in, 2 out]
                n158 = property on="Ids 5" class="Arr (strict)"() -> ("Value"=w36:dbl[])  [unwired: 2 in, 2 out]
                n159 = Build Array(w41, w40, w39, w38, w37, w36) -> (w28:dbl[][])
                n160 = call-poly <vilib>:"Write Delimited Spreadsheet.vi"("format (%s)"="%s", "1D data"=w34, "append to file? (new file:F)"=TRUE, "delimiter (\\t)"="," ("delimiter (\\t)")) -> ("new file path (Not A Path if cancelled)"=w27:path)  [unwired: 10 in, 1 out]
                n161 = call-poly <vilib>:"Write Delimited Spreadsheet.vi"("file path (dialog if empty)"=w27, "format (%.3f)"="%e", "2D data"=w28, "append to file? (new file:F)"=TRUE, "transpose? (no:F)"=TRUE, "delimiter (\\t)"="," ("delimiter (\\t)")) -> ()  [unwired: 8 in, 2 out]
              }
            }
          }
          frame #1 {
            n162 = case shown="True" "Transfer Start" {
              frame False {
              }
              frame True {
                n163 = stacked-sequence {
                  frame #0 {
                    n164 = Build Array("Vd 1 [V]", "Vd 2 [V]", "Vd 3 [V]", "Vd 4 [V]", "Vd 5 [V]") -> (→"Vd array":dbl[])
                  }
                  frame #1 {
                    n165 = property on="STEP" class="DigNum (strict)"() -> ("Value"=w353:dbl)  [unwired: 2 in, 2 out]
                    n166 = Divide(x="Vgs [V]", y=w353) -> (x/y=w355:dbl)
                    n167 = Absolute Value(x=w355) -> (abs(x)=w354:dbl)
                    "Vgs index" <- w354
                    n168 = for {
                      N: w354 -> [_]
                      i -> [w360]
                      n169 = property on="STEP" class="DigNum (strict)"() -> ("Value"=w357:dbl)  [unwired: 2 in, 2 out]
                      n170 = property on="Vgs array" class="Arr (strict)"() -> ("Value"=w361:dbl[])  [unwired: 2 in, 2 out]
                      n171 = Multiply(x=w360, y=w357) -> (x*y=w359:dbl)
                      n172 = Insert Into Array(array=w361, index=w360, new element=w359) -> (w358:dbl[])
                      n173 = property on="Vgs array" class="Arr (strict)"("Value"=w358) -> ()  [unwired: 2 in, 2 out]
                    }
                  }
                  frame #2 {
                    n174 = for {
                      N: 5 -> [_]
                      i -> [w363]
                      n175 = property on="Vd array" class="Arr (strict)"() -> ("Value"=w365:dbl[])  [unwired: 2 in, 2 out]
                      n176 = Index Array(array=w365, index=w363) -> (element=→"Temp Vd":dbl)
                      n177 = property on="Vgs index" class="DigNum (strict)"() -> ("Value"=w366:dbl)  [unwired: 2 in, 2 out]
                      n178 = for {
                        N: w366 -> [_]
                        i -> [w369]
                        n179 = property on="Vgs array" class="Arr (strict)"() -> ("Value"=w370:dbl[])  [unwired: 2 in, 2 out]
                        n180 = property on="Vt [V]" class="DigNum (strict)"() -> ("Value"=w367:dbl)  [unwired: 2 in, 2 out]
                        n181 = Index Array(array=w370, index=w369) -> (element=w368:dbl)
                        n182 = Less Or Equal?(x=w368, y=w367) -> (x <= y?=w373:bool)
                        n183 = case shown="False" w373 {
                          tunnel: w369 -> [w384 w462]
                          tunnel: [w382 w460] -> w371
                          frame False {
                            n184 = property on="Vt [V]" class="DigNum (strict)"() -> ("Value"=w379:dbl)  [unwired: 2 in, 2 out]
                            n185 = property on="Vgs array" class="Arr (strict)"() -> ("Value"=w385:dbl[])  [unwired: 2 in, 2 out]
                            n186 = Index Array(array=w385, index=w384) -> (element=w381:dbl)
                            n187 = Subtract(x=w381, y=w379) -> (x-y=w383:dbl)
                            n188 = property on="Temp Vd" class="DigNum (strict)"() -> ("Value"=w380:dbl)  [unwired: 2 in, 2 out]
                            n189 = Less Or Equal?(x=w380, y=w383) -> (x <= y?=w386:bool)
                            n190 = case shown="True" w386 {
                              tunnel: w384 -> [w393 w431]
                              tunnel: [w398 w432] -> w382
                              frame False {
                                n191 = property on="Vt [V]" class="DigNum (strict)"() -> ("Value"=w391:dbl)  [unwired: 2 in, 2 out]
                                n192 = property on="Length [um]" class="DigNum (strict)"() -> ("Value"=w387:dbl)  [unwired: 2 in, 2 out]
                                n193 = property on="Vgs array" class="Arr (strict)"() -> ("Value"=w394:dbl[])  [unwired: 2 in, 2 out]
                                n194 = property on="Capactiance [nf]" class="DigNum (strict)"() -> ("Value"=w389:dbl)  [unwired: 2 in, 2 out]
                                n195 = property on="u [cm^2/Vs]" class="DigNum (strict)"() -> ("Value"=w390:dbl)  [unwired: 2 in, 2 out]
                                n196 = property on="Width [um]" class="DigNum (strict)"() -> ("Value"=w388:dbl)  [unwired: 2 in, 2 out]
                                n197 = Index Array(array=w394, index=w393) -> (element=w392:dbl)
                                n198 = xnode "Formula"("u"=w390, "Cox"=w389, "W"=w388, "L"=w387, "Vg"=w392, "Vt"=w391) -> ("Result"=w395:dbl)  [unwired: 1 in, 1 out]
                                n199 = property on="Index 3" class="DigNum (strict)"() -> ("Value"=w397:i32)  [unwired: 2 in, 2 out]
                                n200 = case shown="4" w397 {
                                tunnel: [w399 w400 w401 w402 w403] -> w396
                                frame 0, Default {
                                n201 = property on="Ids array 2" class="Arr (strict)"() -> ("Value"=w399:dbl[])  [unwired: 2 in, 2 out]
                                }
                                frame 1 {
                                n202 = property on="Ids 6" class="Arr (strict)"() -> ("Value"=w400:dbl[])  [unwired: 2 in, 2 out]
                                }
                                frame 2 {
                                n203 = property on="Ids 7" class="Arr (strict)"() -> ("Value"=w401:dbl[])  [unwired: 2 in, 2 out]
                                }
                                frame 3 {
                                n204 = property on="Ids 8" class="Arr (strict)"() -> ("Value"=w402:dbl[])  [unwired: 2 in, 2 out]
                                }
                                frame 4 {
                                n205 = property on="Ids 9" class="Arr (strict)"() -> ("Value"=w403:dbl[])  [unwired: 2 in, 2 out]
                                }
                                }
                                n206 = Insert Into Array(array=w396, index=w393, new element=w395) -> (w398:dbl[])
                              }
                              frame True {
                                n207 = property on="Temp Vd" class="DigNum (strict)"() -> ("Value"=w427:dbl)  [unwired: 2 in, 2 out]
                                n208 = property on="Length [um]" class="DigNum (strict)"() -> ("Value"=w422:dbl)  [unwired: 2 in, 2 out]
                                n209 = property on="Capactiance [nf]" class="DigNum (strict)"() -> ("Value"=w424:dbl)  [unwired: 2 in, 2 out]
                                n210 = property on="Vgs array" class="Arr (strict)"() -> ("Value"=w434:dbl[])  [unwired: 2 in, 2 out]
                                n211 = property on="u [cm^2/Vs]" class="DigNum (strict)"() -> ("Value"=w425:dbl)  [unwired: 2 in, 2 out]
                                n212 = property on="Width [um]" class="DigNum (strict)"() -> ("Value"=w423:dbl)  [unwired: 2 in, 2 out]
                                n213 = Index Array(array=w434, index=w431) -> (element=w428:dbl)
                                n214 = property on="Vt [V]" class="DigNum (strict)"() -> ("Value"=w426:dbl)  [unwired: 2 in, 2 out]
                                n215 = xnode "Formula"("W"=w423, "L"=w422, "Cox"=w424, "u"=w425, "Vg"=w428, "Vd"=w427, "Vt"=w426) -> ("Result"=w433:dbl)  [unwired: 1 in, 1 out]
                                n216 = property on="Index 3" class="DigNum (strict)"() -> ("Value"=w430:i32)  [unwired: 2 in, 2 out]
                                n217 = case shown="4" w430 {
                                tunnel: [w435 w436 w437 w438 w439] -> w429
                                frame 0, Default {
                                n218 = property on="Ids array 2" class="Arr (strict)"() -> ("Value"=w435:dbl[])  [unwired: 2 in, 2 out]
                                }
                                frame 1 {
                                n219 = property on="Ids 6" class="Arr (strict)"() -> ("Value"=w436:dbl[])  [unwired: 2 in, 2 out]
                                }
                                frame 2 {
                                n220 = property on="Ids 7" class="Arr (strict)"() -> ("Value"=w437:dbl[])  [unwired: 2 in, 2 out]
                                }
                                frame 3 {
                                n221 = property on="Ids 8" class="Arr (strict)"() -> ("Value"=w438:dbl[])  [unwired: 2 in, 2 out]
                                }
                                frame 4 {
                                n222 = property on="Ids 9" class="Arr (strict)"() -> ("Value"=w439:dbl[])  [unwired: 2 in, 2 out]
                                }
                                }
                                n223 = Insert Into Array(array=w429, index=w431, new element=w433) -> (w432:dbl[])
                              }
                            }
                          }
                          frame True {
                            n224 = property on="Ids array 2" class="Arr (strict)"() -> ("Value"=w463:dbl[])  [unwired: 2 in, 2 out]
                            n225 = Insert Into Array(array=w463, index=w462, new element=0.0 ("new element/subarray")) -> (w460:dbl[])
                          }
                        }
                        n226 = property on="Index 3" class="DigNum (strict)"() -> ("Value"=w372:i32)  [unwired: 2 in, 2 out]
                        n227 = case shown="0, Default" w372 {
                          tunnel: w371 -> [w374 w375 w376 w377 w378]
                          frame 0, Default {
                            n228 = property on="Ids array 2" class="Arr (strict)"("Value"=w374) -> ()  [unwired: 2 in, 2 out]
                          }
                          frame 1 {
                            "Ids 6" <- w375
                          }
                          frame 2 {
                            "Ids 7" <- w376
                          }
                          frame 3 {
                            "Ids 8" <- w377
                          }
                          frame 4 {
                            "Ids 9" <- w378
                          }
                        }
                      }
                      "Index 3" <- w363
                    }
                  }
                  frame #3 {
                    n229 = property on="Vgs array" class="Arr (strict)"() -> ("Value"=w471:dbl[])  [unwired: 2 in, 2 out]
                    n230 = property on="Ids 6" class="Arr (strict)"() -> ("Value"=w470:dbl[])  [unwired: 2 in, 2 out]
                    n231 = property on="Vgs array" class="Arr (strict)"() -> ("Value"=w469:dbl[])  [unwired: 2 in, 2 out]
                    n232 = property on="Ids 7" class="Arr (strict)"() -> ("Value"=w468:dbl[])  [unwired: 2 in, 2 out]
                    n233 = property on="Vgs array" class="Arr (strict)"() -> ("Value"=w467:dbl[])  [unwired: 2 in, 2 out]
                    n234 = property on="Ids 8" class="Arr (strict)"() -> ("Value"=w466:dbl[])  [unwired: 2 in, 2 out]
                    n235 = property on="Vgs array" class="Arr (strict)"() -> ("Value"=w465:dbl[])  [unwired: 2 in, 2 out]
                    n236 = property on="Ids 9" class="Arr (strict)"() -> ("Value"=w464:dbl[])  [unwired: 2 in, 2 out]
                    n237 = Bundle("Value"=w465, "Value"=w464) -> (w473:cluster{"Value":dbl[], "Value":dbl[]})  [unwired: 1 in]
                    n238 = Bundle("Value"=w467, "Value"=w466) -> (w474:cluster{"Value":dbl[], "Value":dbl[]})  [unwired: 1 in]
                    n239 = Bundle("Vgs array"="Vgs array", "Ids array 2"="Ids array 2") -> (w477:cluster{"Vgs array":dbl[], "Ids array 2":dbl[]})  [unwired: 1 in]
                    n240 = Bundle("Value"=w469, "Value"=w468) -> (w475:cluster{"Value":dbl[], "Value":dbl[]})  [unwired: 1 in]
                    n241 = Bundle("Value"=w471, "Value"=w470) -> (w476:cluster{"Value":dbl[], "Value":dbl[]})  [unwired: 1 in]
                    n242 = Build Array(w477, w476, w475, w474, w473) -> (→"Transfer Graph":cluster{"Value":dbl[], "Value":dbl[]}[])
                  }
                }
              }
            }
            n243 = case shown="True" "Graph Clear." {
              frame False {
              }
              frame True {
                w330 = 0 ("dimension size")
                n244 = Initialize Array(w330, w330) -> (w329:i32[])
                n245 = property on="Ids 6" class="Arr (strict)"("Value"=w329) -> ()  [unwired: 2 in, 2 out]
                n246 = property on="Ids 7" class="Arr (strict)"("Value"=w329) -> ()  [unwired: 2 in, 2 out]
                n247 = property on="Vgs array" class="Arr (strict)"("Value"=w329) -> ()  [unwired: 2 in, 2 out]
                n248 = property on="Ids array 2" class="Arr (strict)"("Value"=w329) -> ()  [unwired: 2 in, 2 out]
                n249 = property on="Ids 8" class="Arr (strict)"("Value"=w329) -> ()  [unwired: 2 in, 2 out]
                n250 = property on="Ids 9" class="Arr (strict)"("Value"=w329) -> ()  [unwired: 2 in, 2 out]
                n251 = property on="Ids 9" class="Arr (strict)"() -> ("Value"=w332:dbl[])  [unwired: 2 in, 2 out]
                n252 = property on="Vgs array" class="Arr (strict)"() -> ("Value"=w341:dbl[])  [unwired: 2 in, 2 out]
                n253 = property on="Ids array 2" class="Arr (strict)"() -> ("Value"=w340:dbl[])  [unwired: 2 in, 2 out]
                n254 = property on="Vgs array" class="Arr (strict)"() -> ("Value"=w339:dbl[])  [unwired: 2 in, 2 out]
                n255 = property on="Ids 6" class="Arr (strict)"() -> ("Value"=w338:dbl[])  [unwired: 2 in, 2 out]
                n256 = property on="Vgs array" class="Arr (strict)"() -> ("Value"=w337:dbl[])  [unwired: 2 in, 2 out]
                n257 = property on="Ids 7" class="Arr (strict)"() -> ("Value"=w336:dbl[])  [unwired: 2 in, 2 out]
                n258 = property on="Vgs array" class="Arr (strict)"() -> ("Value"=w335:dbl[])  [unwired: 2 in, 2 out]
                n259 = property on="Ids 8" class="Arr (strict)"() -> ("Value"=w334:dbl[])  [unwired: 2 in, 2 out]
                n260 = property on="Vgs array" class="Arr (strict)"() -> ("Value"=w333:dbl[])  [unwired: 2 in, 2 out]
                n261 = Bundle("Value"=w333, "Value"=w332) -> (w342:cluster{"Value":dbl[], "Value":dbl[]})  [unwired: 1 in]
                n262 = Bundle("Value"=w335, "Value"=w334) -> (w343:cluster{"Value":dbl[], "Value":dbl[]})  [unwired: 1 in]
                n263 = Bundle("Value"=w341, "Value"=w340) -> (w346:cluster{"Value":dbl[], "Value":dbl[]})  [unwired: 1 in]
                n264 = Bundle("Value"=w337, "Value"=w336) -> (w344:cluster{"Value":dbl[], "Value":dbl[]})  [unwired: 1 in]
                n265 = Bundle("Value"=w339, "Value"=w338) -> (w345:cluster{"Value":dbl[], "Value":dbl[]})  [unwired: 1 in]
                n266 = Build Array(w346, w345, w344, w343, w342) -> (w331:cluster{"Value":dbl[], "Value":dbl[]}[])
                n267 = local write "Transfer Graph"(w331) -> ()
              }
            }
            n268 = case shown="True" "Transfer Save Button" {
              frame False {
              }
              frame True {
                w283 = ","
                w289 = "\r"
                w292 = ","
                n269 = local read "u [cm^2/Vs]"() -> (w299:dbl)
                n270 = local read "Vd 1 [V]"() -> (w317:dbl)
                n271 = local read "Vd 2 [V]"() -> (w314:dbl)
                n272 = local read "Vd 3 [V]"() -> (w313:dbl)
                n273 = local read "Vd 4 [V]"() -> (w312:dbl)
                n274 = local read "Vd 5 [V]"() -> (w311:dbl)
                n275 = local read "Capactiance [nf]"() -> (w320:dbl)
                n276 = Get Date/Time String() -> (date string=w328:string, time string=w327:string)  [unwired: 3 in]
                n277 = local read "Length [um]"() -> (w325:dbl)
                n278 = local read "Width [um]"() -> (w323:dbl)
                n279 = local read "Vt [V]"() -> (w301:dbl)
                n280 = local read "STEP"() -> (w300:dbl)
                n281 = local read "Vgs [V]"() -> (w302:dbl)
                n282 = Number To Fractional String(number=w302) -> (F-format string=w297:string)  [unwired: 3 in]
                n283 = Number To Fractional String(number=w311) -> (F-format string=w303:string)  [unwired: 3 in]
                n284 = Number To Fractional String(number=w301) -> (F-format string=w295:string)  [unwired: 3 in]
                n285 = Number To Fractional String(number=w300) -> (F-format string=w293:string)  [unwired: 3 in]
                n286 = Number To Fractional String(number=w299) -> (F-format string=w290:string)  [unwired: 3 in]
                n287 = Number To Fractional String(number=w312) -> (F-format string=w305:string)  [unwired: 3 in]
                n288 = Number To Fractional String(number=w313) -> (F-format string=w307:string)  [unwired: 3 in]
                n289 = Number To Fractional String(number=w317) -> (F-format string=w315:string)  [unwired: 3 in]
                n290 = Number To Fractional String(number=w314) -> (F-format string=w309:string)  [unwired: 3 in]
                n291 = Number To Fractional String(number=w325) -> (F-format string=w324:string)  [unwired: 3 in]
                n292 = Number To Fractional String(number=w323) -> (F-format string=w321:string)  [unwired: 3 in]
                n293 = Number To Fractional String(number=w320) -> (F-format string=w318:string)  [unwired: 3 in]
                n294 = Concatenate Strings(w328, w292, w327, w289, "Length: ", w324, w292, "Width: ", w321, w292, "Capacitance: ", w318, w289, "Vd 1: ", w315, w292, "Vd 2: ", w309, w292, "Vd 3: ", w307, w292, "Vd 4: ", w305, w292, "Vd 5: ", w303, w289, "Vgs: ", w297, w292, "Vt: ", w295, w292, "Step:", w293, w292, "Mobility: ", w290, w289) -> (w280:string)
                n295 = Concatenate Strings("VG", w283, "ID 1", w283, "ID 2", w283, "ID 3", w283, "ID 4", w283, "ID 5", "\r") -> (w279:string)
                n296 = Concatenate Strings(w280, w279) -> (w278:string)
                n297 = property on="Ids array 2" class="Arr (strict)"() -> ("Value"=w273:dbl[])  [unwired: 2 in, 2 out]
                n298 = property on="Vgs array" class="Arr (strict)"() -> ("Value"=w274:dbl[])  [unwired: 2 in, 2 out]
                n299 = property on="Ids 6" class="Arr (strict)"() -> ("Value"=w272:dbl[])  [unwired: 2 in, 2 out]
                n300 = property on="Ids 7" class="Arr (strict)"() -> ("Value"=w271:dbl[])  [unwired: 2 in, 2 out]
                n301 = property on="Ids 8" class="Arr (strict)"() -> ("Value"=w270:dbl[])  [unwired: 2 in, 2 out]
                n302 = property on="Ids 9" class="Arr (strict)"() -> ("Value"=w269:dbl[])  [unwired: 2 in, 2 out]
                n303 = Build Array(w278) -> (w277:string[])
                n304 = call-poly <vilib>:"Write Delimited Spreadsheet.vi"("format (%s)"="%s", "1D data"=w277, "delimiter (\\t)"="," ("delimiter (\\t)")) -> ("new file path (Not A Path if cancelled)"=w264:path)  [unwired: 11 in, 1 out]
                n305 = Build Array(w274, w273, w272, w271, w270, w269) -> (w268:dbl[][])
                n306 = call-poly <vilib>:"Write Delimited Spreadsheet.vi"("file path (dialog if empty)"=w264, "format (%.3f)"="%e", "2D data"=w268, "append to file? (new file:F)"=TRUE, "transpose? (no:F)"=TRUE, "delimiter (\\t)"="," ("delimiter (\\t)")) -> ()  [unwired: 8 in, 2 out]
              }
            }
          }
        }
      }
    }
    frame "Transfer" {
      # "You only can edit certain parts of the State Machine.  Right-click the While Loop and select \nUnlock Code From State Diagram to unlock the state machine from the State Diagram Editor."
      # "Right-click the border of this outer While Loop and select Edit State Diagram to open the State Diagram Editor Window."
      n307 = while {
        shift-right: [w483] -> _
        shift-left: T1."Init" -> [w484]
        stop <- w482 stop-if-true
        # "This outer Case structure contains cases that correspond to the states in the state diagram.  \nConfigure each case to reflect the actions you want each state to perform."
        n308 = case shown="\"Measuring\"" w484 {
          tunnel: [T1."_Quit_" w498 w528 w604 w796 w899 w928] -> w483
          frame "_Quit_" {
            # "The _Quit_ case has no corresponding state on the state diagram -\nit exists to indicate to the outer While Loop when to stop executing.\nThis case is executed immediately after the case for any terminal state, \nand is the last case to execute.  Place any general clean-up code here."
          }
          frame "Init" {
            w493 = 0
            w496 = 2
            w486 = 0
            # "Each non-terminal state has at least one transition.\nThis inner While Loop and inner Case structure \ndetermine which state executes next.  The While \nLoop executes the cases in the Case structure until \nthe conditional terminal receives a TRUE value."
            n309 = property on="Run Button" class="Bool"("DisabledEnum"=w486) -> (error out=w497:errorcluster)  [unwired: 2 in, 1 out]
            n310 = while {
              tunnel: [w500] -> w498
              i -> [w503]
              stop <- w499 stop-if-true
              n311 = external ("Integer to Enum")(enum16{"default"}."default", w503) -> (w501:enum16{"default"})
              n312 = case shown="\"default\"" w501 {
                tunnel: [T1."Waiting"] -> w500
                tunnel: [TRUE] -> w499
                frame "default" {
                }
              }
            }
            n313 = Initialize Array(w493, w493) -> (w491:i32[])
            n314 = property on="Cancel Button" class="Bool"(error in=w497, "DisabledEnum"=w486) -> (error out=w488:errorcluster)  [unwired: 1 in, 1 out]
            n315 = call "Convert to Dynamic Data11"("Array"=w491) -> ("Dynamic Data Type"=w490:dynamicdata)  [unwired: 3 in]
            n316 = call "Convert to Dynamic Data10"("Array"=w491) -> ("Dynamic Data Type"=w492:dynamicdata)  [unwired: 3 in]
            n317 = call "IS2"("Y Input"=w490, "X Input"=w492) -> ("XY Graph"=w489:cluster{"Y":dbl[], "Y":dbl[]}[])  [unwired: 3 in, 6 out]
            n318 = property on="Hysteresis" class="Bool (strict)"(error in=w488, "DisabledEnum"=w486) -> (error out=w487:errorcluster)  [unwired: 1 in, 1 out]
            n319 = property on="Regime" class="Bool (strict)"(error in=w487, "DisabledEnum"=w486) -> (error out=w495:errorcluster)  [unwired: 1 in, 1 out]
            n320 = local write "ID-VG 2"(w489) -> ()
            n321 = local write "IS-VG"(w489) -> ()
            n322 = local write "ID-VG"(w489) -> ()
            n323 = local write "Mobility-VG"(w489) -> ()
            n324 = property on="Stop Button" class="Bool"(error in=w495, "DisabledEnum"=w496) -> (error out=w494:errorcluster)  [unwired: 1 in, 1 out]
            n325 = property on="Transfer Save" class="Bool"(error in=w494, "DisabledEnum"=w496) -> ()  [unwired: 1 in, 2 out]
          }
          frame "Waiting" {
            n326 = flat-sequence {
              tunnel: [w532] -> w527
              tunnel: w527 -> [w544]
              frame #0 {
                n327 = Concatenate Strings("*RST", "\n") -> (w537:string)
                n328 = VISA Write(VISA resource name="VISA resource name", write buffer=w537) -> (VISA resource name out=w541:refnum<visa-resource-name>)  [unwired: 1 in, 2 out]
                n329 = Format Into String(format string="AIT 1,2,%d", "Int time") -> (resulting string=w531:string)  [unwired: 2 in, 1 out]
                n330 = Concatenate Strings(w531, "\n") -> (w535:string)
                n331 = Concatenate Strings("CN;FMT 12,0;AAD 1,1;AAD 2,1;AAD 3,1", "\n") -> (w542:string)
                n332 = VISA Write(VISA resource name=w541, write buffer=w542) -> (VISA resource name out=w530:refnum<visa-resource-name>)  [unwired: 1 in, 2 out]
                n333 = VISA Write(VISA resource name=w530, write buffer=w535) -> (VISA resource name out=w532:refnum<visa-resource-name>)  [unwired: 1 in, 2 out]
              }
              frame #1 {
                n334 = Format Into String(format string="DV %d,0,%f,%f; DV %d,0,%f,%f", "VS SMU No", "VS [V]", "VS Comp [V].", "VD SMU No", "VD [V]", "VD Comp [V].") -> (resulting string=w547:string)  [unwired: 2 in, 1 out]
                n335 = Concatenate Strings(w547, "\n") -> (w548:string)
                n336 = VISA Write(VISA resource name=w544, write buffer=w548) -> ()  [unwired: 1 in, 3 out]
              }
            }
            n337 = while {
              tunnel: [w556] -> w528
              i -> [w559]
              stop <- w555 stop-if-true
              n338 = external ("Integer to Enum")(enum16{"Cancel", "Start", "Saving", "default"}."Cancel", w559) -> (w557:enum16{"Cancel", "Start", "Saving", "default"})
              n339 = case shown="\"Start\"" w557 {
                tunnel: [T1."Exit" T1."Measuring" T1."Save" T1."Waiting"] -> w556
                tunnel: ["Cancel Button" "Run Button" "Transfer Save" TRUE] -> w555
                frame "Cancel" {
                  # "Add a boolean wire\nthat is TRUE when\nthis transition is active"
                }
                frame "Start" {
                  # "Add a boolean wire\nthat is TRUE when\nthis transition is active"
                }
                frame "Saving" {
                  # "Add a boolean wire\nthat is TRUE when\nthis transition is active"
                }
                frame "default" {
                }
              }
            }
          }
          frame "Measuring" {
            w589 = 2
            w597 = 0
            n340 = Initialize Array(w597, w597) -> (w603:i32[])
            n341 = while {
              shift-right: [w621] -> w602
              shift-left: w603 -> [w624]
              shift-right: [w622] -> w601
              shift-left: w603 -> [w623]
              shift-right: [w620] -> w600
              shift-left: w603 -> [w619]
              shift-right: [w617] -> w599
              shift-left: w603 -> [w618]
              shift-right: [w615] -> w598
              shift-left: w603 -> [w616]
              tunnel: [w610] -> w594
              i -> [w612]
              stop <- w610 stop-if-true
              n342 = Subtract(x="VG stop [V]", y="VG start [V]") -> (x-y=w629:dbl)
              n343 = Divide(x=w629, y="VG step [V]") -> (x/y=w626:dbl)
              n344 = Wait Until Next ms Multiple(millisecond multiple=u32 100) -> ()  [unwired: 1 out]
              n345 = case shown="True" "Hysteresis" {
                tunnel: w626 -> [w752 w756]
                tunnel: [w752 w755] -> w627
                frame False {
                  n346 = local write "Hysteresis LED"(FALSE ("Hysteresis LED")) -> ()
                }
                frame True {
                  n347 = Multiply(x=2, y=w756) -> (x*y=w755:dbl)
                  "Hysteresis LED" <- TRUE ("Hysteresis Indicator")
                }
              }
              n348 = Increment(x=w627) -> (x+1=w607:dbl)
              n349 = for {
                N: w607 -> [_]
                shift-right: [w650] -> _
                shift-left: "VG start [V]" -> [w633]
                tunnel: w626 -> [w665]
                tunnel: "VG step [V]" -> [w669]
                shift-right: [w649] -> w621
                shift-left: w624 -> [w664]
                shift-right: [w647] -> w622
                shift-left: w623 -> [w663]
                shift-right: [w644] -> w620
                shift-left: w619 -> [w655]
                shift-right: [w640] -> w617
                shift-left: w618 -> [w642]
                shift-right: [w636] -> w615
                shift-left: w616 -> [w656]
                tunnel: ["Stop Button"] -> w608
                i -> [w632]
                stop <- "Stop Button" stop-if-true
                n350 = flat-sequence {
                  tunnel: ["VG SMU No"] -> w654
                  tunnel: [w671] -> w653
                  tunnel: w633 -> [w670]
                  tunnel: w654 -> [w675]
                  tunnel: w653 -> [w678]
                  tunnel: [w677] -> w652
                  tunnel: [w676] -> w648
                  tunnel: w652 -> [w681]
                  tunnel: [w680] -> w651
                  tunnel: [w679] -> w645
                  tunnel: w651 -> [w693]
                  tunnel: w642 -> [w685]
                  tunnel: [w686] -> w641
                  tunnel: [w696] -> w637
                  frame #0 {
                    n351 = local read "VISA resource name"() -> (w673:refnum<visa-resource-name>)
                    n352 = call "setV.vi"("comp"="VG Comp [V].", "voltage"=w670, "SMU"="VG SMU No", "VISA resource name"=w673) -> ("VISA resource name dup"=w671:refnum<visa-resource-name>)
                  }
                  frame #1 {
                    n353 = call "readI.vi"("SMU"=w675, "*VISA resource name*"=w678) -> ("current"=w676:dbl, "*VISA resource name*DUP"=w677:refnum<visa-resource-name>)
                    "IG [V]" <- w676
                  }
                  frame #2 {
                    n354 = local read "VS SMU No"() -> (w682:dbl)
                    n355 = call "readI.vi"("SMU"=w682, "*VISA resource name*"=w681) -> ("current"=w679:dbl, "*VISA resource name*DUP"=w680:refnum<visa-resource-name>)
                    "IS [V]" <- w679
                  }
                  frame #3 {
                    n356 = local read "VD SMU No"() -> (w683:dbl)
                    n357 = call "readI.vi"("SMU"=w683, "*VISA resource name*"=w693) -> ("current"=w686:dbl)  [unwired: 1 out]
                    "ID [V]" <- w686
                    n358 = Array Size(array=w685) -> (size(s)=w694:i32)
                    n359 = Decrement(x=w694) -> (x-1=w695:i32)
                    n360 = Index Array(array=w685, index=w695) -> (element=w690:dbl)
                    n361 = Absolute Value(x=w686) -> (abs(x)=w689:dbl)
                    n362 = Absolute Value(x=w690) -> (abs(x)=w687:dbl)
                    n363 = Square Root(x=w687) -> (sqrt(x)=w692:dbl)
                    n364 = Square Root(x=w689) -> (sqrt(x)=w691:dbl)
                    n365 = Subtract(x=w692, y=w691) -> (x-y=w688:dbl)
                    n366 = Absolute Value(x=w688) -> (abs(x)=→"d'ID":dbl)
                  }
                  frame #4 {
                    n367 = case shown="False" "Regime" {
                      tunnel: [w698 w721] -> w696
                      frame True {
                        n368 = local read "Length [um]"() -> (w701:dbl)
                        n369 = local read "Width [um]"() -> (w700:dbl)
                        n370 = local read "Thickness [nm]"() -> (w699:dbl)
                        n371 = local read "VG step [V]"() -> (w704:dbl)
                        n372 = local read "d'ID"() -> (w703:dbl)
                        n373 = Absolute Value(x=w704) -> (abs(x)=w702:dbl)
                        n374 = xnode "Formula"("d'ID"=w703, "d'VG"=w702, "L"=w701, "W"=w700, "tox"=w699) -> ("Result"=w698:dbl)  [unwired: 1 in, 1 out]
                        n375 = local write "Mobility [cm^2/Vs]"(w698) -> ()
                      }
                      frame False {
                        n376 = local read "VG step [V]"() -> (w728:dbl)
                        n377 = local read "VD [V]"() -> (w729:dbl)
                        n378 = local read "d'ID"() -> (w727:dbl)
                        n379 = Absolute Value(x=w729) -> (abs(x)=w725:dbl)
                        n380 = Absolute Value(x=w728) -> (abs(x)=w726:dbl)
                        n381 = xnode "Formula"("d'ID"=w727, "d'VG"=w726, "VD"=w725, "L"="Length [um]", "W"="Width [um]", "ti"="Thickness [nm]") -> ("Result"=w721:dbl)  [unwired: 1 in, 1 out]
                        "Mobility [cm^2/Vs]" <- w721
                      }
                    }
                  }
                }
                n382 = Decrement(x=w665) -> (x-1=w666:dbl)
                n383 = Greater?(x=w632, y=w666) -> (0:w667:bool)
                n384 = case shown="True" w667 {
                  tunnel: w669 -> [w748 w749]
                  tunnel: [w748 w750] -> w668
                  frame False {
                  }
                  frame True {
                    n385 = Negate(x=w749) -> (-x=w750:dbl)
                  }
                }
                n386 = Add(x=w633, y=w668) -> (x+y=w650:dbl)
                n387 = Build Array (concatenate)(w664, w633) -> (w649:dbl[])
                n388 = call "Convert to Dynamic Data"("Array"=w649) -> ("Dynamic Data Type"=w634:dynamicdata)  [unwired: 3 out]
                n389 = Build Array (concatenate)(w663, w648) -> (w647:dbl[])
                n390 = Absolute Value(x=w647) -> (abs(x)=w662:dbl[])
                n391 = call "Convert to Dynamic Data4"("Array"=w662) -> ("Dynamic Data Type"=w646:dynamicdata)  [unwired: 3 out]
                n392 = call "IS"("Y Input"=w646, "X Input"=w634) -> ("XY Graph"=→"ID-VG 2":cluster{"Y":dbl[], "Y":dbl[]}[])  [unwired: 3 in, 6 out]
                n393 = Build Array (concatenate)(w655, w645) -> (w644:dbl[])
                n394 = Absolute Value(x=w644) -> (abs(x)=w661:dbl[])
                n395 = call "Convert to Dynamic Data3"("Array"=w661) -> ("Dynamic Data Type"=w643:dynamicdata)  [unwired: 3 out]
                n396 = call "IG2"("Y Input"=w643, "X Input"=w634) -> ("XY Graph"=→"IS-VG":cluster{"Y":dbl[], "Y":dbl[]}[])  [unwired: 3 in, 6 out]
                n397 = Build Array (concatenate)(w642, w641) -> (w640:dbl[])
                n398 = Absolute Value(x=w640) -> (abs(x)=w639:dbl[])
                n399 = call "Convert to Dynamic Data5"("Array"=w639) -> ("Dynamic Data Type"=w638:dynamicdata)  [unwired: 3 out]
                n400 = call "IG3"("Y Input"=w638, "X Input"=w634) -> ("XY Graph"=→"ID-VG":cluster{"Y":dbl[], "Y":dbl[]}[])  [unwired: 3 in, 6 out]
                n401 = Build Array (concatenate)(w656, w637) -> (w636:dbl[])
                n402 = Absolute Value(x=w636) -> (abs(x)=w658:dbl[])
                n403 = call "Convert to Dynamic Data2"("Array"=w658) -> ("Dynamic Data Type"=w635:dynamicdata)  [unwired: 3 out]
                n404 = call "IG"("Y Input"=w635, "X Input"=w634) -> ("XY Graph"=→"Mobility-VG":cluster{"Y":dbl[], "Y":dbl[]}[])  [unwired: 3 in, 6 out]
                "VG [V]" <- w633
              }
              n405 = Decrement(x="Repeat Times") -> (x-1=w606:i32)
              n406 = Greater Or Equal?(x=w612, y=w606) -> (x >= y?=w611:bool)
              n407 = Or(x=w611, y=w608) -> (x .or. y?=w610:bool)
            }
            "VG Array" <- w602
            "IG Array" <- w601
            "IS Array" <- w600
            "ID Array" <- w599
            "Mobility Array" <- w598
            n408 = property on="Run Button" class="Bool"("DisabledEnum"=w589) -> (error out=w596:errorcluster)  [unwired: 2 in, 1 out]
            n409 = property on="Transfer Save" class="Bool"(error in=w596, "DisabledEnum"=w589) -> (error out=w593:errorcluster)  [unwired: 1 in, 1 out]
            n410 = property on="Hysteresis" class="Bool (strict)"(error in=w593, "DisabledEnum"=w589) -> (error out=w592:errorcluster)  [unwired: 1 in, 1 out]
            n411 = property on="Regime" class="Bool (strict)"(error in=w592, "DisabledEnum"=w589) -> (error out=w591:errorcluster)  [unwired: 1 in, 1 out]
            n412 = property on="Cancel Button" class="Bool"(error in=w591, "DisabledEnum"=w589) -> (error out=w590:errorcluster)  [unwired: 1 in, 1 out]
            n413 = property on="Stop Button" class="Bool"(error in=w590, "DisabledEnum"=0) -> ()  [unwired: 1 in, 2 out]
            n414 = while {
              tunnel: [w759] -> w604
              tunnel: w594 -> [w757]
              i -> [w762]
              stop <- w758 stop-if-true
              n415 = external ("Integer to Enum")(enum16{"Stop", "default"}."Stop", w762) -> (w760:enum16{"Stop", "default"})
              n416 = case shown="\"Stop\"" w760 {
                tunnel: [T1."Stop" T1."Measuring"] -> w759
                tunnel: [w784 TRUE] -> w758
                tunnel: w757 -> [w784 _]
                frame "Stop" {
                  # "Add a boolean wire\nthat is TRUE when\nthis transition is active"
                }
                frame "default" {
                }
              }
            }
          }
          frame "Stop" {
            w791 = 0
            n417 = property on="Run Button" class="Bool"("DisabledEnum"=w791) -> (error out=w795:errorcluster)  [unwired: 2 in, 1 out]
            n418 = property on="Transfer Save" class="Bool"(error in=w795, "DisabledEnum"=w791) -> (error out=w794:errorcluster)  [unwired: 1 in, 1 out]
            n419 = property on="Cancel Button" class="Bool"(error in=w794, "DisabledEnum"=w791) -> (error out=w790:errorcluster)  [unwired: 1 in, 1 out]
            n420 = property on="Hysteresis" class="Bool (strict)"(error in=w790, "DisabledEnum"=w791) -> (error out=w789:errorcluster)  [unwired: 1 in, 1 out]
            n421 = property on="Regime" class="Bool (strict)"(error in=w789, "DisabledEnum"=w791) -> (error out=w793:errorcluster)  [unwired: 1 in, 1 out]
            n422 = while {
              tunnel: [w810] -> w796
              i -> [w813]
              stop <- w809 stop-if-true
              n423 = external ("Integer to Enum")(enum16{"default"}."default", w813) -> (w811:enum16{"default"})
              n424 = case shown="\"default\"" w811 {
                tunnel: [T1."Waiting"] -> w810
                tunnel: [TRUE] -> w809
                frame "default" {
                }
              }
            }
            n425 = property on="Stop Button" class="Bool"(error in=w793, "DisabledEnum"=2) -> ()  [unwired: 1 in, 2 out]
            n426 = flat-sequence {
              tunnel: [w798] -> w788
              tunnel: w788 -> [w806]
              frame #0 {
                w797 = 0.001
                w802 = 0
                n427 = local read "VISA resource name"() -> (w798:refnum<visa-resource-name>)
                n428 = call "setV.vi"("comp"=w797, "voltage"=w802, "SMU"=1, "VISA resource name"=w798) -> ("VISA resource name dup"=w800:refnum<visa-resource-name>)
                n429 = call "setV.vi"("comp"=w797, "voltage"=w802, "SMU"=2, "VISA resource name"=w800) -> ("VISA resource name dup"=w801:refnum<visa-resource-name>)
                n430 = call "setV.vi"("comp"=w797, "voltage"=w802, "SMU"=3, "VISA resource name"=w801) -> ()  [unwired: 1 out]
              }
              frame #1 {
                n431 = Concatenate Strings("*RST; DZ;CL", "\n") -> (w805:string)
                n432 = VISA Write(VISA resource name=w806, write buffer=w805) -> ()  [unwired: 1 in, 3 out]
              }
            }
          }
          frame "Save" {
            w837 = 2
            w851 = "," ("string")
            w852 = "," ("string")
            w853 = ","
            w856 = "\r"
            w871 = "\r"
            w865 = "\r"
            n433 = property on="Run Button" class="Bool"("DisabledEnum"=w837) -> (error out=w842:errorcluster)  [unwired: 2 in, 1 out]
            n434 = local read "Int time"() -> (w896:dbl)
            n435 = local read "Length [um]"() -> (w892:dbl)
            n436 = local read "Width [um]"() -> (w889:dbl)
            n437 = local read "Thickness [nm]"() -> (w886:dbl)
            n438 = Get Date/Time String() -> (date string=w898:string, time string=w897:string)  [unwired: 3 in]
            n439 = property on="Stop Button" class="Bool"(error in=w842, "DisabledEnum"=w837) -> (error out=w841:errorcluster)  [unwired: 1 in, 1 out]
            n440 = Number To Decimal String(number=w896) -> (decimal integer string=w895:string)  [unwired: 1 in]
            n441 = Number To Fractional String(number=w892) -> (F-format string=w891:string)  [unwired: 3 in]
            n442 = Number To Fractional String(number=w889) -> (F-format string=w888:string)  [unwired: 3 in]
            n443 = Number To Fractional String(number=w886) -> (F-format string=w885:string)  [unwired: 3 in]
            n444 = property on="Transfer Save" class="Bool"(error in=w841, "DisabledEnum"=w837) -> (error out=w840:errorcluster)  [unwired: 1 in, 1 out]
            n445 = local read "VG stop [V]"() -> (w876:dbl)
            n446 = local read "VD [V]"() -> (w882:dbl)
            n447 = local read "VS [V]"() -> (w879:dbl)
            n448 = Number To Fractional String(number=w876) -> (F-format string=w877:string)  [unwired: 3 in]
            n449 = Number To Fractional String(number=w882) -> (F-format string=w881:string)  [unwired: 3 in]
            n450 = Number To Fractional String(number=w879) -> (F-format string=w880:string)  [unwired: 3 in]
            n451 = property on="Cancel Button" class="Bool"(error in=w840, "DisabledEnum"=w837) -> (error out=w839:errorcluster)  [unwired: 1 in, 1 out]
            n452 = Concatenate Strings(w898, w853, w897, w865, "Int Time" ("string"), w895, w853, "Length" ("string"), w891, w853, "Width" ("string"), w888, w853, "Thickness" ("string"), w885, w865) -> (w884:string)
            n453 = Concatenate Strings("VG" ("string"), w852, "ID" ("string"), w852, "IG" ("string"), w852, "IS" ("string"), w852, "Mobility" ("string"), "\r") -> (w864:string)
            n454 = Concatenate Strings("End of VG: " ("string"), w877) -> (w874:string)
            n455 = Concatenate Strings("VD: " ("string"), w881) -> (w873:string)
            n456 = Concatenate Strings("VS: " ("string"), w880) -> (w872:string)
            n457 = property on="Regime" class="Bool (strict)"(error in=w839, "DisabledEnum"=w837) -> (error out=w838:errorcluster)  [unwired: 1 in, 1 out]
            n458 = Concatenate Strings(w874, w851, w873, w851, w872, w871, w871) -> (w870:string)
            n459 = property on="Regime" class="Bool (strict)"(error in=w838, "DisabledEnum"=w837) -> ()  [unwired: 1 in, 2 out]
            n460 = local read "VG Array"() -> (w861:dbl[])
            n461 = local read "ID Array"() -> (w860:dbl[])
            n462 = local read "IG Array"() -> (w859:dbl[])
            n463 = local read "IS Array"() -> (w858:dbl[])
            n464 = local read "Mobility Array"() -> (w857:dbl[])
            n465 = Concatenate Strings(w884, w870, w864, w856, w856) -> (w855:string)
            n466 = Build Array(w861, w860, w859, w858, w857) -> (w849:dbl[][])
            n467 = Build Array(w855) -> (w854:string[])
            n468 = call-poly <vilib>:"Write Delimited Spreadsheet.vi"("format (%s)"="%s", "1D data"=w854, "delimiter (\\t)"="," ("delimiter (\\t)")) -> ("new file path (Not A Path if cancelled)"=w848:path)  [unwired: 11 in, 1 out]
            n469 = call-poly <vilib>:"Write Delimited Spreadsheet.vi"("file path (dialog if empty)"=w848, "format (%.3f)"="%e", "2D data"=w849, "append to file? (new file:F)"=TRUE, "transpose? (no:F)"=TRUE, "delimiter (\\t)"="," ("delimiter (\\t)")) -> ()  [unwired: 8 in, 2 out]
            n470 = while {
              tunnel: [w901] -> w899
              i -> [w904]
              stop <- w900 stop-if-true
              n471 = external ("Integer to Enum")(enum16{"default"}."default", w904) -> (w902:enum16{"default"})
              n472 = case shown="\"default\"" w902 {
                tunnel: [T1."Init"] -> w901
                tunnel: [TRUE] -> w900
                frame "default" {
                }
              }
            }
          }
          frame "Exit" {
            n473 = while {
              tunnel: [w930] -> w928
              i -> [w933]
              stop <- w929 stop-if-true
              n474 = external ("Integer to Enum")(enum16{"default"}."default", w933) -> (w931:enum16{"default"})
              n475 = case shown="\"default\"" w931 {
                tunnel: [T1."_Quit_"] -> w930
                tunnel: [TRUE] -> w929
                frame "default" {
                }
              }
            }
          }
        }
        n476 = Equal?(x=w484, y=T1."_Quit_") -> (x = y?=w482:bool)
      }
    }
    frame "Output" {
      # "You only can edit certain parts of the State Machine.  Right-click the While Loop and select \nUnlock Code From State Diagram to unlock the state machine from the State Diagram Editor."
      # "Right-click the border of this outer While Loop and select Edit State Diagram to open the State Diagram Editor Window."
      n477 = while {
        shift-right: [w960] -> _
        shift-left: T2."Init" -> [w961]
        stop <- w959 stop-if-true
        # "This outer Case structure contains cases that correspond to the states in the state diagram.  \nConfigure each case to reflect the actions you want each state to perform."
        n478 = case shown="\"Measuring\"" w961 {
          tunnel: [T2."_Quit_" w975 w1005 w1074 w1262 w1298 w1339] -> w960
          frame "_Quit_" {
            # "The _Quit_ case has no corresponding state on the state diagram -\nit exists to indicate to the outer While Loop when to stop executing.\nThis case is executed immediately after the case for any terminal state, \nand is the last case to execute.  Place any general clean-up code here."
          }
          frame "Init" {
            w966 = 0 ("dimension size")
            w969 = 2
            w974 = 0
            # "Each non-terminal state has at least one transition.\nThis inner While Loop and inner Case structure \ndetermine which state executes next.  The While \nLoop executes the cases in the Case structure until \nthe conditional terminal receives a TRUE value."
            n479 = property on="Start Button" class="Bool"("DisabledEnum"=w974) -> (error out=w973:errorcluster)  [unwired: 2 in, 1 out]
            n480 = property on="Hysteresis." class="Bool (strict)"(error in=w973, "DisabledEnum"=w974) -> (error out=w972:errorcluster)  [unwired: 1 in, 1 out]
            n481 = property on="Cancel Running" class="Bool"(error in=w972, "DisabledEnum"=w974) -> (error out=w971:errorcluster)  [unwired: 1 in, 1 out]
            n482 = property on="Output Stop" class="Bool"(error in=w971, "DisabledEnum"=w969) -> (error out=w970:errorcluster)  [unwired: 1 in, 1 out]
            n483 = property on="Output Save" class="Bool"(error in=w970, "DisabledEnum"=w969) -> ()  [unwired: 1 in, 2 out]
            n484 = while {
              tunnel: [w977] -> w975
              i -> [w980]
              stop <- w976 stop-if-true
              n485 = external ("Integer to Enum")(enum16{"default"}."default", w980) -> (w978:enum16{"default"})
              n486 = case shown="\"default\"" w978 {
                tunnel: [T2."Waiting"] -> w977
                tunnel: [TRUE] -> w976
                frame "default" {
                }
              }
            }
            n487 = local write "Processing Detector"(FALSE ("Processing Detector")) -> ()
            n488 = Initialize Array(w966, w966) -> (w967:i32[])
            n489 = call "Convert to Dynamic Data12"("Array"=w967) -> ("Dynamic Data Type"=w965:dynamicdata)  [unwired: 3 in]
            n490 = call "Convert to Dynamic Data13"("Array"=w967) -> ("Dynamic Data Type"=w964:dynamicdata)  [unwired: 3 in]
            n491 = call "4"("Y Input"=w964, "X Input"=w965) -> ("XY Graph"=w963:cluster{"Y":dbl[], "Y":dbl[]}[])  [unwired: 3 in, 6 out]
            n492 = local write "VD vs. IS"(w963) -> ()
            n493 = local write "VD vs. ID"(w963) -> ()
            n494 = local write "VD vs. IG"(w963) -> ()
          }
          frame "Waiting" {
            n495 = flat-sequence {
              frame #0 {
                n496 = Concatenate Strings("*RST", "\n") -> (w1024:string)
                n497 = Format Into String(format string="AIT 1,2,%d", "Int Time [Second]") -> (resulting string=w1015:string)  [unwired: 2 in, 1 out]
                n498 = VISA Write(VISA resource name="VISA resource name.", write buffer=w1024) -> (VISA resource name out=w1026:refnum<visa-resource-name>)  [unwired: 1 in, 2 out]
                n499 = Concatenate Strings("CN;FMT 12,0;AAD 1,1;AAD 2,1;AAD 3,1", "\n") -> (w1027:string)
                n500 = Concatenate Strings(w1015, "\n") -> (w1023:string)
                n501 = VISA Write(VISA resource name=w1026, write buffer=w1027) -> (VISA resource name out=w1022:refnum<visa-resource-name>)  [unwired: 1 in, 2 out]
                n502 = VISA Write(VISA resource name=w1022, write buffer=w1023) -> (VISA resource name out=w1016:refnum<visa-resource-name>)  [unwired: 1 in, 2 out]
                n503 = Format Into String(format string="DV %d,0,%f,%f ", "Source SMU no.", "VS [V].", "Source comp [V].") -> (resulting string=w1014:string)  [unwired: 2 in, 1 out]
                n504 = Concatenate Strings(w1014, "\n") -> (w1017:string)
                n505 = VISA Write(VISA resource name=w1016, write buffer=w1017) -> ()  [unwired: 1 in, 3 out]
              }
              frame #1 {
                n506 = Subtract(x="VG Stop. [V]", y="VG Start. [V]") -> (x-y=w1031:dbl)
                n507 = Divide(x=w1031, y="VG Step. [V]") -> (x/y=→"Temp":dbl)
              }
            }
            n508 = local write "Processing Detector"(FALSE ("Processing Detector")) -> ()
            n509 = while {
              tunnel: [w1034] -> w1005
              i -> [w1037]
              stop <- w1033 stop-if-true
              n510 = external ("Integer to Enum")(enum16{"Cancel", "Save", "Start", "default"}."Cancel", w1037) -> (w1035:enum16{"Cancel", "Save", "Start", "default"})
              n511 = case shown="\"Save\"" w1035 {
                tunnel: [T2."Exit" T2."Saving" T2."Measuring" T2."Waiting"] -> w1034
                tunnel: ["Cancel Running" "Output Save" "Start Button" TRUE] -> w1033
                frame "Cancel" {
                  # "Add a boolean wire\nthat is TRUE when\nthis transition is active"
                }
                frame "Save" {
                  # "Add a boolean wire\nthat is TRUE when\nthis transition is active"
                }
                frame "Start" {
                  # "Add a boolean wire\nthat is TRUE when\nthis transition is active"
                }
                frame "default" {
                }
              }
            }
          }
          frame "Measuring" {
            w1073 = 2
            n512 = property on="Start Button" class="Bool"("DisabledEnum"=w1073) -> (error out=w1071:errorcluster)  [unwired: 2 in, 1 out]
            n513 = while {
              tunnel: [w1079] -> w1067
              i -> [w1082]
              stop <- w1079 stop-if-true
              w1084 = 0
              n514 = local read "VISA resource name."() -> (w1090:refnum<visa-resource-name>)
              n515 = local read "Temp"() -> (w1078:dbl)
              n516 = Wait Until Next ms Multiple(millisecond multiple=u32 100) -> ()  [unwired: 1 out]
              n517 = Initialize Array(w1084, w1084) -> (w1085:i32[])
              n518 = Increment(x=w1078) -> (x+1=w1077:i32)
              n519 = for {
                N: w1077 -> [_]
                shift-right: [w1110] -> _
                shift-left: w1090 -> [w1106]
                shift-right: [w1107] -> w1087
                shift-left: w1085 -> [w1109]
                shift-right: [w1102] -> w1086
                shift-left: w1085 -> [w1108]
                shift-right: [w1100] -> w1088
                shift-left: w1085 -> [w1101]
                shift-right: [w1098] -> w1089
                shift-left: w1085 -> [w1099]
                tunnel: [w1092] -> w1081
                i -> [w1093]
                stop <- w1092 stop-if-true
                n520 = local read "VG Step. [V]"() -> (w1094:dbl)
                n521 = Multiply(x=w1094, y=w1093) -> (x*y=w1097:dbl)
                n522 = Subtract(x="VD stop [V]", y="VD start [V]") -> (x-y=w1116:dbl)
                n523 = Divide(x=w1116, y="VD step [V]") -> (x/y=w1113:dbl)
                n524 = call "setV.vi"("comp"="Gate comp [V].", "voltage"=w1097, "SMU"="Gate SMU no.", "VISA resource name"=w1106) -> ("VISA resource name dup"=w1105:refnum<visa-resource-name>)
                n525 = case shown="False" "Hysteresis." {
                  tunnel: w1113 -> [w1174 w1178]
                  tunnel: [w1174 w1177] -> w1095
                  frame False {
                    n526 = local write "Hysteresis LED."(FALSE ("Hysteresis LED.")) -> ()
                  }
                  frame True {
                    n527 = Multiply(x=2, y=w1178) -> (x*y=w1177:dbl)
                    "Hysteresis LED." <- TRUE ("Boolean")
                  }
                }
                n528 = Increment(x=w1095) -> (x+1=w1091:dbl)
                n529 = for {
                  N: w1091 -> [_]
                  shift-right: [w1152] -> _
                  shift-left: "VD start [V]" -> [w1141]
                  tunnel: w1113 -> [w1147]
                  tunnel: "VD step [V]" -> [w1151]
                  shift-right: [w1145] -> w1110
                  shift-left: w1105 -> [w1146]
                  shift-right: [w1139] -> w1107
                  shift-left: w1109 -> [w1143]
                  shift-right: [w1124] -> w1102
                  shift-left: w1108 -> [w1142]
                  shift-right: [w1122] -> w1100
                  shift-left: w1101 -> [w1134]
                  shift-right: [w1119] -> w1098
                  shift-left: w1099 -> [w1129]
                  tunnel: ["Output Stop"] -> w1092
                  i -> [w1118]
                  stop <- "Output Stop" stop-if-true
                  n530 = Decrement(x=w1147) -> (x-1=w1148:dbl)
                  n531 = Greater?(x=w1118, y=w1148) -> (0:w1149:bool)
                  n532 = flat-sequence {
                    tunnel: w1146 -> [w1157]
                    tunnel: w1141 -> [w1155]
                    tunnel: [w1156] -> w1137
                    tunnel: ["Drain SMU no."] -> w1136
                    tunnel: [w1160] -> w1140
                    tunnel: w1137 -> [w1161]
                    tunnel: w1136 -> [w1159]
                    tunnel: [w1158] -> w1135
                    tunnel: w1135 -> [w1165]
                    tunnel: [w1162] -> w1133
                    tunnel: [w1164] -> w1131
                    tunnel: [w1168] -> w1145
                    tunnel: w1131 -> [w1169]
                    tunnel: [w1166] -> w1128
                    frame #0 {
                      n533 = call "setV.vi"("comp"="Drain comp [V].", "voltage"=w1155, "SMU"="Drain SMU no.", "VISA resource name"=w1157) -> ("VISA resource name dup"=w1156:refnum<visa-resource-name>)
                    }
                    frame #1 {
                      n534 = call "readI.vi"("SMU"=w1159, "*VISA resource name*"=w1161) -> ("current"=w1160:dbl, "*VISA resource name*DUP"=w1158:refnum<visa-resource-name>)
                      "Drain current" <- w1160
                    }
                    frame #2 {
                      n535 = local read "Source SMU no."() -> (w1163:dbl)
                      n536 = call "readI.vi"("SMU"=w1163, "*VISA resource name*"=w1165) -> ("current"=w1162:dbl, "*VISA resource name*DUP"=w1164:refnum<visa-resource-name>)
                      "Source current" <- w1162
                    }
                    frame #3 {
                      n537 = local read "Gate SMU no."() -> (w1167:dbl)
                      n538 = call "readI.vi"("SMU"=w1167, "*VISA resource name*"=w1169) -> ("current"=w1166:dbl, "*VISA resource name*DUP"=w1168:refnum<visa-resource-name>)
                      "Gate current" <- w1166
                    }
                  }
                  n539 = case shown="True" w1149 {
                    tunnel: w1151 -> [w1170 w1171]
                    tunnel: [w1170 w1172] -> w1150
                    frame False {
                    }
                    frame True {
                      n540 = Negate(x=w1171) -> (-x=w1172:dbl)
                    }
                  }
                  n541 = Build Array (concatenate)(w1142, w1140) -> (w1124:dbl[])
                  n542 = Build Array (concatenate)(w1143, w1141) -> (w1139:dbl[])
                  n543 = Absolute Value(x=w1124) -> (abs(x)=w1123:dbl[])
                  n544 = call "Convert to Dynamic Data6"("Array"=w1139) -> ("Dynamic Data Type"=w1127:dynamicdata)  [unwired: 3 out]
                  n545 = call "Convert to Dynamic Data7"("Array"=w1123) -> ("Dynamic Data Type"=w1138:dynamicdata)  [unwired: 3 out]
                  n546 = call "?"("Y Input"=w1138, "X Input"=w1127) -> ("XY Graph"=→"VD vs. ID":cluster{"Y":dbl[], "Y":dbl[]}[])  [unwired: 3 in, 6 out]
                  n547 = Add(x=w1141, y=w1150) -> (x+y=w1152:dbl)
                  n548 = Build Array (concatenate)(w1134, w1133) -> (w1122:dbl[])
                  n549 = Absolute Value(x=w1122) -> (abs(x)=w1121:dbl[])
                  n550 = call "Convert to Dynamic Data8"("Array"=w1121) -> ("Dynamic Data Type"=w1132:dynamicdata)  [unwired: 3 in]
                  n551 = call "2"("Y Input"=w1132, "X Input"=w1127) -> ("XY Graph"=→"VD vs. IS":cluster{"Y":dbl[], "Y":dbl[]}[])  [unwired: 3 in, 6 out]
                  n552 = Build Array (concatenate)(w1129, w1128) -> (w1119:dbl[])
                  n553 = Absolute Value(x=w1119) -> (abs(x)=w1120:dbl[])
                  n554 = call "Convert to Dynamic Data9"("Array"=w1120) -> ("Dynamic Data Type"=w1126:dynamicdata)  [unwired: 3 in]
                  n555 = call "3"("Y Input"=w1126, "X Input"=w1127) -> ("XY Graph"=→"VD vs. IG":cluster{"Y":dbl[], "Y":dbl[]}[])  [unwired: 3 in, 6 out]
                  "VD." <- w1141
                }
                "Processing Detector" <- TRUE ("Processing Detector")
              }
              "VD Array." <- w1087
              "ID Array." <- w1086
              "IS Array." <- w1088
              "IG Array." <- w1089
              n556 = Decrement(x="Repeat Times.") -> (x-1=w1076:i32)
              n557 = Greater Or Equal?(x=w1082, y=w1076) -> (x >= y?=w1080:bool)
              n558 = Or(x=w1081, y=w1080) -> (x .or. y?=w1079:bool)
            }
            n559 = property on="Cancel Running" class="Bool"(error in=w1071, "DisabledEnum"=w1073) -> (error out=w1070:errorcluster)  [unwired: 1 in, 1 out]
            n560 = property on="Output Save" class="Bool"(error in=w1070, "DisabledEnum"=w1073) -> (error out=w1069:errorcluster)  [unwired: 1 in, 1 out]
            n561 = property on="Hysteresis." class="Bool (strict)"(error in=w1069, "DisabledEnum"=w1073) -> (error out=w1068:errorcluster)  [unwired: 1 in, 1 out]
            n562 = property on="Output Stop" class="Bool"(error in=w1068, "DisabledEnum"=0) -> ()  [unwired: 1 in, 2 out]
            n563 = while {
              tunnel: [w1181] -> w1074
              tunnel: w1067 -> [w1179]
              i -> [w1184]
              stop <- w1180 stop-if-true
              n564 = external ("Integer to Enum")(enum16{"Stop", "default"}."Stop", w1184) -> (w1182:enum16{"Stop", "default"})
              n565 = case shown="\"Stop\"" w1182 {
                tunnel: [T2."Stopping" T2."Measuring"] -> w1181
                tunnel: [w1206 TRUE] -> w1180
                tunnel: w1179 -> [w1206 _]
                frame "Stop" {
                  # "Add a boolean wire\nthat is TRUE when\nthis transition is active"
                }
                frame "default" {
                }
              }
            }
          }
          frame "Saving" {
            w1215 = ","
            w1232 = "\r"
            w1237 = ","
            w1261 = 2
            n566 = local read "Int Time [Second]"() -> (w1252:dbl)
            n567 = local read "VG Start. [V]"() -> (w1242:dbl)
            n568 = local read "VD stop [V]"() -> (w1248:dbl)
            n569 = local read "VD start [V]"() -> (w1250:dbl)
            n570 = local read "VD step [V]"() -> (w1245:dbl)
            n571 = local read "VG Stop. [V]"() -> (w1239:dbl)
            n572 = Get Date/Time String() -> (date string=w1256:string, time string=w1255:string)  [unwired: 3 in]
            n573 = local read "VG Step. [V]"() -> (w1238:dbl)
            n574 = Number To Fractional String(number=w1250) -> (F-format string=w1249:string)  [unwired: 3 in]
            n575 = Number To Fractional String(number=w1248) -> (F-format string=w1246:string)  [unwired: 3 in]
            n576 = Number To Fractional String(number=w1245) -> (F-format string=w1243:string)  [unwired: 3 in]
            n577 = Number To Fractional String(number=w1242) -> (F-format string=w1240:string)  [unwired: 3 in]
            n578 = Number To Decimal String(number=w1252) -> (decimal integer string=w1253:string)  [unwired: 1 in]
            n579 = Number To Fractional String(number=w1239) -> (F-format string=w1235:string)  [unwired: 3 in]
            n580 = Number To Fractional String(number=w1238) -> (F-format string=w1233:string)  [unwired: 3 in]
            n581 = property on="Start Button" class="Bool"("DisabledEnum"=w1261) -> (error out=w1260:errorcluster)  [unwired: 2 in, 1 out]
            n582 = property on="Output Stop" class="Bool"(error in=w1260, "DisabledEnum"=w1261) -> (error out=w1259:errorcluster)  [unwired: 1 in, 1 out]
            n583 = Concatenate Strings(w1256, w1237, w1255, w1232, "Int Time: ", w1253, w1237, "VD Start: ", w1249, w1237, "VD End: ", w1246, w1237, "VD Step: ", w1243, w1232, "VG Start: ", w1240, w1237, "VG Stop: ", w1235, w1237, "VG step: ", w1233, w1232) -> (w1231:string)
            n584 = property on="Cancel Running" class="Bool"(error in=w1259, "DisabledEnum"=w1261) -> (error out=w1258:errorcluster)  [unwired: 1 in, 1 out]
            n585 = Concatenate Strings("VD" ("string"), w1215, "ID" ("string"), w1215, "IS" ("string"), w1215, "IG" ("string"), "\r") -> (w1210:string)
            n586 = property on="Output Save" class="Bool"(error in=w1258, "DisabledEnum"=w1261) -> (error out=w1257:errorcluster)  [unwired: 1 in, 1 out]
            n587 = local read "IG Array."() -> (w1211:dbl[])
            n588 = local read "ID Array."() -> (w1223:dbl[])
            n589 = local read "IS Array."() -> (w1212:dbl[])
            n590 = local read "VD Array."() -> (w1224:dbl[])
            n591 = Concatenate Strings(w1231, w1210) -> (w1228:string)
            n592 = property on="Hysteresis." class="Bool (strict)"(error in=w1257, "DisabledEnum"=w1261) -> ()  [unwired: 1 in, 2 out]
            n593 = Build Array(w1228) -> (w1227:string[])
            n594 = Build Array(w1224, w1223, w1212, w1211) -> (w1222:dbl[][])
            n595 = call-poly <vilib>:"Write Delimited Spreadsheet.vi"("format (%s)"="%s", "1D data"=w1227, "delimiter (\\t)"="," ("delimiter (\\t)")) -> ("new file path (Not A Path if cancelled)"=w1217:path)  [unwired: 11 in, 1 out]
            n596 = call-poly <vilib>:"Write Delimited Spreadsheet.vi"("file path (dialog if empty)"=w1217, "format (%.3f)"="%e", "2D data"=w1222, "append to file? (new file:F)"=TRUE, "transpose? (no:F)"=TRUE, "delimiter (\\t)"="," ("delimiter (\\t)")) -> ()  [unwired: 8 in, 2 out]
            n597 = while {
              tunnel: [w1264] -> w1262
              i -> [w1267]
              stop <- w1263 stop-if-true
              n598 = external ("Integer to Enum")(enum16{"default"}."default", w1267) -> (w1265:enum16{"default"})
              n599 = case shown="\"default\"" w1265 {
                tunnel: [T2."Init"] -> w1264
                tunnel: [TRUE] -> w1263
                frame "default" {
                }
              }
            }
          }
          frame "Stopping" {
            w1297 = 0
            n600 = property on="Start Button" class="Bool"("DisabledEnum"=w1297) -> (error out=w1295:errorcluster)  [unwired: 2 in, 1 out]
            n601 = property on="Cancel Running" class="Bool"(error in=w1295, "DisabledEnum"=w1297) -> (error out=w1294:errorcluster)  [unwired: 1 in, 1 out]
            n602 = property on="Output Save" class="Bool"(error in=w1294, "DisabledEnum"=w1297) -> (error out=w1293:errorcluster)  [unwired: 1 in, 1 out]
            n603 = while {
              tunnel: [w1312] -> w1298
              i -> [w1315]
              stop <- w1311 stop-if-true
              n604 = external ("Integer to Enum")(enum16{"default"}."default", w1315) -> (w1313:enum16{"default"})
              n605 = case shown="\"default\"" w1313 {
                tunnel: [T2."Waiting"] -> w1312
                tunnel: [TRUE] -> w1311
                frame "default" {
                }
              }
            }
            n606 = property on="Hysteresis." class="Bool (strict)"(error in=w1293, "DisabledEnum"=w1297) -> (error out=w1292:errorcluster)  [unwired: 1 in, 1 out]
            n607 = property on="Output Stop" class="Bool"(error in=w1292, "DisabledEnum"=2) -> ()  [unwired: 1 in, 2 out]
            n608 = flat-sequence {
              tunnel: [w1299] -> w1291
              tunnel: w1291 -> [w1307]
              frame #0 {
                w1300 = 0.001
                w1304 = 0
                n609 = local read "VISA resource name."() -> (w1299:refnum<visa-resource-name>)
                n610 = call "setV.vi"("comp"=w1300, "voltage"=w1304, "SMU"=1, "VISA resource name"=w1299) -> ("VISA resource name dup"=w1302:refnum<visa-resource-name>)
                n611 = call "setV.vi"("comp"=w1300, "voltage"=w1304, "SMU"=2, "VISA resource name"=w1302) -> ("VISA resource name dup"=w1303:refnum<visa-resource-name>)
                n612 = call "setV.vi"("comp"=w1300, "voltage"=w1304, "SMU"=3, "VISA resource name"=w1303) -> ()  [unwired: 1 out]
              }
              frame #1 {
                n613 = Concatenate Strings("DZ;CL", "\n") -> (w1310:string)
                n614 = VISA Write(VISA resource name=w1307, write buffer=w1310) -> ()  [unwired: 1 in, 3 out]
              }
            }
          }
          frame "Exit" {
            n615 = while {
              tunnel: [w1341] -> w1339
              i -> [w1344]
              stop <- w1340 stop-if-true
              n616 = external ("Integer to Enum")(enum16{"default"}."default", w1344) -> (w1342:enum16{"default"})
              n617 = case shown="\"default\"" w1342 {
                tunnel: [T2."_Quit_"] -> w1341
                tunnel: [TRUE] -> w1340
                frame "default" {
                }
              }
            }
          }
        }
        n618 = Equal?(x=w961, y=T2."_Quit_") -> (x = y?=w959:bool)
      }
    }
  }
